vi "SpectrometerSpinCoater_v12.vi"() -> ()   [LabVIEW 2020]
uses:
  TypDef/TabControl_InSitu_Type.ctl
  <instrlib>/Classes/CCD/Abstract_CCD/Abstract_CCD.lvclass
  <instrlib>/Classes/SpinCoater/SpinCoater.lvclass
  TypDef/DeviceQueue_TypeDef.ctl
  TypDef/DeviceQueue_Action.ctl
  TypDef/TabControl.ctl
  TypDef/DataQueue_TypeDef.ctl
  TypDef/DataQueue_Action.ctl
  <vilib>/Utility/error.llb/DialogType.ctl
  <instrlib>/Classes/CCD/Avantes/Avantes.lvclass
  C:/Program Files/National Instruments/LabVIEW 2020/instr.lib/Classes/CCD/Abstract_CCD/Abstract_CCD.lvclass
  <vilib>/Analysis/baseanly.llb/A x Vector.vi
  <vilib>/Analysis/NI_AALBase.lvlib
panel:
  out "x-y":dbl
  in  "Reference\nValue":dbl
  out "WL-Det\nPos":i32
  in  "Motor_ShortStop":bool
  out "UpperWLLimit":i32=713
  out "LowerWLLimit":i32=149
  out "Nr After Spin":u16
  out "Action":string="TimeOut"
  out "Time.spin":refnum<file>
  out "Meas.spin":refnum<file>
  out "Arduino":bool
  out "NKT":bool
  out "Spectromter":bool
  in  "Abort Button":bool
  in  "Stop Button":bool=TRUE
  in  "Tab Control":T1(tab)
  in  "Trim\nSpec":bool=TRUE
  in  "Wl \nUp":dbl[unit]=7.102291259765626e-07
  in  "Wl \nLow":dbl[unit]=3.7998095703125003e-07
  in  "Frames for Ref/Dark":dbl=10000.0
  in  "Shutter Toggle":bool
  in  "Program Spin Coater":T2(array[cluster])=[{"Speed (rpm)"=1500.0, "Time (s)"=10.0, "Acc (rpm/s)"=0.0}]
  in  "Spectra Count":u16
  in  "Measure_MeasureSpectrum":bool
  out "Overall Time":dbl=13.0
  in  "Frames":i32=34211
  in  "StartMeasurement_Button":bool
  in  "Measure_Preview":bool
  out "Measure_Graph":T3(graph) caption="XY Graph"
  in  "Measure_FramesSpectrometer":dbl=200.0 caption="Frames for Spectrometer"
  in  "StartSpin_Button":bool
  in  "Record RefSpec":bool
  in  "Measure:\nRecord_Darkspec":bool
  in  "Measure_Comments":string="Just for testing" caption="Comments"
  in  "Measure_FileName":string="newlineShort" caption="File Name"
  in  "Measure_SavePath":path=path "C:/Users/Cerberus/Desktop/Test/v12Test" caption="Save Path"
  out "Measure_FrameRate":dbl[unit]=2631.5791015625 caption="Frame Rate"
  in  "Measure_IntegrationTime":dbl[unit]=3e-05 caption="Integration Time"
  in  "Tab Control SpinType":T4=enum."Short"
  in  "Seconds after Spin":dbl[unit]=3.0
  in  "Calculate Frames_Normal":bool=TRUE caption="Calculate Frames"
  in  "periodic time":dbl[unit]=2.0
  in  "Duration after":dbl[unit]
  in  "Spin at end":bool
  in  "Seconds to Spin_Normal":dbl[unit]=5.0 caption="Seconds to Spin"
  in  "Threshold":dbl=0.3
  in  "Time Detect":dbl[unit]=2.0
  in  "Seconds to Spin_Short":dbl[unit]=5.0 caption="Seconds to Spin"
  in  "Spin Time":dbl[unit]=2.0
  in  "Calculate Frames_Short":bool=TRUE caption="Calculate Frames"
  in  "Wavelenght Detect":dbl[unit]=6.000000000000001e-07
  out "SS_StepsLeft":dbl
  out "SS_TimePrediction":dbl[unit]=-6.0
  out "Horizontal Progress Bar":u8(slide) scale=0.0..100.0
  in  "SpectralStability:\nRecord_Darkspec":bool
  in  "SpectralStability_Record":bool
  in  "SpectralStability_\nMeasurementNumber":u32 caption="Measurement Number"
  in  "SpectralStability_Duration":dbl[unit] caption="Duration"
  in  "Duration/Times":bool
  in  "SpectralStability_\nPeriodicTime":dbl[unit] caption="Periodic Time"
  in  "SpectralStability_MeasureSpectrum":bool
  in  "SpectralStability_Preview":bool
  out "SpectralStability_Graph":T3(graph) caption="XY Graph"
  in  "SpectralStability_FramesSpectrometer":dbl=200.0 caption="Frames for Spectrometer"
  in  "SpectralStability_Comments":string="Just for testing" caption="Comments"
  in  "SpectralStability_FileName":string="TestingAfter" caption="File Name"
  in  "SpectralStability_SavePath":path=path "C:/Users/Timo/Desktop/Test/180824" caption="Save Path"
  out "SpectralStability_FrameRate":dbl[unit]=2631.5791015625 caption="Frame Rate"
  in  "SpectralStability_IntegrationTime":dbl[unit]=3e-05 caption="Integration Time"
  in  "Shutter Close":bool
  in  "Shutter Open":bool
  in  "SHUTTER DEBUG":bool
  in  "Shutter Position":u16=1000
  in  "Dividider Get Spectra":u32=1 min=1
  in  "Automatically \nadjust count":bool=TRUE
  in  "Reset Count\nafter Spin Coating":bool=TRUE
  in  "ESC_Speed":dbl
  in  "ESC_Milliseconds":dbl
  in  "ESC DEBUG":bool
  in  "Port Arduino":refnum<visa-resource-name>="COM7"
  out "Error Arduino":bool caption="Error"
  in  "Init_Arduino":bool caption="Init"
  out "Caption_Settings_Arduino":string="Arduino"
  out "Caption_Settings_NKT":string="NKT Laser"
  out "Error_Spectromter":bool caption="Error"
  in  "Init_Spectrometer":bool caption="Init"
  out "Caption_Settings_Spectrometer":string="Spectromter"
  # "Speed (rpm)   Time (s)        Acceleration \n                                               (rpm/s)"
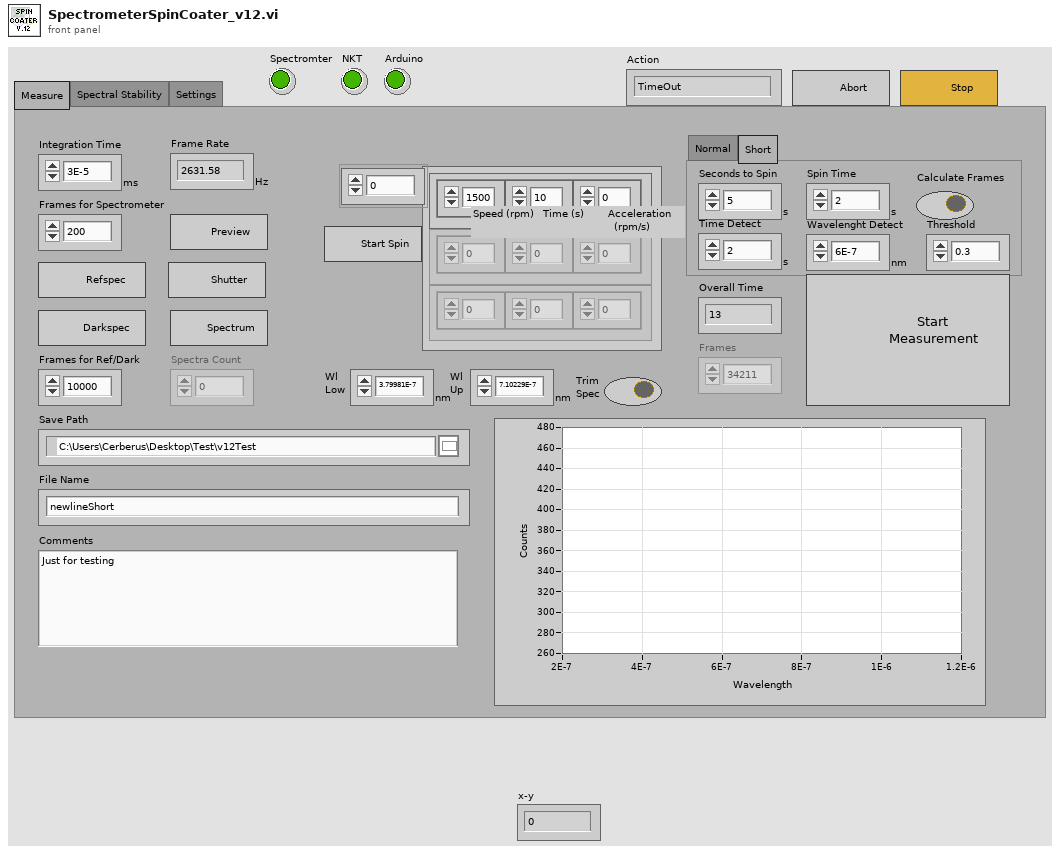
[diagram p1: front panel]
types:
  T1 = enum32{"Measure", "Spectral Stability", "Settings"}
  T2 = cluster{"Speed (rpm)":dbl, "Time (s)":dbl, "Acc (rpm/s)":dbl}[]
  T3 = cluster{"Wavlength":dbl[unit][], "Image":dbl[]}[]
  T4 = typedef "TabControl_InSitu_Type.ctl" = enum32{"Normal", "Short"}
  T5 = cluster{"Dark":cluster{"Image":dbl[][][], "Frame Size":cluster{"F":i32, "Y":i32, "X":i32}}[], "Ref":cluster{"Image":dbl[][][], "Frame Size":cluster{"F":i32, "Y":i32, "X":i32}}[], "Wavlength":dbl[unit][], "Wavlength Trim":dbl[unit][], "spec":dbl[][]}
  T6 = cluster{"Abstract_CCD.lvclass":refnum<class "Abstract_CCD.lvclass">, "SpinCoater.lvclass":refnum<class "SpinCoater.lvclass">}
  T7 = enum8{"Enabled", "Disabled", "Disabled and Grayed Out"}
  T8 = typedef "DataQueue_TypeDef.ctl" = cluster{"QueueAction":T9, "Data":cluster{"Image":dbl[][][], "Frame Size":cluster{"F":i32, "Y":i32, "X":i32}}[], "Data_Raw":cluster{"Image":dbl[][][], "Frame Size":cluster{"F":i32, "Y":i32, "X":i32}}[], "Data_Dark":cluster{"Image":dbl[][][], "Frame Size":cluster{"F":i32, "Y":i32, "X":i32}}[], "Data_Ref":cluster{"Image":dbl[][][], "Frame Size":cluster{"F":i32, "Y":i32, "X":i32}}[], "Device Information":string[], "Numeric Control":dbl, "Boolean":bool, "Wavelength":dbl[unit][], "Time":dbl[], "Time Stamp":timestamp, "Numeric Control 2":dbl, "TabControl":T10, "Numeric Control 3":dbl}
  T9 = typedef "DataQueue_Action.ctl" = enum16{"TimeOut", "Close_Program", "Abort", "Stop_Measurement", "Measure_InSituSpinCoating", "Measure_InSituSpinCoating_Short", "Measure_Spectrum", "Measure_SpectrumAdvanced", "Measure_SpectralStability", "Save_InSitu", "Save_SpectralStability", "Set_Ref", "Set_Dark", "Set_Wavelength", "Spectrometer_Measure", "Spectrometer_Preview", "Transfer_Settings", "Change_TrimSettings"}
  T10 = typedef "TabControl.ctl" = enum16{"Measure", "Spectral Stability", "Settings"}
  T11 = typedef "DeviceQueue_TypeDef.ctl" = cluster{"QueueAction":T12, "Numeric 1":dbl, "Numeric 2":dbl, "Boolean 1":bool, "Boolean 2":bool, "Spin Program":dbl[][], "Spin Prg v07":cluster{"Speed (rpm)":dbl, "Time (s)":dbl, "Acc (rpm/s)":dbl}[], "Time Stamp":timestamp, "TabControl":T10}
  T12 = typedef "DeviceQueue_Action.ctl" = enum16{"TimeOut", "Wait", "Close_Program", "Abort", "Spectrometer_Init", "Spectrometer_Close", "Spectrometer_DeviceInformation", "Spectrometer_Measure", "Spectrometer_MeasureAdvanced", "Spectrometer_Preview", "Spectrometer_Abort", "Spectrometer_StartMeasurement", "Spectrometer_GetData", "Spectrometer_GetData_Short", "Spectrometer_StopMeasurement", "Spectrometer_SetIntegrationTime", "Spectrometer_SetFrames", "Spectrometer_SetDarkspec", "Spectrometer_SetReference", "Spectrometer_SetTriggerMode", "Laser_Init", "Laser_Close", "Arduino_Init", "Arduino_Close", "Arduino_LoadProgram", "Arduino_StartProgram", "Arduino_SetSpeed", "Arduino_SetMillis", "Arduino_StopSpin", "Arduino_ShortStop", "Arduino_Shutter_SetPosition", "Arduino_Shutter_Close", "Arduino_Shutter_Open", "Measure_InSitu", "Measure_Spectrum", "Measure_InSituAdvanced", "Measure_InSituAdvanced_Short", "Measure_SpectralStability", "Measure_Stop"}
  T13 = enum16{"open", "replace", "create", "open or create", "replace or create", "replace or create with confirmation"}
  T14 = cluster{"Image":dbl[][][], "Frame Size":cluster{"F":i32, "Y":i32, "X":i32}}[]
  T15 = cluster{"Image":dbl[][][], "Frame Size":cluster{"F":i32, "Y":i32, "X":i32}}
  T16 = cluster{"Wavlength":dbl[unit][], "A x Vector":dbl[]}
  T17 = cluster{"Wavlength":dbl[unit][], "A x Vector":dbl[]}[]
  T18 = cluster{u16[][][], u16[][][], dbl[], "Numeric Control":dbl, "Numeric Control 2":dbl}
  T19 = typedef "DialogType.ctl" = u16
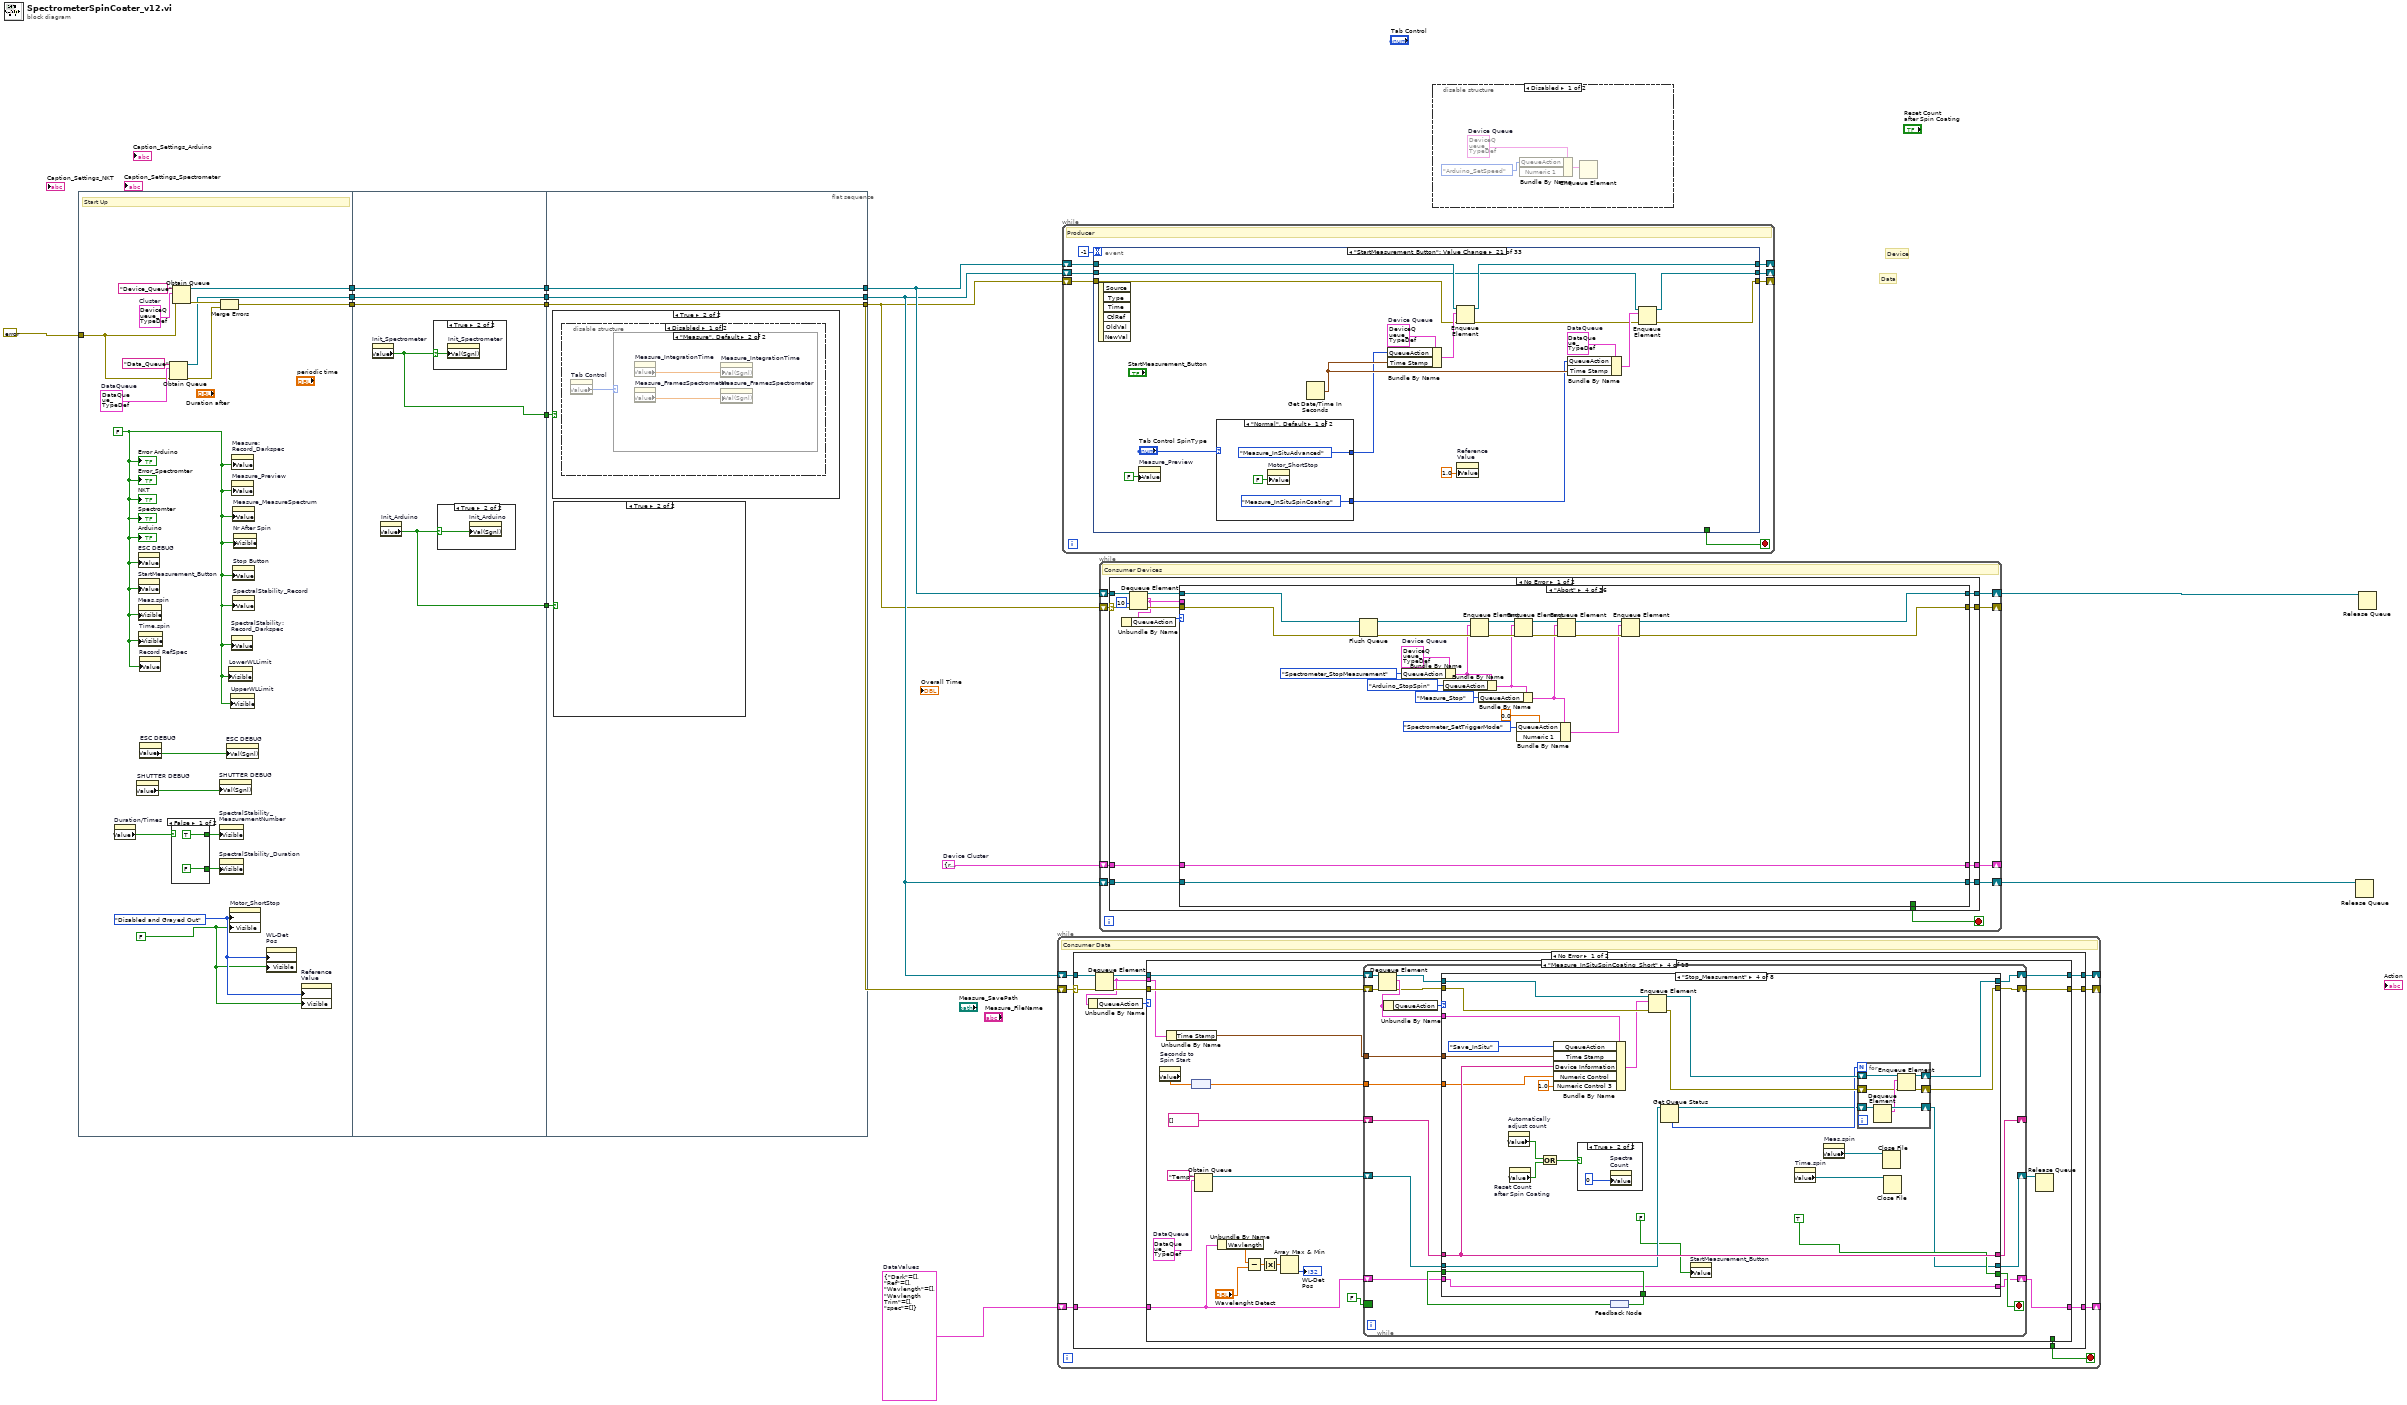
[diagram p0: block diagram]
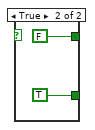
[diagram p3: hidden frame]
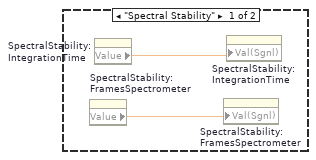
[diagram p8: hidden frame]
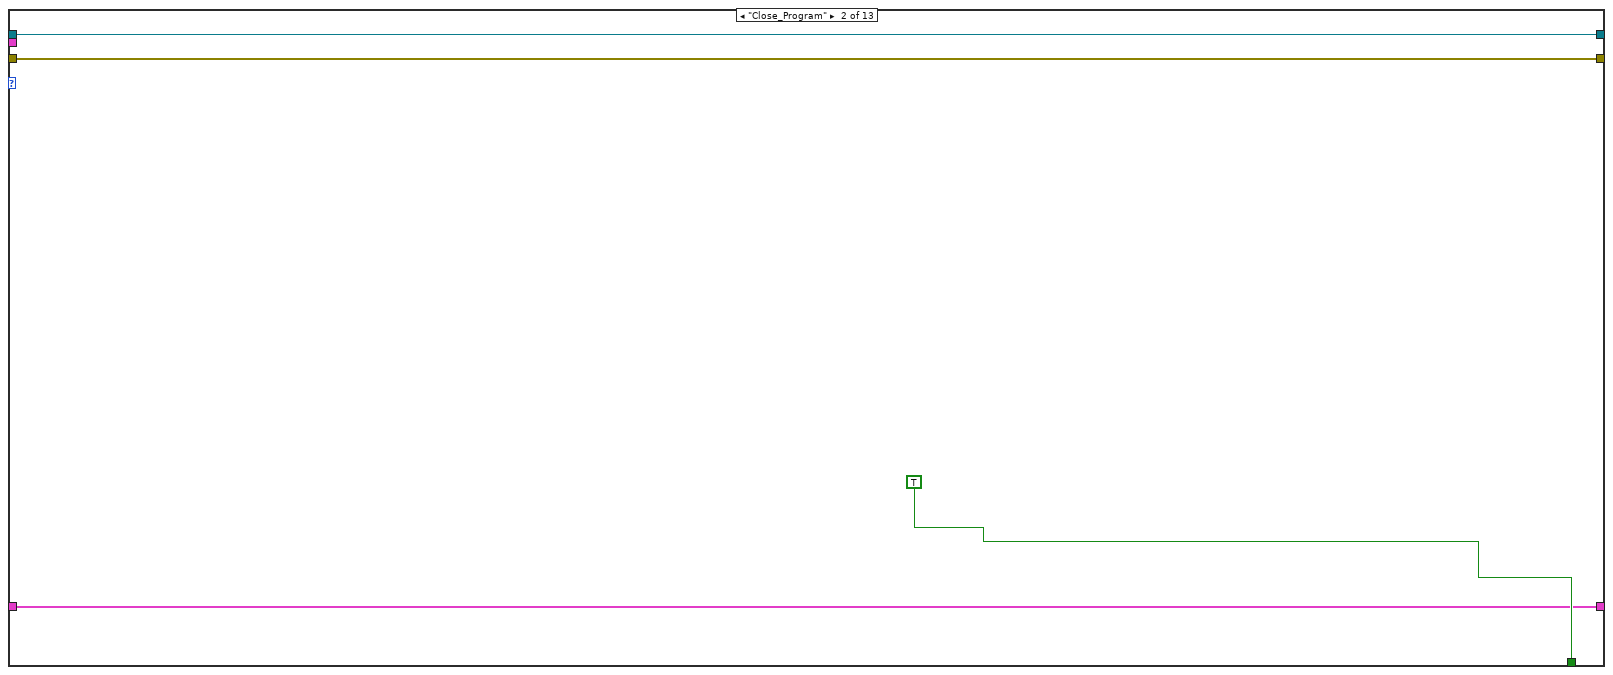
[diagram p11: hidden frame]
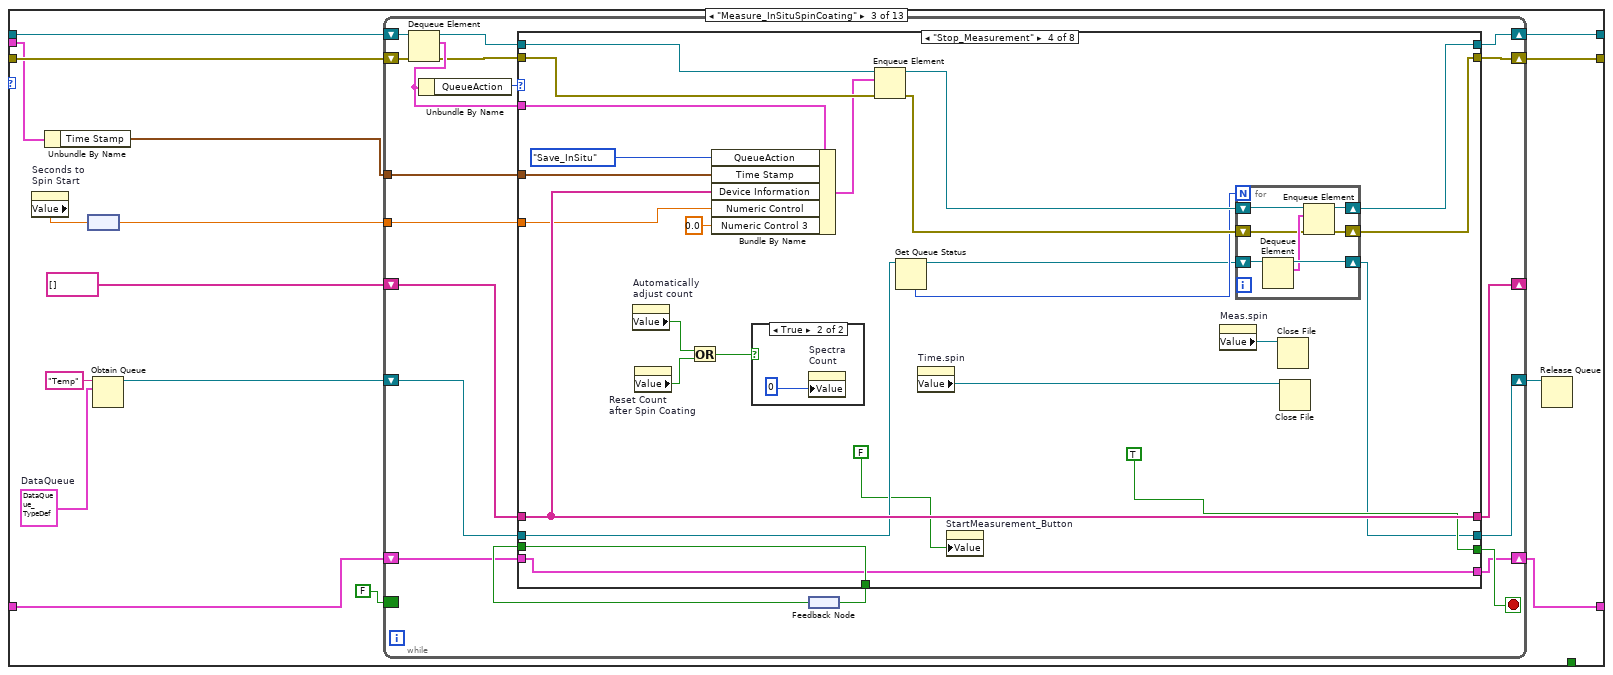
[diagram p12: hidden frame]
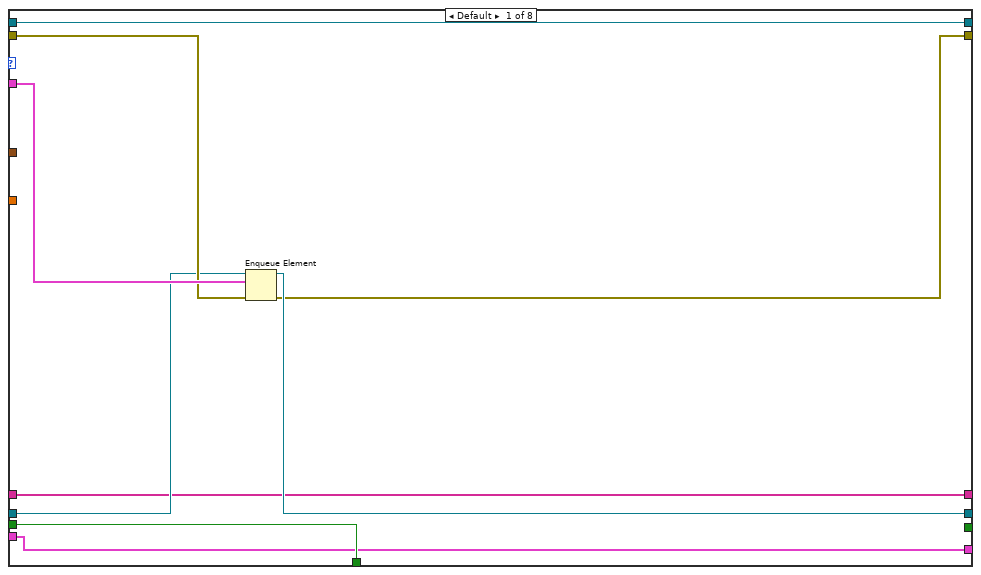
[diagram p13: hidden frame]
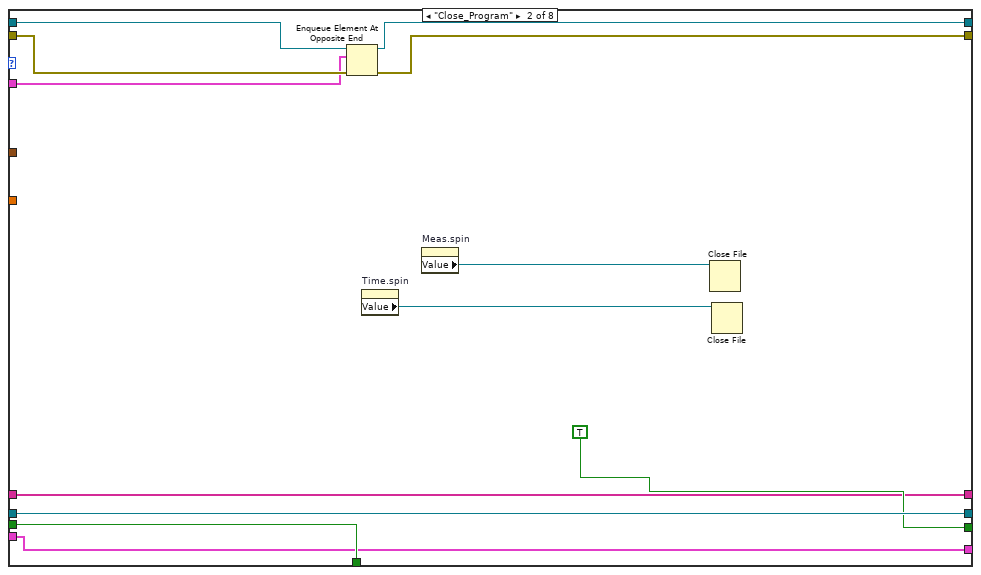
[diagram p14: hidden frame]
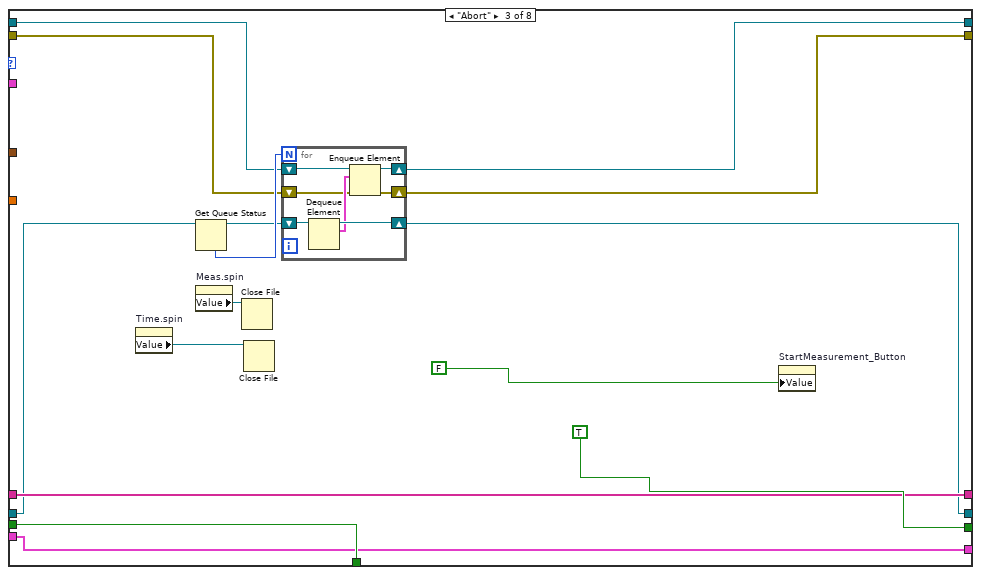
[diagram p15: hidden frame]
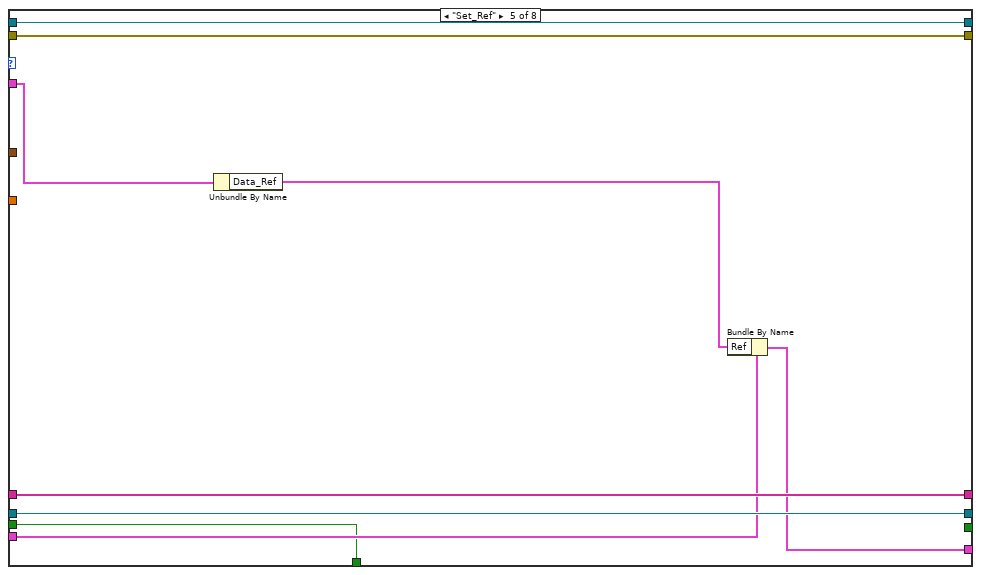
[diagram p17: hidden frame]
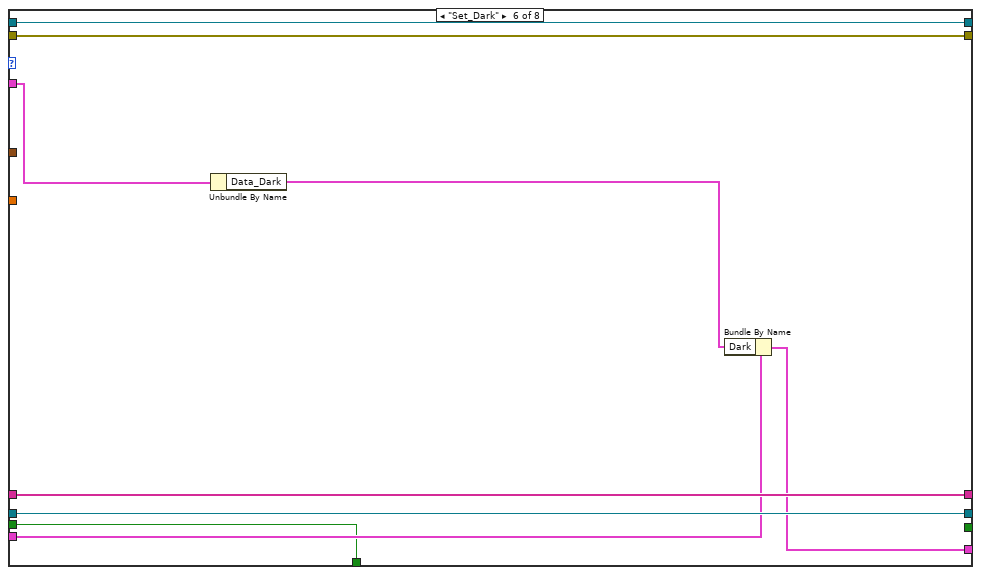
[diagram p18: hidden frame]
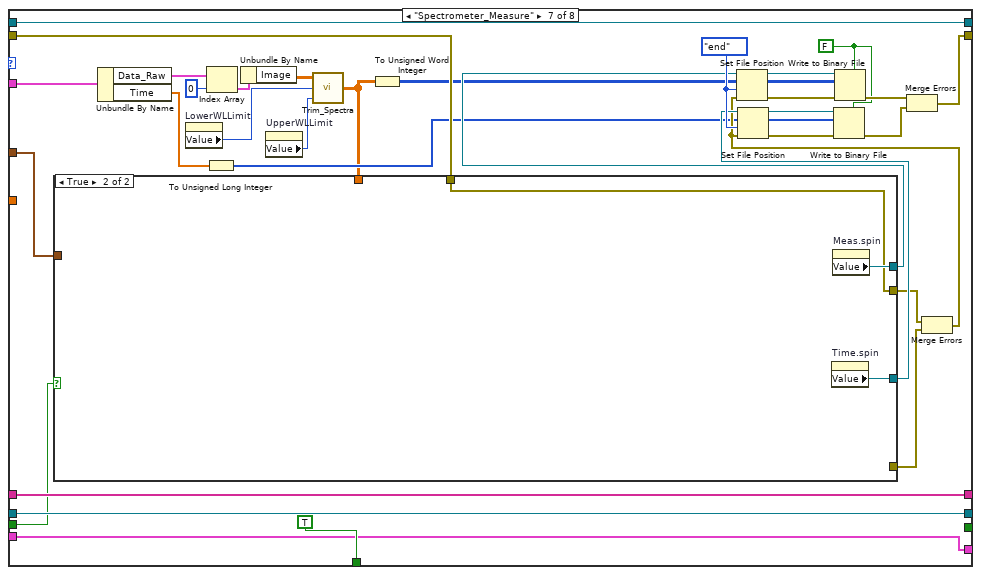
[diagram p19: hidden frame]
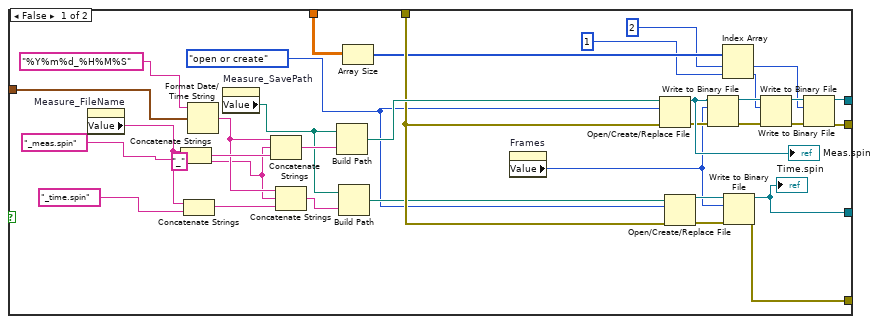
[diagram p20: hidden frame]
diagram:
  w7 = T5 {"Dark"=[], "Ref"=[], "Wavlength"=[], "Wavlength Trim"=[], "spec"=[]}  # DataValues
  w11 = T6 {"Abstract_CCD.lvclass"=refnum, "SpinCoater.lvclass"=refnum}  # Device Cluster
  # "Data"
  # "Device"
  n1 = flat-sequence {
    tunnel: errorcluster {"status"=FALSE, "code"=0, "source"=""} ("error constant") -> [w29]
    tunnel: [w32] -> w15
    tunnel: [w26] -> w14
    tunnel: [w25] -> w13
    tunnel: w15 -> [w43]
    tunnel: w14 -> [w42]
    tunnel: w13 -> [w41]
    tunnel: [w43] -> w6
    tunnel: [w42] -> w5
    tunnel: [w41] -> w4
    tunnel: [w40] -> w3
    tunnel: [w39] -> w2
    tunnel: [w48] -> w1
    tunnel: [w49] -> w8
    tunnel: [w50] -> w12
    tunnel: w6 -> [w50]
    tunnel: w5 -> [w49]
    tunnel: w4 -> [w48]
    tunnel: w3 -> [w47]
    tunnel: w2 -> [w46]
    frame #0 {
      w18 = T7."Disabled and Grayed Out" ("Disabled")
      w17 = FALSE ("Visible")
      w30 = T8 {"QueueAction"=enum."TimeOut", "Data"=[], "Data_Raw"=[], "Data_Dark"=[], "Data_Ref"=[], "Device Information"=[], "Numeric Control"=0.0, "Boolean"=FALSE, "Wavelength"=[], "Time"=[], "Time Stamp"=timestamp(0 s since 1904-01-01), "Numeric Control 2"=0.0, "TabControl"=enum."Measure", "Numeric Control 3"=0.0}  # DataQueue
      w33 = T11 {"QueueAction"=enum."TimeOut", "Numeric 1"=0.0, "Numeric 2"=0.0, "Boolean 1"=FALSE, "Boolean 2"=FALSE, "Spin Program"=[], "Spin Prg v07"=[], "Time Stamp"=timestamp(0 s since 1904-01-01), "TabControl"=enum."Measure"}  # Cluster
      w19 = FALSE ("Error Arduino")
      # "Start Up"
      n2 = property on="Duration/Times" class="Bool (strict)"() -> ("Value"=w21:bool)  [unwired: 2 in, 2 out]
      n3 = property on="SHUTTER DEBUG" class="Bool (strict)"() -> ("Value"=w20:bool)  [unwired: 2 in, 2 out]
      n4 = property on="ESC DEBUG" class="Bool (strict)"("Value"=w19) -> ()  [unwired: 2 in, 2 out]
      n5 = property on="StartMeasurement_Button" class="Bool (strict)"("Value"=w19) -> ()  [unwired: 2 in, 2 out]
      n6 = property on="Meas.spin" class="Ref (strict)"("Visible"=w19) -> ()  [unwired: 2 in, 2 out]
      n7 = property on="Time.spin" class="Ref (strict)"("Visible"=w19) -> ()  [unwired: 2 in, 2 out]
      n8 = property on="Record RefSpec" class="Bool (strict)"("Value"=w19) -> ()  [unwired: 2 in, 2 out]
      n9 = property on="ESC DEBUG" class="Bool (strict)"() -> ("Value"=w24:bool)  [unwired: 2 in, 2 out]
      n10 = Obtain Queue(name (unnamed)="Data_Queue", element data type=w30, error in (no error)=w29) -> (queue out=w26:refnum<queue>, error out=w27:errorcluster)  [unwired: 2 in, 1 out]
      n11 = case shown="False" w21 {
        tunnel: [FALSE TRUE] -> w23
        tunnel: [TRUE FALSE] -> w22
        frame False {
        }
        frame True {
        }
      }
      n12 = Obtain Queue(name (unnamed)="Device_Queue", element data type=w33, error in (no error)=w29) -> (queue out=w32:refnum<queue>, error out=w28:errorcluster)  [unwired: 2 in, 1 out]
      n13 = property on="SHUTTER DEBUG" class="Bool (strict)"("Val(Sgnl)"=w20) -> ()  [unwired: 2 in, 2 out]
      n14 = property on="SpectralStability_\nMeasurementNumber" class="DigNum (strict)"("Visible"=w22) -> ()  [unwired: 2 in, 2 out]
      n15 = property on="SpectralStability_Duration" class="DigNum (strict)"("Visible"=w23) -> ()  [unwired: 2 in, 2 out]
      n16 = Merge Errors(w28, w27) -> (w25:errorcluster)
      n17 = property on="ESC DEBUG" class="Bool (strict)"("Val(Sgnl)"=w24) -> ()  [unwired: 2 in, 2 out]
      n18 = property on="LowerWLLimit" class="DigNum (strict)"("Visible"=w19) -> ()  [unwired: 2 in, 2 out]
      n19 = property on="Motor_ShortStop" class="Bool (strict)"("DisabledEnum"=w18, "Visible"=w17) -> ()  [unwired: 2 in, 2 out]
      n20 = property on="UpperWLLimit" class="DigNum (strict)"("Visible"=w19) -> ()  [unwired: 2 in, 2 out]
      n21 = property on="SpectralStability:\nRecord_Darkspec" class="Bool (strict)"("Value"=w19) -> ()  [unwired: 2 in, 2 out]
      n22 = property on="Measure:\nRecord_Darkspec" class="Bool (strict)"("Value"=w19) -> ()  [unwired: 2 in, 2 out]
      n23 = property on="Measure_Preview" class="Bool (strict)"("Value"=w19) -> ()  [unwired: 2 in, 2 out]
      n24 = property on="Measure_MeasureSpectrum" class="Bool (strict)"("Value"=w19) -> ()  [unwired: 2 in, 2 out]
      n25 = property on="Stop Button" class="Bool (strict)"("Value"=w19) -> ()  [unwired: 2 in, 2 out]
      n26 = property on="SpectralStability_Record" class="Bool (strict)"("Value"=w19) -> ()  [unwired: 2 in, 2 out]
      n27 = property on="Nr After Spin" class="DigNum (strict)"("Visible"=w19) -> ()  [unwired: 2 in, 2 out]
      n28 = property on="WL-Det\nPos" class="DigNum (strict)"("DisabledEnum"=w18, "Visible"=w17) -> ()  [unwired: 2 in, 2 out]
      n29 = property on="Reference\nValue" class="DigNum (strict)"("DisabledEnum"=w18, "Visible"=w17) -> ()  [unwired: 2 in, 2 out]
      "Error_Spectromter" <- w19
      "Error Arduino" <- w19
      "Spectromter" <- w19
      "NKT" <- w19
      "Arduino" <- w19
    }
    frame #1 {
      n30 = property on="Init_Spectrometer" class="Bool (strict)"() -> ("Value"=w40:bool)  [unwired: 2 in, 2 out]
      n31 = property on="Init_Arduino" class="Bool (strict)"() -> ("Value"=w39:bool)  [unwired: 2 in, 2 out]
      n32 = case shown="True" w40 {
        selector: w40 -> [_ w45]
        frame False {
        }
        frame True {
          n33 = property on="Init_Spectrometer" class="Bool (strict)"("Val(Sgnl)"=w45) -> ()  [unwired: 2 in, 2 out]
        }
      }
      n34 = case shown="True" w39 {
        selector: w39 -> [_ w44]
        frame False {
        }
        frame True {
          n35 = property on="Init_Arduino" class="Bool (strict)"("Val(Sgnl)"=w44) -> ()  [unwired: 2 in, 2 out]
        }
      }
    }
    frame #2 {
      n36 = case shown="True" w47 {
        frame False {
        }
        frame True {
          n37 = disable-structure shown="Disabled" {
            frame Disabled {
              n38 = property on="Tab Control" class="TabCtl (strict)"() -> ("Value"=w51:T1)  [unwired: 2 in, 2 out]
              n39 = case shown="\"Measure\", Default" w51 {
                frame "Spectral Stability" {
                  n40 = property on="SpectralStability:\nFramesSpectrometer" class="DigNum (strict)"() -> ("Value"=w52:dbl)  [unwired: 2 in, 2 out]
                  n41 = property on="SpectralStability:\nIntegrationTime" class="DigNum (strict)"() -> ("Value"=w53:dbl[unit])  [unwired: 2 in, 2 out]
                  n42 = property on="SpectralStability:\nFramesSpectrometer" class="DigNum (strict)"("Val(Sgnl)"=w52) -> ()  [unwired: 2 in, 2 out]
                  n43 = property on="SpectralStability:\nIntegrationTime" class="DigNum (strict)"("Val(Sgnl)"=w53) -> ()  [unwired: 2 in, 2 out]
                }
                frame "Measure", Default {
                  n44 = property on="Measure_IntegrationTime" class="DigNum (strict)"() -> ("Value"=w54:dbl[unit])  [unwired: 2 in, 2 out]
                  n45 = property on="Measure_FramesSpectrometer" class="DigNum (strict)"() -> ("Value"=w55:dbl)  [unwired: 2 in, 2 out]
                  n46 = property on="Measure_IntegrationTime" class="DigNum (strict)"("Val(Sgnl)"=w54) -> ()  [unwired: 2 in, 2 out]
                  n47 = property on="Measure_FramesSpectrometer" class="DigNum (strict)"("Val(Sgnl)"=w55) -> ()  [unwired: 2 in, 2 out]
                }
              }
            }
            frame Enabled {
            }
          }
        }
      }
      n48 = case shown="True" w46 {
        frame False {
        }
        frame True {
        }
      }
    }
  }
  n49 = while {
    shift-right: [w56] -> _
    shift-left: w1 -> [w62]
    shift-right: [w57] -> _
    shift-left: w8 -> [w61]
    shift-right: [w58] -> _
    shift-left: w7 -> [w60]
    stop <- w59 stop-if-true
    # "Consumer Data"
    n50 = case shown="No Error" w62 {
      selector: w62 -> [w73 w1049]
      tunnel: w61 -> [w72 w1050]
      tunnel: w60 -> [w70 w1047]
      tunnel: [w69 _] -> w59
      tunnel: [w68 w1047] -> w58
      tunnel: [w67 w1050] -> w57
      tunnel: [w65 w1048] -> w56
      frame No Error {
        n51 = Dequeue Element(queue=w72, error in (no error)=w73) -> (queue out=w66:refnum<queue>, element=w63:T8, error out=w64:errorcluster)  [unwired: 1 in, 1 out]
        n52 = Unbundle By Name(w63) -> ("QueueAction"=w71:T9)
        n53 = case shown="\"Measure_InSituSpinCoating_Short\"" w71 {
          tunnel: w70 -> [w74 w79 w81 w294 w502 w607 w709 w928 w965 w974 w997 w1010 w1017]
          tunnel: [_ TRUE _ _ _ _ _ _ _ _ _ _ _] -> w69
          tunnel: [w74 w79 w83 w296 w502 w607 w700 w928 w969 w988 w996 w1010 w1016] -> w68
          tunnel: [w76 w78 w96 w309 w508 w613 w693 w950 w970 w989 w993 w1012 w1023] -> w67
          tunnel: w66 -> [w76 w78 w94 w307 w509 w614 w704 w950 w970 w989 w993 w1012 w1023]
          tunnel: [w75 w77 w95 w308 w507 w612 w694 w949 w971 w990 w994 w1011 w1020] -> w65
          tunnel: w64 -> [w75 w77 w93 w306 w510 w615 w703 w949 w971 w990 w994 w1011 w1020]
          tunnel: w63 -> [_ _ w88 w301 _ _ w696 w940 w972 w991 w995 w1001 w1022]
          frame "TimeOut", Default {
          }
          frame "Close_Program" {
          }
          frame "Measure_InSituSpinCoating" {
            w91 = T8 {"QueueAction"=enum."TimeOut", "Data"=[], "Data_Raw"=[], "Data_Dark"=[], "Data_Ref"=[], "Device Information"=[], "Numeric Control"=0.0, "Boolean"=FALSE, "Wavelength"=[], "Time"=[], "Time Stamp"=timestamp(0 s since 1904-01-01), "Numeric Control 2"=0.0, "TabControl"=enum."Measure", "Numeric Control 3"=0.0}  # DataQueue
            n54 = property on="Seconds to\nSpin Start" class="DigNum (strict)"() -> ("Value"=w85:dbl[unit])  [unwired: 2 in, 2 out]
            n55 = Unbundle By Name(w88) -> ("Time Stamp"=w87:timestamp)
            n56 = node(w85) -> (w84:dbl)
            n57 = Obtain Queue(name (unnamed)="Temp", element data type=w91) -> (queue out=w90:refnum<queue>)  [unwired: 3 in, 2 out]
            n58 = while {
              shift-right: [w106] -> w96
              shift-left: w94 -> [w115]
              shift-right: [w107] -> w95
              shift-left: w93 -> [w114]
              shift-right: [w108] -> w89
              shift-left: w90 -> [w109]
              tunnel: w87 -> [w102]
              shift-right: [w103] -> _
              shift-left: string[] [] ("Device Information") -> [w104]
              border: FALSE -> [_]
              tunnel: w84 -> [w99]
              shift-right: [w97] -> w83
              shift-left: w81 -> [w98]
              stop <- w105 stop-if-true
              n59 = Dequeue Element(queue=w115, error in (no error)=w114) -> (queue out=w110:refnum<queue>, element=w112:T8, error out=w111:errorcluster)  [unwired: 1 in, 1 out]
              n60 = Unbundle By Name(w112) -> ("QueueAction"=w113:T9)
              n61 = feedback #1() -> (w101:bool)
              n62 = case shown="\"Stop_Measurement\"" w113 {
                tunnel: w112 -> [w124 w134 _ w183 w201 w210 w242 w287]
                tunnel: w111 -> [w123 w135 w142 w180 w199 w208 w233 w284]
                tunnel: w110 -> [w119 w136 w141 w179 w200 w209 w241 w285]
                tunnel: w109 -> [w122 w131 w143 w174 w197 w206 w230 w288]
                tunnel: [w121 w131 w138 w171 w197 w206 w230 w288] -> w108
                tunnel: [w120 w132 w140 w170 w199 w208 w231 w284] -> w107
                tunnel: [w119 w133 w139 w169 w200 w209 w241 w285] -> w106
                tunnel: [_ TRUE TRUE TRUE _ _ _ _] -> w105
                tunnel: w104 -> [w118 w129 w150 w181 w198 w207 w228 _]
                tunnel: [w118 w129 w150 w181 w198 w207 w228 w286] -> w103
                tunnel: w102 -> [_ _ _ w182 _ _ w243 _]
                tunnel: w101 -> [w117 w128 w149 w168 w193 w202 w226 w283]
                tunnel: [w117 w128 w149 w168 w193 w202 TRUE w283] -> w100
                tunnel: w99 -> [_ _ _ w165 _ _ _ _]
                tunnel: w98 -> [w116 w125 w137 w160 w196 w205 w211 w282]
                tunnel: [w116 w125 w137 w160 w194 w203 w211 w282] -> w97
                frame Default {
                  n63 = Enqueue Element(queue=w122, element=w124, error in (no error)=w123) -> (queue out=w121:refnum<queue>, error out=w120:errorcluster)  [unwired: 1 in, 1 out]
                }
                frame "Close_Program" {
                  n64 = Enqueue Element At Opposite End(queue=w136, element=w134, error in (no error)=w135) -> (queue out=w133:refnum<queue>, error out=w132:errorcluster)  [unwired: 1 in, 1 out]
                  n65 = property on="Time.spin" class="Ref (strict)"() -> ("Value"=w126:refnum<file>)  [unwired: 2 in, 2 out]
                  n66 = property on="Meas.spin" class="Ref (strict)"() -> ("Value"=w127:refnum<file>)  [unwired: 2 in, 2 out]
                  n67 = Close File(refnum=w127) -> ()  [unwired: 1 in, 2 out]
                  n68 = Close File(refnum=w126) -> ()  [unwired: 1 in, 2 out]
                }
                frame "Abort" {
                  n69 = property on="Time.spin" class="Ref (strict)"() -> ("Value"=w147:refnum<file>)  [unwired: 2 in, 2 out]
                  n70 = Get Queue Status(queue=w143) -> (queue out=w144:refnum<queue>, # elements in queue=w145:i32)  [unwired: 2 in, 6 out]
                  n71 = property on="Meas.spin" class="Ref (strict)"() -> ("Value"=w148:refnum<file>)  [unwired: 2 in, 2 out]
                  n72 = Close File(refnum=w148) -> ()  [unwired: 1 in, 2 out]
                  n73 = Close File(refnum=w147) -> ()  [unwired: 1 in, 2 out]
                  n74 = for {
                    N: w145 -> [_]
                    shift-right: [w157] -> w138
                    shift-left: w144 -> [w158]
                    shift-right: [w154] -> w139
                    shift-left: w141 -> [w155]
                    shift-right: [w152] -> w140
                    shift-left: w142 -> [w153]
                    n75 = Dequeue Element(queue=w158) -> (queue out=w157:refnum<queue>, element=w156:T8)  [unwired: 2 in, 2 out]
                    n76 = Enqueue Element(queue=w155, element=w156, error in (no error)=w153) -> (queue out=w154:refnum<queue>, error out=w152:errorcluster)  [unwired: 1 in, 1 out]
                  }
                  n77 = property on="StartMeasurement_Button" class="Bool (strict)"("Value"=FALSE ("StartMeasurement_Button")) -> ()  [unwired: 2 in, 2 out]
                }
                frame "Stop_Measurement" {
                  n78 = property on="Automatically \nadjust count" class="Bool (strict)"() -> ("Value"=w162:bool)  [unwired: 2 in, 2 out]
                  n79 = property on="Reset Count\nafter Spin Coating" class="Bool (strict)"() -> ("Value"=w163:bool)  [unwired: 2 in, 2 out]
                  n80 = Or(x=w162, y=w163) -> (x .or. y?=w161:bool)
                  n81 = Bundle By Name(cluster=w183, "QueueAction"=DataQueue_Action."Save_InSitu", "Time Stamp"=w182, "Device Information"=w181, "Numeric Control"=w165, "Numeric Control 3"=0.0) -> (w178:T8)
                  n82 = case shown="True" w161 {
                    frame False {
                    }
                    frame True {
                      n83 = property on="Spectra \nCount" class="DigNum (strict)"("Value"=u16 0 ("Spectra Count")) -> ()  [unwired: 2 in, 2 out]
                    }
                  }
                  n84 = Enqueue Element(queue=w179, element=w178, error in (no error)=w180) -> (queue out=w176:refnum<queue>, error out=w175:errorcluster)  [unwired: 1 in, 1 out]
                  n85 = Get Queue Status(queue=w174) -> (queue out=w172:refnum<queue>, # elements in queue=w173:i32)  [unwired: 2 in, 6 out]
                  n86 = property on="Time.spin" class="Ref (strict)"() -> ("Value"=w166:refnum<file>)  [unwired: 2 in, 2 out]
                  n87 = property on="StartMeasurement_Button" class="Bool (strict)"("Value"=FALSE ("StartMeasurement_Button")) -> ()  [unwired: 2 in, 2 out]
                  n88 = property on="Meas.spin" class="Ref (strict)"() -> ("Value"=w167:refnum<file>)  [unwired: 2 in, 2 out]
                  n89 = for {
                    N: w173 -> [_]
                    shift-right: [w191] -> w171
                    shift-left: w172 -> [w192]
                    shift-right: [w188] -> w169
                    shift-left: w176 -> [w189]
                    shift-right: [w186] -> w170
                    shift-left: w175 -> [w187]
                    n90 = Dequeue Element(queue=w192) -> (queue out=w191:refnum<queue>, element=w190:T8)  [unwired: 2 in, 2 out]
                    n91 = Enqueue Element(queue=w189, element=w190, error in (no error)=w187) -> (queue out=w188:refnum<queue>, error out=w186:errorcluster)  [unwired: 1 in, 1 out]
                  }
                  n92 = Close File(refnum=w167) -> ()  [unwired: 1 in, 2 out]
                  n93 = Close File(refnum=w166) -> ()  [unwired: 1 in, 2 out]
                }
                frame "Set_Ref" {
                  n94 = Unbundle By Name(w201) -> ("Data_Ref"=w195:T14)
                  n95 = Bundle By Name(cluster=w196, "Ref"=w195) -> (w194:T5)
                }
                frame "Set_Dark" {
                  n96 = Unbundle By Name(w210) -> ("Data_Dark"=w204:T14)
                  n97 = Bundle By Name(cluster=w205, "Dark"=w204) -> (w203:T5)
                }
                frame "Spectrometer_Measure" {
                  w216 = FALSE ("prepend array or string size? (T)")
                  w229 = enum16{"start", "end", "current"}."end" ("from (0:start)")
                  n98 = Unbundle By Name(w242) -> ("Data_Raw"=w238:T14, "Time"=w232:dbl[])
                  n99 = property on="LowerWLLimit" class="DigNum (strict)"() -> ("Value"=w213:i32)  [unwired: 2 in, 2 out]
                  n100 = To Unsigned Long Integer(number=w232) -> (unsigned 32bit integer=w218:u32[])
                  n101 = Index Array(array=w238, index=0) -> (element=w237:T15)
                  n102 = Unbundle By Name(w237) -> ("Image"=w215:dbl[][][])
                  n103 = property on="UpperWLLimit" class="DigNum (strict)"() -> ("Value"=w212:i32)  [unwired: 2 in, 2 out]
                  n104 = call "Trim_Spectra.vi"("WL_UpperIndex"=w212, "WL_LowerIndex"=w213, "Image"=w215) -> ("ImageCut"=w214:dbl[][][])
                  n105 = case shown="True" w226 {
                    tunnel: w243 -> [w275 _]
                    tunnel: w233 -> [w270 w279]
                    tunnel: [w256 w279] -> w220
                    tunnel: [w244 _] -> w221
                    tunnel: [w255 w281] -> w223
                    tunnel: [w245 w280] -> w222
                    tunnel: w214 -> [w253 _]
                    frame False {
                      w265 = T13."open or create" ("operation (0:open)")
                      w264 = "_" ("string")
                      n106 = property on="Measure_FileName" class="Str"() -> ("Value"=w273:string)  [unwired: 2 in, 2 out]
                      n107 = Concatenate Strings(w273, "_meas.spin" ("string")) -> (w276:string)
                      n108 = Concatenate Strings(w273, "_time.spin" ("string")) -> (w268:string)
                      n109 = Format Date/Time String(time format string (%c)="%Y%m%d_%H%M%S", seconds (now)=w275) -> (date/time string=w269:string)  [unwired: 1 in]
                      n110 = property on="Measure_SavePath" class="Path"() -> ("Value"=w247:path)  [unwired: 2 in, 2 out]
                      n111 = Concatenate Strings(w269, w264, w276) -> (w274:string)
                      n112 = Concatenate Strings(w269, w264, w268) -> (w267:string)
                      n113 = Build Path(base path=w247, name or relative path=w274) -> (appended path=w271:path)
                      n114 = Build Path(base path=w247, name or relative path=w267) -> (appended path=w266:path)
                      n115 = Array Size(array=w253) -> (size(s)=w252:i32[])
                      n116 = property on="Frames" class="DigNum (strict)"() -> ("Value"=w246:i32)  [unwired: 2 in, 2 out]
                      n117 = Open/Create/Replace File(file path (use dialog)=w271, error in=w270, operation (0:open)=w265) -> (refnum out=w263:refnum<file>, error out=w262:errorcluster)  [unwired: 3 in, 1 out]
                      "Meas.spin" <- w263
                      n118 = Open/Create/Replace File(file path (use dialog)=w266, error in=w270, operation (0:open)=w265) -> (refnum out=w261:refnum<file>, error out=w260:errorcluster)  [unwired: 3 in, 1 out]
                      n119 = Write to Binary File(file (use dialog)=w263, data=w246, error in=w262) -> (refnum out=w259:refnum<file>, error out=w258:errorcluster)  [unwired: 3 in, 1 out]
                      n120 = Index Array(array=w252, index #1=2 ("index"), index #2=1 ("index")) -> (element #1=w248:i32, element #2=w249:i32)
                      n121 = Write to Binary File(file (use dialog)=w261, data=w246, error in=w260) -> (refnum out=w245:refnum<file>, error out=w244:errorcluster)  [unwired: 3 in, 1 out]
                      "Time.spin" <- w245
                      n122 = Write to Binary File(file (use dialog)=w259, data=w249, error in=w258) -> (refnum out=w254:refnum<file>, error out=w257:errorcluster)  [unwired: 3 in, 1 out]
                      n123 = Write to Binary File(file (use dialog)=w254, data=w248, error in=w257) -> (refnum out=w255:refnum<file>, error out=w256:errorcluster)  [unwired: 3 in, 1 out]
                    }
                    frame True {
                      n124 = property on="Time.spin" class="Ref (strict)"() -> ("Value"=w280:refnum<file>)  [unwired: 2 in, 2 out]
                      n125 = property on="Meas.spin" class="Ref (strict)"() -> ("Value"=w281:refnum<file>)  [unwired: 2 in, 2 out]
                    }
                  }
                  n126 = To Unsigned Word Integer(number=w214) -> (unsigned 16bit integer=w217:u16[][][])
                  n127 = Merge Errors(w220, w221) -> (w219:errorcluster)
                  n128 = Set File Position(refnum=w223, from (0:start)=w229, error in=w219) -> (refnum out=w235:refnum<file>, error out=w234:errorcluster)  [unwired: 1 in]
                  n129 = Set File Position(refnum=w222, from (0:start)=w229, error in=w219) -> (refnum out=w240:refnum<file>, error out=w239:errorcluster)  [unwired: 1 in]
                  n130 = Write to Binary File(file (use dialog)=w240, data=w218, error in=w239, 5:w216) -> (error out=w224:errorcluster)  [unwired: 2 in, 2 out]
                  n131 = Write to Binary File(file (use dialog)=w235, data=w217, error in=w234, 5:w216) -> (error out=w225:errorcluster)  [unwired: 2 in, 2 out]
                  n132 = Merge Errors(w225, w224) -> (w231:errorcluster)
                }
                frame "Transfer_Settings" {
                  n133 = Unbundle By Name(w287) -> ("Device Information"=w286:string[])
                }
              }
              n134 = feedback-in #1(w100) -> ()
            }
            n135 = Release Queue(queue=w89) -> ()  [unwired: 2 in, 3 out]
          }
          frame "Measure_InSituSpinCoating_Short" {
            w304 = T8 {"QueueAction"=enum."TimeOut", "Data"=[], "Data_Raw"=[], "Data_Dark"=[], "Data_Ref"=[], "Device Information"=[], "Numeric Control"=0.0, "Boolean"=FALSE, "Wavelength"=[], "Time"=[], "Time Stamp"=timestamp(0 s since 1904-01-01), "Numeric Control 2"=0.0, "TabControl"=enum."Measure", "Numeric Control 3"=0.0}  # DataQueue
            n136 = property on="Seconds to\nSpin Start" class="DigNum (strict)"() -> ("Value"=w298:dbl[unit])  [unwired: 2 in, 2 out]
            n137 = Unbundle By Name(w301) -> ("Time Stamp"=w300:timestamp)
            n138 = node(w298) -> (w297:dbl)
            n139 = Obtain Queue(name (unnamed)="Temp", element data type=w304) -> (queue out=w303:refnum<queue>)  [unwired: 3 in, 2 out]
            n140 = Unbundle By Name(w294) -> ("Wavlength"=w292:dbl[unit][])
            n141 = Subtract(x=w292, y="Wavelenght Detect") -> (x-y=w293:dbl[unit][])
            n142 = Absolute Value(x=w293) -> (abs(x)=w291:dbl[unit][])
            n143 = Array Max & Min(array=w291) -> (min index (indices)=→"WL-Det\nPos":i32)  [unwired: 3 out]
            n144 = while {
              shift-right: [w319] -> w309
              shift-left: w307 -> [w328]
              shift-right: [w320] -> w308
              shift-left: w306 -> [w327]
              shift-right: [w321] -> w302
              shift-left: w303 -> [w322]
              tunnel: w300 -> [w315]
              shift-right: [w316] -> _
              shift-left: string[] [] ("Device Information") -> [w317]
              border: FALSE -> [_]
              tunnel: w297 -> [w312]
              shift-right: [w310] -> w296
              shift-left: w294 -> [w311]
              stop <- w318 stop-if-true
              n145 = Dequeue Element(queue=w328, error in (no error)=w327) -> (queue out=w323:refnum<queue>, element=w325:T8, error out=w324:errorcluster)  [unwired: 1 in, 1 out]
              n146 = Unbundle By Name(w325) -> ("QueueAction"=w326:T9)
              n147 = feedback #2() -> (w314:bool)
              n148 = case shown="\"Stop_Measurement\"" w326 {
                tunnel: w325 -> [w337 w347 _ w396 w414 w423 w455 w500]
                tunnel: w324 -> [w336 w348 w357 w393 w412 w421 w446 w497]
                tunnel: w323 -> [w332 w349 w356 w392 w413 w422 w454 w498]
                tunnel: w322 -> [w335 w344 w358 w387 w410 w419 w443 w501]
                tunnel: [w334 w344 w353 w384 w410 w419 w443 w501] -> w321
                tunnel: [w333 w345 w355 w383 w412 w421 w444 w497] -> w320
                tunnel: [w332 w346 w354 w382 w413 w422 w454 w498] -> w319
                tunnel: [_ TRUE TRUE TRUE _ _ _ _] -> w318
                tunnel: w317 -> [w331 w342 w363 w394 w411 w420 w441 _]
                tunnel: [w331 w342 w363 w394 w411 w420 w441 w499] -> w316
                tunnel: w315 -> [_ _ _ w395 _ _ w456 _]
                tunnel: w314 -> [w330 w341 w362 w381 w406 w415 w439 w496]
                tunnel: [w330 w341 w362 w381 w406 w415 TRUE w496] -> w313
                tunnel: w312 -> [_ _ _ w380 _ _ _ _]
                tunnel: w311 -> [w329 w340 w352 w375 w409 w418 w424 w495]
                tunnel: [w329 w340 w352 w375 w407 w416 w424 w495] -> w310
                frame Default {
                  n149 = Enqueue Element(queue=w335, element=w337, error in (no error)=w336) -> (queue out=w334:refnum<queue>, error out=w333:errorcluster)  [unwired: 1 in, 1 out]
                }
                frame "Close_Program" {
                  n150 = property on="Meas.spin" class="Ref (strict)"() -> ("Value"=w339:refnum<file>)  [unwired: 2 in, 2 out]
                  n151 = property on="Time.spin" class="Ref (strict)"() -> ("Value"=w338:refnum<file>)  [unwired: 2 in, 2 out]
                  n152 = Enqueue Element At Opposite End(queue=w349, element=w347, error in (no error)=w348) -> (queue out=w346:refnum<queue>, error out=w345:errorcluster)  [unwired: 1 in, 1 out]
                  n153 = Close File(refnum=w339) -> ()  [unwired: 1 in, 2 out]
                  n154 = Close File(refnum=w338) -> ()  [unwired: 1 in, 2 out]
                }
                frame "Abort" {
                  n155 = property on="Time.spin" class="Ref (strict)"() -> ("Value"=w350:refnum<file>)  [unwired: 2 in, 2 out]
                  n156 = property on="Meas.spin" class="Ref (strict)"() -> ("Value"=w351:refnum<file>)  [unwired: 2 in, 2 out]
                  n157 = Get Queue Status(queue=w358) -> (queue out=w359:refnum<queue>, # elements in queue=w360:i32)  [unwired: 2 in, 6 out]
                  n158 = Close File(refnum=w351) -> ()  [unwired: 1 in, 2 out]
                  n159 = Close File(refnum=w350) -> ()  [unwired: 1 in, 2 out]
                  n160 = for {
                    N: w360 -> [_]
                    shift-right: [w370] -> w353
                    shift-left: w359 -> [w371]
                    shift-right: [w367] -> w354
                    shift-left: w356 -> [w368]
                    shift-right: [w365] -> w355
                    shift-left: w357 -> [w366]
                    n161 = Dequeue Element(queue=w371) -> (queue out=w370:refnum<queue>, element=w369:T8)  [unwired: 2 in, 2 out]
                    n162 = Enqueue Element(queue=w368, element=w369, error in (no error)=w366) -> (queue out=w367:refnum<queue>, error out=w365:errorcluster)  [unwired: 1 in, 1 out]
                  }
                  n163 = property on="StartMeasurement_Button" class="Bool (strict)"("Value"=FALSE ("StartMeasurement_Button")) -> ()  [unwired: 2 in, 2 out]
                }
                frame "Stop_Measurement" {
                  n164 = property on="Automatically \nadjust count" class="Bool (strict)"() -> ("Value"=w377:bool)  [unwired: 2 in, 2 out]
                  n165 = property on="Reset Count\nafter Spin Coating" class="Bool (strict)"() -> ("Value"=w378:bool)  [unwired: 2 in, 2 out]
                  n166 = Or(x=w377, y=w378) -> (x .or. y?=w376:bool)
                  n167 = Bundle By Name(cluster=w396, "QueueAction"=DataQueue_Action."Save_InSitu", "Time Stamp"=w395, "Device Information"=w394, "Numeric Control"=w380, "Numeric Control 3"=1.0) -> (w391:T8)
                  n168 = case shown="True" w376 {
                    frame False {
                    }
                    frame True {
                      n169 = property on="Spectra \nCount" class="DigNum (strict)"("Value"=u16 0 ("Spectra Count")) -> ()  [unwired: 2 in, 2 out]
                    }
                  }
                  n170 = Enqueue Element(queue=w392, element=w391, error in (no error)=w393) -> (queue out=w389:refnum<queue>, error out=w388:errorcluster)  [unwired: 1 in, 1 out]
                  n171 = Get Queue Status(queue=w387) -> (queue out=w385:refnum<queue>, # elements in queue=w386:i32)  [unwired: 2 in, 6 out]
                  n172 = property on="StartMeasurement_Button" class="Bool (strict)"("Value"=FALSE ("StartMeasurement_Button")) -> ()  [unwired: 2 in, 2 out]
                  n173 = property on="Time.spin" class="Ref (strict)"() -> ("Value"=w373:refnum<file>)  [unwired: 2 in, 2 out]
                  n174 = property on="Meas.spin" class="Ref (strict)"() -> ("Value"=w374:refnum<file>)  [unwired: 2 in, 2 out]
                  n175 = for {
                    N: w386 -> [_]
                    shift-right: [w404] -> w384
                    shift-left: w385 -> [w405]
                    shift-right: [w401] -> w382
                    shift-left: w389 -> [w402]
                    shift-right: [w399] -> w383
                    shift-left: w388 -> [w400]
                    n176 = Dequeue Element(queue=w405) -> (queue out=w404:refnum<queue>, element=w403:T8)  [unwired: 2 in, 2 out]
                    n177 = Enqueue Element(queue=w402, element=w403, error in (no error)=w400) -> (queue out=w401:refnum<queue>, error out=w399:errorcluster)  [unwired: 1 in, 1 out]
                  }
                  n178 = Close File(refnum=w374) -> ()  [unwired: 1 in, 2 out]
                  n179 = Close File(refnum=w373) -> ()  [unwired: 1 in, 2 out]
                }
                frame "Set_Ref" {
                  n180 = Unbundle By Name(w414) -> ("Data_Ref"=w408:T14)
                  n181 = Bundle By Name(cluster=w409, "Ref"=w408) -> (w407:T5)
                }
                frame "Set_Dark" {
                  n182 = Unbundle By Name(w423) -> ("Data_Dark"=w417:T14)
                  n183 = Bundle By Name(cluster=w418, "Dark"=w417) -> (w416:T5)
                }
                frame "Spectrometer_Measure" {
                  w429 = FALSE ("prepend array or string size? (T)")
                  w442 = enum16{"start", "end", "current"}."end" ("from (0:start)")
                  n184 = Unbundle By Name(w455) -> ("Data_Raw"=w451:T14, "Time"=w445:dbl[])
                  n185 = property on="LowerWLLimit" class="DigNum (strict)"() -> ("Value"=w426:i32)  [unwired: 2 in, 2 out]
                  n186 = To Unsigned Long Integer(number=w445) -> (unsigned 32bit integer=w431:u32[])
                  n187 = Index Array(array=w451, index=0) -> (element=w450:T15)
                  n188 = Unbundle By Name(w450) -> ("Image"=w428:dbl[][][])
                  n189 = property on="UpperWLLimit" class="DigNum (strict)"() -> ("Value"=w425:i32)  [unwired: 2 in, 2 out]
                  n190 = call "Trim_Spectra.vi"("WL_UpperIndex"=w425, "WL_LowerIndex"=w426, "Image"=w428) -> ("ImageCut"=w427:dbl[][][])
                  n191 = case shown="False" w439 {
                    tunnel: w456 -> [w488 _]
                    tunnel: w446 -> [w483 w494]
                    tunnel: [w470 w494] -> w433
                    tunnel: [w459 _] -> w434
                    tunnel: [w469 w493] -> w436
                    tunnel: [w458 w492] -> w435
                    tunnel: w427 -> [w467 _]
                    frame False {
                      w478 = T13."open or create" ("operation (0:open)")
                      w477 = "_" ("string")
                      n192 = property on="Measure_FileName" class="Str"() -> ("Value"=w486:string)  [unwired: 2 in, 2 out]
                      n193 = Concatenate Strings(w486, "_meas.spin" ("string")) -> (w489:string)
                      n194 = Concatenate Strings(w486, "_time.spin" ("string")) -> (w481:string)
                      n195 = Format Date/Time String(time format string (%c)="%Y%m%d_%H%M%S", seconds (now)=w488) -> (date/time string=w482:string)  [unwired: 1 in]
                      n196 = property on="Measure_SavePath" class="Path"() -> ("Value"=w461:path)  [unwired: 2 in, 2 out]
                      n197 = Concatenate Strings(w482, w477, w489) -> (w487:string)
                      n198 = Concatenate Strings(w482, w477, w481) -> (w480:string)
                      n199 = Build Path(base path=w461, name or relative path=w487) -> (appended path=w484:path)
                      n200 = Build Path(base path=w461, name or relative path=w480) -> (appended path=w479:path)
                      n201 = Array Size(array=w467) -> (size(s)=w466:i32[])
                      n202 = property on="Frames" class="DigNum (strict)"() -> ("Value"=w460:i32)  [unwired: 2 in, 2 out]
                      n203 = Open/Create/Replace File(file path (use dialog)=w484, error in=w483, operation (0:open)=w478) -> (refnum out=w457:refnum<file>, error out=w476:errorcluster)  [unwired: 3 in, 1 out]
                      n204 = Open/Create/Replace File(file path (use dialog)=w479, error in=w483, operation (0:open)=w478) -> (refnum out=w475:refnum<file>, error out=w474:errorcluster)  [unwired: 3 in, 1 out]
                      n205 = Write to Binary File(file (use dialog)=w457, data=w460, error in=w476) -> (refnum out=w473:refnum<file>, error out=w472:errorcluster)  [unwired: 3 in, 1 out]
                      n206 = Index Array(array=w466, index #1=2 ("index"), index #2=1 ("index")) -> (element #1=w462:i32, element #2=w463:i32)
                      n207 = Write to Binary File(file (use dialog)=w475, data=w460, error in=w474) -> (refnum out=w458:refnum<file>, error out=w459:errorcluster)  [unwired: 3 in, 1 out]
                      n208 = property on="Meas.spin" class="Ref (strict)"("Value"=w457) -> ()  [unwired: 2 in, 2 out]
                      n209 = Write to Binary File(file (use dialog)=w473, data=w463, error in=w472) -> (refnum out=w468:refnum<file>, error out=w471:errorcluster)  [unwired: 3 in, 1 out]
                      n210 = property on="Time.spin" class="Ref (strict)"("Value"=w458) -> ()  [unwired: 2 in, 2 out]
                      n211 = Write to Binary File(file (use dialog)=w468, data=w462, error in=w471) -> (refnum out=w469:refnum<file>, error out=w470:errorcluster)  [unwired: 3 in, 1 out]
                    }
                    frame True {
                      n212 = property on="Meas.spin" class="Ref (strict)"() -> ("Value"=w493:refnum<file>)  [unwired: 2 in, 2 out]
                      n213 = property on="Time.spin" class="Ref (strict)"() -> ("Value"=w492:refnum<file>)  [unwired: 2 in, 2 out]
                    }
                  }
                  n214 = To Unsigned Word Integer(number=w427) -> (unsigned 16bit integer=w430:u16[][][])
                  n215 = Merge Errors(w433, w434) -> (w432:errorcluster)
                  n216 = Set File Position(refnum=w436, from (0:start)=w442, error in=w432) -> (refnum out=w448:refnum<file>, error out=w447:errorcluster)  [unwired: 1 in]
                  n217 = Set File Position(refnum=w435, from (0:start)=w442, error in=w432) -> (refnum out=w453:refnum<file>, error out=w452:errorcluster)  [unwired: 1 in]
                  n218 = Write to Binary File(file (use dialog)=w453, data=w431, error in=w452, 5:w429) -> (error out=w437:errorcluster)  [unwired: 2 in, 2 out]
                  n219 = Write to Binary File(file (use dialog)=w448, data=w430, error in=w447, 5:w429) -> (error out=w438:errorcluster)  [unwired: 2 in, 2 out]
                  n220 = Merge Errors(w438, w437) -> (w444:errorcluster)
                }
                frame "Transfer_Settings" {
                  n221 = Unbundle By Name(w500) -> ("Device Information"=w499:string[])
                }
              }
              n222 = feedback-in #2(w313) -> ()
            }
            n223 = Release Queue(queue=w302) -> ()  [unwired: 2 in, 3 out]
          }
          frame "Measure_Spectrum" {
            w505 = T8 {"QueueAction"=enum."TimeOut", "Data"=[], "Data_Raw"=[], "Data_Dark"=[], "Data_Ref"=[], "Device Information"=[], "Numeric Control"=0.0, "Boolean"=FALSE, "Wavelength"=[], "Time"=[], "Time Stamp"=timestamp(0 s since 1904-01-01), "Numeric Control 2"=0.0, "TabControl"=enum."Measure", "Numeric Control 3"=0.0}  # DataQueue
            n224 = Obtain Queue(name (unnamed)="Temp", element data type=w505) -> (queue out=w504:refnum<queue>)  [unwired: 3 in, 2 out]
            n225 = while {
              shift-right: [w514] -> w508
              shift-left: w509 -> [w522]
              shift-right: [w515] -> w507
              shift-left: w510 -> [w523]
              shift-right: [w516] -> w503
              shift-left: w504 -> [w518]
              tunnel: w502 -> [w512]
              stop <- w513 stop-if-true
              n226 = Dequeue Element(queue=w522, error in (no error)=w523) -> (queue out=w520:refnum<queue>, element=w517:T8, error out=w519:errorcluster)  [unwired: 1 in, 1 out]
              n227 = Unbundle By Name(w517) -> ("QueueAction"=w521:T9, "TabControl"=w511:T10)
              n228 = case shown="\"Spectrometer_Measure\"" w521 {
                tunnel: w520 -> [w524 w552 w592]
                tunnel: w519 -> [w527 w562 w591]
                tunnel: w518 -> [w529 w568 w594]
                tunnel: w517 -> [w525 w541 _]
                tunnel: [w528 w568 w590] -> w516
                tunnel: [w526 w553 w588] -> w515
                tunnel: [w524 w552 w589] -> w514
                tunnel: [_ _ TRUE] -> w513
                tunnel: w512 -> [_ w545 _]
                tunnel: w511 -> [_ w539 w586]
                frame Default {
                  n229 = Enqueue Element(queue=w529, element=w525, error in (no error)=w527) -> (queue out=w528:refnum<queue>, error out=w526:errorcluster)  [unwired: 1 in, 1 out]
                }
                frame "Spectrometer_Measure" {
                  n230 = Unbundle By Name(w541) -> ("Data_Raw"=w559:T14)
                  n231 = case shown="\"Spectral Stability\"" w539 {
                    tunnel: [w581 "SpectralStability_SavePath"] -> w532
                    tunnel: [w580 "SpectralStability_FileName"] -> w530
                    tunnel: [w576 "SpectralStability_Comments"] -> w533
                    frame "Measure", Default {
                      n232 = property on="Spectra Count" class="DigNum (strict)"() -> ("Value"=w582:u16)  [unwired: 2 in, 2 out]
                      n233 = property on="Measure_SavePath" class="Path"() -> ("Value"=w581:path)  [unwired: 2 in, 2 out]
                      n234 = property on="Measure_Comments" class="Str"() -> ("Value"=w576:string)  [unwired: 2 in, 2 out]
                      n235 = property on="Measure_FileName" class="Str"() -> ("Value"=w577:string)  [unwired: 2 in, 2 out]
                      n236 = Number To Decimal String(number=w582) -> (decimal integer string=w578:string)  [unwired: 1 in]
                      n237 = Concatenate Strings(w577, "_", w578) -> (w580:string)
                    }
                    frame "Spectral Stability" {
                    }
                  }
                  n238 = Index Array(array=w559, index=0) -> (element=w557:T15)
                  n239 = Unbundle By Name(w541) -> ("Time Stamp"=w540:timestamp)
                  n240 = Unbundle By Name(w557) -> ("Image"=w535:dbl[][][])
                  n241 = Index Array(array=w535, index (dim 1)=0 ("disabled index (row)")) -> (element=w551:dbl[][])  [unwired: 2 in]
                  n242 = Transpose 2D Array(2D array=w551) -> (transposed array=w548:dbl[][])
                  n243 = Format Date/Time String(time format string (%c)="%Y%m%d_%H%M%S", seconds (now)=w540) -> (date/time string=w566:string)  [unwired: 1 in]
                  n244 = Matrix Size(0:w548) -> (2:w549:i32)  [unwired: 1 out]
                  n245 = Empty String/Path?(string/path=w533) -> (empty?=w534:bool)
                  n246 = Reciprocal(x=w549) -> (1/x=w550:dbl)
                  n247 = Concatenate Strings(w566, "_") -> (w531:string)
                  n248 = case shown="False" w534 {
                    tunnel: w533 -> [w575 _]
                    tunnel: w532 -> [w574 _]
                    tunnel: w531 -> [w573 _]
                    tunnel: w530 -> [w572 _]
                    frame False {
                      n249 = Concatenate Strings(w573, w572, "_comments.txt" ("string")) -> (w569:string)
                      n250 = Build Path(base path=w574, name or relative path=w569) -> (appended path=w570:path)
                      n251 = Write to Text File(file (use dialog)=w570, text=w575) -> ()  [unwired: 2 in, 3 out]
                    }
                    frame True {
                    }
                  }
                  n252 = Initialize Array(w550, w549) -> (w547:dbl[])
                  n253 = Concatenate Strings(w531, w530, ".spectra" ("string")) -> (w537:string)
                  n254 = Unbundle By Name(w545) -> ("Wavlength"=w542:dbl[unit][])
                  n255 = call-poly <vilib>:"A x B.vi"("Vector"=w547, "A"=w548) -> ("A x Vector"=w536:dbl[])  [unwired: 1 out]
                  n256 = Build Path(base path=w532, name or relative path=w537) -> (appended path=w564:path)
                  n257 = Bundle("Wavlength"=w542, "A x Vector"=w536) -> (w544:T16)  [unwired: 1 in]
                  n258 = Open/Create/Replace File(file path (use dialog)=w564, error in=w562, operation (0:open)=T13."open or create") -> (refnum out=w561:refnum<file>, error out=w560:errorcluster)  [unwired: 3 in, 1 out]
                  n259 = Build Array(w544) -> (w543:T17)
                  n260 = To Unsigned Word Integer(number=w535) -> (unsigned 16bit integer=w556:u16[][][])
                  n261 = property on="Measure_Graph" class="XYGraph (strict)"("Value"=w543) -> ()  [unwired: 2 in, 2 out]
                  n262 = Write to Binary File(file (use dialog)=w561, data=w556, error in=w560) -> (refnum out=w554:refnum<file>, error out=w555:errorcluster)  [unwired: 3 in, 1 out]
                  n263 = Close File(refnum=w554, error in=w555) -> (error out=w553:errorcluster)  [unwired: 1 out]
                }
                frame "Stop_Measurement" {
                  w587 = FALSE ("Measure Spectrum")
                  n264 = case shown="Default" w586 {
                    frame Default {
                    }
                    frame "Measure" {
                      n265 = property on="Automatically \nadjust count" class="Bool (strict)"() -> ("Value"=w597:bool)  [unwired: 2 in, 2 out]
                      n266 = case shown="True" w597 {
                        frame False {
                        }
                        frame True {
                          n267 = Increment(x="Spectra Count") -> (x+1=w598:u16)
                          n268 = property on="Spectra Count" class="DigNum (strict)"("Value"=w598) -> ()  [unwired: 2 in, 2 out]
                        }
                      }
                    }
                  }
                  n269 = Get Queue Status(queue=w594) -> (queue out=w595:refnum<queue>, # elements in queue=w593:i32)  [unwired: 2 in, 6 out]
                  n270 = property on="SpectralStability_MeasureSpectrum" class="Bool (strict)"("Value"=w587) -> ()  [unwired: 2 in, 2 out]
                  n271 = property on="Measure_MeasureSpectrum" class="Bool (strict)"("Value"=w587) -> ()  [unwired: 2 in, 2 out]
                  n272 = for {
                    N: w593 -> [_]
                    shift-right: [w605] -> w590
                    shift-left: w595 -> [w606]
                    shift-right: [w602] -> w589
                    shift-left: w592 -> [w603]
                    shift-right: [w600] -> w588
                    shift-left: w591 -> [w601]
                    n273 = Dequeue Element(queue=w606) -> (queue out=w605:refnum<queue>, element=w604:T8)  [unwired: 2 in, 2 out]
                    n274 = Enqueue Element(queue=w603, element=w604, error in (no error)=w601) -> (queue out=w602:refnum<queue>, error out=w600:errorcluster)  [unwired: 1 in, 1 out]
                  }
                }
              }
            }
            n275 = Release Queue(queue=w503) -> ()  [unwired: 2 in, 3 out]
          }
          frame "Measure_SpectrumAdvanced" {
            w610 = T8 {"QueueAction"=enum."TimeOut", "Data"=[], "Data_Raw"=[], "Data_Dark"=[], "Data_Ref"=[], "Device Information"=[], "Numeric Control"=0.0, "Boolean"=FALSE, "Wavelength"=[], "Time"=[], "Time Stamp"=timestamp(0 s since 1904-01-01), "Numeric Control 2"=0.0, "TabControl"=enum."Measure", "Numeric Control 3"=0.0}  # DataQueue
            n276 = Obtain Queue(name (unnamed)="Temp", element data type=w610) -> (queue out=w609:refnum<queue>)  [unwired: 3 in, 2 out]
            n277 = while {
              shift-right: [w618] -> w613
              shift-left: w614 -> [w626]
              shift-right: [w619] -> w612
              shift-left: w615 -> [w627]
              shift-right: [w620] -> w608
              shift-left: w609 -> [w622]
              tunnel: w607 -> [w616]
              stop <- w617 stop-if-true
              n278 = Dequeue Element(queue=w626, error in (no error)=w627) -> (queue out=w624:refnum<queue>, element=w621:T8, error out=w623:errorcluster)  [unwired: 1 in, 1 out]
              n279 = Unbundle By Name(w621) -> ("QueueAction"=w625:T9)
              n280 = case shown="\"Stop_Measurement\"" w625 {
                tunnel: w624 -> [w628 w652 w678]
                tunnel: w623 -> [w631 w662 w677]
                tunnel: w622 -> [w633 w671 w680]
                tunnel: w621 -> [w629 w639 _]
                tunnel: [w632 w671 w676] -> w620
                tunnel: [w630 w653 w674] -> w619
                tunnel: [w628 w652 w675] -> w618
                tunnel: [_ _ TRUE] -> w617
                tunnel: w616 -> [_ w644 _]
                frame Default {
                  n281 = Enqueue Element(queue=w633, element=w629, error in (no error)=w631) -> (queue out=w632:refnum<queue>, error out=w630:errorcluster)  [unwired: 1 in, 1 out]
                }
                frame "Spectrometer_Measure" {
                  w668 = "_"
                  n282 = Unbundle By Name(w639) -> ("Time Stamp"=w638:timestamp)
                  n283 = property on="Nr After Spin" class="DigNum (strict)"() -> ("Value"=w637:u16)  [unwired: 2 in, 2 out]
                  n284 = Unbundle By Name(w644) -> ("Wavlength"=w641:dbl[unit][])
                  n285 = property on="Measure_FileName" class="Str"() -> ("Value"=w667:string)  [unwired: 2 in, 2 out]
                  n286 = Number To Decimal String(number=w637) -> (decimal integer string=w635:string)  [unwired: 1 in]
                  n287 = Format Date/Time String(time format string (%c)="%Y%m%d_%H%M%S", seconds (now)=w638) -> (date/time string=w669:string)  [unwired: 1 in]
                  n288 = Concatenate Strings(w669, w668, w667, w668, "a" ("string"), w635, ".spectra" ("string")) -> (w666:string)
                  n289 = property on="Measure_SavePath" class="Path"() -> ("Value"=w665:path)  [unwired: 2 in, 2 out]
                  n290 = Build Path(base path=w665, name or relative path=w666) -> (appended path=w664:path)
                  n291 = Unbundle By Name(w639) -> ("Data_Raw"=w659:T14)
                  n292 = Open/Create/Replace File(file path (use dialog)=w664, error in=w662, operation (0:open)=T13."open or create") -> (refnum out=w661:refnum<file>, error out=w660:errorcluster)  [unwired: 3 in, 1 out]
                  n293 = Index Array(array=w659, index=0) -> (element=w657:T15)
                  n294 = Unbundle By Name(w657) -> ("Image"=w645:dbl[][][])
                  n295 = Index Array(array=w645, index (dim 1)=0 ("disabled index (row)")) -> (element=w651:dbl[][])  [unwired: 2 in]
                  n296 = Transpose 2D Array(2D array=w651) -> (transposed array=w648:dbl[][])
                  n297 = To Unsigned Word Integer(number=w645) -> (unsigned 16bit integer=w656:u16[][][])
                  n298 = Matrix Size(0:w648) -> (2:w649:i32)  [unwired: 1 out]
                  n299 = Write to Binary File(file (use dialog)=w661, data=w656, error in=w660) -> (refnum out=w654:refnum<file>, error out=w655:errorcluster)  [unwired: 3 in, 1 out]
                  n300 = Reciprocal(x=w649) -> (1/x=w650:dbl)
                  n301 = Close File(refnum=w654, error in=w655) -> (error out=w653:errorcluster)  [unwired: 1 out]
                  n302 = Initialize Array(w650, w649) -> (w647:dbl[])
                  n303 = call-poly <vilib>:"A x B.vi"("Vector"=w647, "A"=w648) -> ("A x Vector"=w640:dbl[])  [unwired: 1 out]
                  n304 = Bundle("Wavlength"=w641, "A x Vector"=w640) -> (w643:T16)  [unwired: 1 in]
                  n305 = Build Array(w643) -> (w642:T17)
                  n306 = property on="Measure_Graph" class="XYGraph (strict)"("Value"=w642) -> ()  [unwired: 2 in, 2 out]
                }
                frame "Stop_Measurement" {
                  n307 = property on="Automatically \nadjust count" class="Bool (strict)"() -> ("Value"=w672:bool)  [unwired: 2 in, 2 out]
                  n308 = case shown="True" w672 {
                    frame False {
                    }
                    frame True {
                      n309 = property on="Nr After Spin" class="DigNum (strict)"() -> ("Value"=w684:u16)  [unwired: 2 in, 2 out]
                      n310 = Increment(x=w684) -> (x+1=w683:u16)
                      n311 = property on="Nr After Spin" class="DigNum (strict)"("Value"=w683) -> ()  [unwired: 2 in, 2 out]
                    }
                  }
                  n312 = Get Queue Status(queue=w680) -> (queue out=w681:refnum<queue>, # elements in queue=w679:i32)  [unwired: 2 in, 6 out]
                  n313 = property on="Measure_MeasureSpectrum" class="Bool (strict)"("Value"=FALSE ("Measure Spectrum")) -> ()  [unwired: 2 in, 2 out]
                  n314 = for {
                    N: w679 -> [_]
                    shift-right: [w690] -> w676
                    shift-left: w681 -> [w691]
                    shift-right: [w687] -> w675
                    shift-left: w678 -> [w688]
                    shift-right: [w685] -> w674
                    shift-left: w677 -> [w686]
                    n315 = Dequeue Element(queue=w691) -> (queue out=w690:refnum<queue>, element=w689:T8)  [unwired: 2 in, 2 out]
                    n316 = Enqueue Element(queue=w688, element=w689, error in (no error)=w686) -> (queue out=w687:refnum<queue>, error out=w685:errorcluster)  [unwired: 1 in, 1 out]
                  }
                }
              }
            }
            n317 = Release Queue(queue=w608) -> ()  [unwired: 2 in, 3 out]
          }
          frame "Measure_SpectralStability" {
            w707 = T8 {"QueueAction"=enum."TimeOut", "Data"=[], "Data_Raw"=[], "Data_Dark"=[], "Data_Ref"=[], "Device Information"=[], "Numeric Control"=0.0, "Boolean"=FALSE, "Wavelength"=[], "Time"=[], "Time Stamp"=timestamp(0 s since 1904-01-01), "Numeric Control 2"=0.0, "TabControl"=enum."Measure", "Numeric Control 3"=0.0}  # DataQueue
            n318 = Unbundle By Name(w696) -> ("Time Stamp"=w702:timestamp)
            n319 = Unbundle By Name(w696) -> ("Numeric Control"=w692:dbl)
            n320 = property on="SpectralStability\n_SavePath" class="Path"() -> ("Value"=w698:path)  [unwired: 2 in, 2 out]
            n321 = property on="SpectralStability\n_FileName" class="Str"() -> ("Value"=w697:string)  [unwired: 2 in, 2 out]
            n322 = Obtain Queue(name (unnamed)="Temp", element data type=w707) -> (queue out=w706:refnum<queue>)  [unwired: 3 in, 2 out]
            n323 = call "Num2Str_TrailingZero.vi"("Numeric Control"=w692) -> ("format string"=w695:string)  [unwired: 10 in]
            n324 = Format Date/Time String(time format string (%c)="%Y%m%d_%H%M%S", seconds (now)=w702) -> (date/time string=w699:string)  [unwired: 1 in]
            n325 = while {
              shift-right: [w712] -> w700
              shift-left: w709 -> [w712]
              shift-right: [w718] -> _
              shift-left: w706 -> [w720]
              border: 0 -> [_]
              shift-right: [w719] -> w693
              shift-left: w704 -> [w728]
              shift-right: [w717] -> w694
              shift-left: w703 -> [w727]
              tunnel: w699 -> [w715]
              tunnel: w698 -> [w714]
              tunnel: w697 -> [w713]
              tunnel: w695 -> [w711]
              tunnel: w692 -> [w710]
              stop <- w716 stop-if-true
              n326 = Dequeue Element(queue=w728, error in (no error)=w727) -> (queue out=w726:refnum<queue>, element=w724:T8, error out=w725:errorcluster)  [unwired: 1 in, 1 out]
              n327 = Unbundle By Name(w724) -> ("QueueAction"=w723:T9)
              n328 = feedback #3() -> (w721:i32)
              n329 = case shown="\"Spectrometer_Measure\"" w723 {
                tunnel: w726 -> [w732 w741 w747 w765 w848 w855]
                tunnel: w725 -> [w731 w738 w748 w766 _ w856]
                tunnel: w724 -> [w733 w737 _ _ w802 w887]
                tunnel: [w735 w743 w754 w772 w786 w888] -> w722
                tunnel: w721 -> [w735 w743 w754 w772 w846 w888]
                tunnel: w720 -> [w734 w742 w750 w768 w847 w865]
                tunnel: [w732 w740 w745 w763 w848 w855] -> w719
                tunnel: [w730 w742 w749 w767 w847 w865] -> w718
                tunnel: [w729 w739 w746 w764 w791 w856] -> w717
                tunnel: [_ TRUE TRUE TRUE _ _] -> w716
                tunnel: w715 -> [_ _ _ _ w844 w885]
                tunnel: w714 -> [_ _ _ _ w811 w853]
                tunnel: w713 -> [_ _ _ _ w843 w883]
                tunnel: w712 -> [_ _ _ _ w818 w882]
                tunnel: w711 -> [_ _ _ _ w845 _]
                tunnel: w710 -> [_ _ _ _ w787 _]
                frame Default {
                  n330 = Enqueue Element(queue=w734, element=w733, error in (no error)=w731) -> (queue out=w730:refnum<queue>, error out=w729:errorcluster)  [unwired: 1 in, 1 out]
                }
                frame "Close_Program" {
                  n331 = Enqueue Element At Opposite End(queue=w741, element=w737, error in (no error)=w738) -> (queue out=w740:refnum<queue>, error out=w739:errorcluster)  [unwired: 1 in, 1 out]
                }
                frame "Abort" {
                  n332 = Get Queue Status(queue=w750) -> (queue out=w752:refnum<queue>, # elements in queue=w753:i32)  [unwired: 2 in, 6 out]
                  n333 = for {
                    N: w753 -> [_]
                    shift-right: [w760] -> w749
                    shift-left: w752 -> [w761]
                    shift-right: [w757] -> w745
                    shift-left: w747 -> [w758]
                    shift-right: [w755] -> w746
                    shift-left: w748 -> [w756]
                    n334 = Dequeue Element(queue=w761) -> (queue out=w760:refnum<queue>, element=w759:T8)  [unwired: 2 in, 2 out]
                    n335 = Enqueue Element(queue=w758, element=w759, error in (no error)=w756) -> (queue out=w757:refnum<queue>, error out=w755:errorcluster)  [unwired: 1 in, 1 out]
                  }
                  n336 = property on="SpectralStability_Record" class="Bool (strict)"("Value"=FALSE ("SpectralStability_Record")) -> ()  [unwired: 2 in, 2 out]
                }
                frame "Stop_Measurement" {
                  n337 = Get Queue Status(queue=w768) -> (queue out=w770:refnum<queue>, # elements in queue=w771:i32)  [unwired: 2 in, 6 out]
                  n338 = for {
                    N: w771 -> [_]
                    shift-right: [w778] -> w767
                    shift-left: w770 -> [w779]
                    shift-right: [w775] -> w763
                    shift-left: w765 -> [w776]
                    shift-right: [w773] -> w764
                    shift-left: w766 -> [w774]
                    n339 = Dequeue Element(queue=w779) -> (queue out=w778:refnum<queue>, element=w777:T8)  [unwired: 2 in, 2 out]
                    n340 = Enqueue Element(queue=w776, element=w777, error in (no error)=w774) -> (queue out=w775:refnum<queue>, error out=w773:errorcluster)  [unwired: 1 in, 1 out]
                  }
                  n341 = property on="SpectralStability_Record" class="Bool (strict)"("Value"=FALSE ("SpectralStability_Record")) -> ()  [unwired: 2 in, 2 out]
                }
                frame "Spectrometer_Measure" {
                  w842 = "_"
                  n342 = Increment(x=w846) -> (x+1=w786:i32)
                  n343 = Unbundle By Name(w802) -> ("Numeric Control 2"=w801:dbl)
                  n344 = Unbundle By Name(w802) -> ("Data_Raw"=w840:T14)
                  n345 = Format Into String(format string=w845, w846) -> (resulting string=w800:string)  [unwired: 2 in, 1 out]
                  n346 = Concatenate Strings(w844, w842, w843, w842) -> (w813:string)
                  n347 = Unbundle By Name(w818) -> ("Wavlength"=w816:dbl[unit][])
                  n348 = Index Array(array=w840, index=0) -> (element=w838:T15)
                  n349 = Divide(x=w786, y=w787) -> (x/y=w790:dbl)
                  n350 = Concatenate Strings(w813, "s" ("string"), w800, ".smean" ("string")) -> (w822:string)
                  n351 = Concatenate Strings(w813, "raw" ("string"), w800, ".spectra" ("string")) -> (w830:string)
                  n352 = Unbundle By Name(w838) -> ("Image"=w826:dbl[][][])
                  n353 = Concatenate Strings(w813, "timing.txt" ("string")) -> (w810:string)
                  n354 = Subtract(x=w787, y=w786) -> (x-y=w782:dbl)
                  "SS_StepsLeft" <- w782
                  n355 = Number To Exponential String(number=w801, 1:FALSE ("use system decimal point (T)")) -> (E-format string=w798:string)  [unwired: 2 in]
                  n356 = Build Path(base path=w811, name or relative path=w822) -> (appended path=w819:path)
                  n357 = Build Path(base path=w811, name or relative path=w810) -> (appended path=w809:path)
                  n358 = Multiply(x=w790, y=100.0) -> (x*y=w789:dbl)
                  n359 = property on="SS:PeriodicTime" class="DigNum (strict)"() -> ("Value"=w784:dbl[unit])  [unwired: 2 in, 2 out]
                  n360 = Build Path(base path=w811, name or relative path=w830) -> (appended path=w827:path)
                  n361 = Index Array(array=w826, index (dim 1)=0 ("disabled index (row)")) -> (element=w837:dbl[][])  [unwired: 2 in]
                  n362 = To Unsigned Byte Integer(number=w789) -> (unsigned 8bit integer=→"Horizontal Progress Bar":u8)
                  n363 = To Unsigned Word Integer(number=w826) -> (unsigned 16bit integer=w825:u16[][][])
                  n364 = Open/Create/Replace File(file path (use dialog)=w809, operation (0:open)=T13."open or create") -> (refnum out=w807:refnum<file>, error out=w804:errorcluster)  [unwired: 4 in, 1 out]
                  n365 = Concatenate Strings(w800, "\t", w798, "\r\n") -> (w797:string)
                  n366 = Transpose 2D Array(2D array=w837) -> (transposed array=w834:dbl[][])
                  n367 = Write to Binary File(file (use dialog)=w827, data=w825) -> (refnum out=w823:refnum<file>, error out=w824:errorcluster)  [unwired: 4 in, 1 out]
                  n368 = Multiply(x=w784, y=w782) -> (x*y=→"SS_TimePrediction":dbl[unit])
                  n369 = Set File Position(refnum=w807, from (0:start)=enum16{"start", "end", "current"}."end", error in=w804) -> (refnum out=w805:refnum<file>, error out=w803:errorcluster)  [unwired: 1 in]
                  n370 = Matrix Size(0:w834) -> (2:w835:i32)  [unwired: 1 out]
                  n371 = Close File(refnum=w823, error in=w824) -> (error out=w794:errorcluster)  [unwired: 1 out]
                  n372 = Reciprocal(x=w835) -> (1/x=w836:dbl)
                  n373 = Write to Text File(file (use dialog)=w805, text=w797, error in=w803) -> (refnum out=w796:refnum<file>, error out=w795:errorcluster)  [unwired: 1 in, 1 out]
                  n374 = Initialize Array(w836, w835) -> (w833:dbl[])
                  n375 = call-poly <vilib>:"A x B.vi"("Vector"=w833, "A"=w834) -> ("A x Vector"=w815:dbl[])  [unwired: 1 out]
                  n376 = Bundle("Wavlength"=w816, "A x Vector"=w815) -> (w817:T16)  [unwired: 1 in]
                  n377 = Close File(refnum=w796, error in=w795) -> (error out=w792:errorcluster)  [unwired: 1 out]
                  n378 = Write to Binary File(file (use dialog)=w819, data=w815) -> (refnum out=w821:refnum<file>, error out=w820:errorcluster)  [unwired: 4 in, 1 out]
                  n379 = Build Array(w817) -> (w814:T17)
                  n380 = Close File(refnum=w821, error in=w820) -> (error out=w793:errorcluster)  [unwired: 1 out]
                  n381 = property on="SpectralStability:\nGraph" class="XYGraph (strict)"("Value"=w814) -> ()  [unwired: 2 in, 2 out]
                  n382 = Merge Errors(w794, w793, w792) -> (w791:errorcluster)
                }
                frame "Transfer_Settings" {
                  w858 = "\r\n"
                  w872 = 0.0
                  w878 = 0 ("index")
                  n383 = Unbundle By Name(w882) -> ("Dark"=w879:T14, "Ref"=w880:T14, "Wavlength"=w881:dbl[unit][])
                  n384 = Concatenate Strings(w885, "_", w883) -> (w871:string)
                  n385 = property on="SpectralStability_\nPeriodicTime" class="DigNum (strict)"() -> ("Value"=w864:dbl[unit])  [unwired: 2 in, 2 out]
                  n386 = Unbundle By Name(w887) -> ("Device Information"=w886:string[])
                  n387 = property on="SpectralStability_Duration" class="DigNum (strict)"() -> ("Value"=w863:dbl[unit])  [unwired: 2 in, 2 out]
                  n388 = Index Array(array=w879, index=w878) -> (element=w876:T15)
                  n389 = Index Array(array=w880, index=w878) -> (element=w877:T15)
                  n390 = Concatenate Strings(w871, "_add.spin" ("string")) -> (w868:string)
                  n391 = Concatenate Strings(w871, "_comments.txt" ("string")) -> (w854:string)
                  n392 = Unbundle By Name(w876) -> ("Image"=w850:dbl[][][])
                  n393 = Unbundle By Name(w877) -> ("Image"=w849:dbl[][][])
                  n394 = property on="SpectralStability_\nMeasurementNumber" class="DigNum (strict)"() -> ("Value"=w862:u32)  [unwired: 2 in, 2 out]
                  n395 = Build Path(base path=w853, name or relative path=w868) -> (appended path=w867:path)
                  n396 = Build Path(base path=w853, name or relative path=w854) -> (appended path=w852:path)
                  n397 = node(w881) -> (w873:dbl[])
                  n398 = property on="Duration/Times" class="Bool (strict)"() -> ("Value"=w861:bool)  [unwired: 2 in, 2 out]
                  n399 = To Unsigned Word Integer(number=w850) -> (unsigned 16bit integer=w875:u16[][][])
                  n400 = To Unsigned Word Integer(number=w849) -> (unsigned 16bit integer=w874:u16[][][])
                  n401 = call "DeviceInfo2Str.vi"("Device Information"=w886) -> ("String"=w860:string)  [unwired: 10 in]
                  n402 = property on="SpectralStability:\nComments" class="Str"() -> ("Value"=w857:string)  [unwired: 2 in, 2 out]
                  n403 = Bundle(w875, w874, w873, w872, w872) -> (w866:cluster{u16[][][], u16[][][], dbl[], dbl, dbl})  [unwired: 1 in]
                  n404 = call "String_SpectralStabilitySettings.vi"("Duration/Times"=w861, "Measurement Number"=w862, "Duration"=w863, "Periodic Time"=w864) -> ("String"=w859:string)  [unwired: 7 in]
                  n405 = Concatenate Strings(w860, w858, w859, w858, w857) -> (w851:string)
                  n406 = Write to Binary File(file (use dialog)=w867, data=w866) -> ()  [unwired: 4 in, 3 out]
                  n407 = Write to Text File(file (use dialog)=w852, text=w851) -> ()  [unwired: 2 in, 3 out]
                }
              }
              n408 = feedback-in #3(w722) -> ()
            }
          }
          frame "Save_InSitu" {
            w906 = "\r\n"
            n409 = Unbundle By Name(w940) -> ("Time Stamp"=w938:timestamp, "Device Information"=w930:string[], "Numeric Control"=w927:dbl, "Numeric Control 2"=w926:dbl, "Numeric Control 3"=w890:dbl)
            n410 = case shown="0, Default" w890 {
              tunnel: ["In-Situ Normal:\n" ("string") "In-Situ Short\n" ("string")] -> w889
              frame 0, Default {
              }
              frame 1 {
              }
            }
            n411 = Unbundle By Name(w928) -> ("Dark"=w946:T14, "Ref"=w944:T14, "Wavlength Trim"=w948:dbl[unit][])
            n412 = property on="Threshold" class="DigNum (strict)"() -> ("Value"=w891:dbl)  [unwired: 2 in, 2 out]
            n413 = node(w948) -> (w941:dbl[])
            n414 = property on="Frames" class="DigNum (strict)"() -> ("Value"=w914:i32)  [unwired: 2 in, 2 out]
            n415 = property on="Wavelenght Detect" class="DigNum (strict)"() -> ("Value"=w892:dbl[unit])  [unwired: 2 in, 2 out]
            n416 = call "DeviceInfo2Str.vi"("Device Information"=w930) -> ("String"=w929:string)  [unwired: 10 in]
            n417 = Number To Decimal String(number=w914) -> (decimal integer string=w913:string)  [unwired: 1 in]
            n418 = Index Array(array=w944, index=0) -> (element=w942:T15)
            n419 = property on="Time Detect" class="DigNum (strict)"() -> ("Value"=w893:dbl[unit])  [unwired: 2 in, 2 out]
            n420 = property on="LowerWLLimit" class="DigNum (strict)"() -> ("Value"=w902:i32)  [unwired: 2 in, 2 out]
            n421 = Index Array(array=w946, index=0) -> (element=w943:T15)
            n422 = property on="Measure_FileName" class="Str"() -> ("Value"=w923:string)  [unwired: 2 in, 2 out]
            n423 = property on="Spin Time" class="DigNum (strict)"() -> ("Value"=w894:dbl[unit])  [unwired: 2 in, 2 out]
            n424 = property on="Seconds to Spin_Normal" class="DigNum (strict)"() -> ("Value"=w896:dbl[unit])  [unwired: 2 in, 2 out]
            n425 = Unbundle By Name(w943) -> ("Image"=w903:dbl[][][])
            n426 = Unbundle By Name(w942) -> ("Image"=w904:dbl[][][])
            n427 = property on="UpperWLLimit" class="DigNum (strict)"() -> ("Value"=w901:i32)  [unwired: 2 in, 2 out]
            n428 = Format Date/Time String(time format string (%c)="%Y%m%d_%H%M%S", seconds (now)=w938) -> (date/time string=w937:string)  [unwired: 1 in]
            n429 = property on="Seconds after Spin" class="DigNum (strict)"() -> ("Value"=w895:dbl[unit])  [unwired: 2 in, 2 out]
            n430 = Concatenate Strings(w937, "_" ("string"), w923) -> (w935:string)
            n431 = property on="Program Spin Coater" class="Arr (strict)"() -> ("Value"=w912:T2)  [unwired: 2 in, 2 out]
            n432 = call "Trim_Spectra.vi"("WL_UpperIndex"=w901, "WL_LowerIndex"=w902, "Image"=w904) -> ("ImageCut"=w899:dbl[][][])
            n433 = call "Trim_Spectra.vi"("WL_UpperIndex"=w901, "WL_LowerIndex"=w902, "Image"=w903) -> ("ImageCut"=w900:dbl[][][])
            n434 = call "MeasurementSpin2String_v02.vi"("Program Spin Coater"=w912, "Seconds to Spin Start"=w896, "Seconds after Spin Stop"=w895, "Spin Time"=w894, "Time Detect"=w893, "Wavelength Detect"=w892, "Threshold"=w891) -> ("concatenated string"=w911:string)  [unwired: 8 in]
            n435 = To Unsigned Word Integer(number=w899) -> (unsigned 16bit integer=w916:u16[][][])
            n436 = To Unsigned Word Integer(number=w900) -> (unsigned 16bit integer=w917:u16[][][])
            n437 = property on="Duration after" class="DigNum (strict)"() -> ("Value"=w908:dbl[unit])  [unwired: 2 in, 2 out]
            n438 = property on="periodic time" class="DigNum (strict)"() -> ("Value"=w909:dbl[unit])  [unwired: 2 in, 2 out]
            n439 = property on="Spin at end" class="Bool (strict)"() -> ("Value"=w907:bool)  [unwired: 2 in, 2 out]
            n440 = call "AfterSpinOptions.vi"("Spin at end"=w907, "Duration after"=w908, "periodic time"=w909) -> ("concatenated string"=w910:string)  [unwired: 8 in]
            n441 = Concatenate Strings(w889, w929, w906, "Frames:\t" ("string"), w913, w906, w911, w906, w910, w906, "Comments:" ("string"), w906, "Measure_Comments") -> (w925:string)
            n442 = Bundle(w917, w916, w941, "Numeric Control"=w927, "Numeric Control 2"=w926) -> (w920:T18)  [unwired: 1 in]
            n443 = property on="Measure_SavePath" class="Path"() -> ("Value"=w922:path)  [unwired: 2 in, 2 out]
            n444 = Concatenate Strings(w935, "_add.spin" ("string")) -> (w934:string)
            n445 = Concatenate Strings(w935, "_comments.txt" ("string")) -> (w933:string)
            n446 = Build Path(base path=w922, name or relative path=w934) -> (appended path=w921:path)
            n447 = Build Path(base path=w922, name or relative path=w933) -> (appended path=w932:path)
            n448 = Write to Text File(file (use dialog)=w932, text=w925) -> (error out=w919:errorcluster)  [unwired: 2 in, 2 out]
            n449 = Write to Binary File(file (use dialog)=w921, data=w920) -> (error out=w918:errorcluster)  [unwired: 4 in, 2 out]
            n450 = flat-sequence {
              tunnel: w919 -> [_]
              tunnel: w918 -> [_]
              frame #0 {
                n451 = property on="Action" class="Str"("Value"="" ("Action")) -> ()  [unwired: 2 in, 2 out]
              }
            }
            n452 = property on="Action" class="Str"("Value"="Saving" ("Action")) -> ()  [unwired: 2 in, 2 out]
          }
          frame "Set_Dark" {
            # "Averaging"
            n453 = Unbundle By Name(w965) -> ("Wavlength"=w964:dbl[unit][])
            n454 = Unbundle By Name(w972) -> ("Data_Dark"=w962:T14)
            n455 = Index Array(array=w962, index=0) -> (element=w967:T15)
            n456 = Unbundle By Name(w967) -> ("Image"=w961:dbl[][][])
            n457 = Index Array(array=w961, index (dim 1)=0 ("disabled index (row)")) -> (element=w959:dbl[][])  [unwired: 2 in]
            n458 = Transpose 2D Array(2D array=w959) -> (transposed array=w956:dbl[][])
            n459 = Matrix Size(0:w956) -> (2:w957:i32)  [unwired: 1 out]
            n460 = Reciprocal(x=w957) -> (1/x=w958:dbl)
            n461 = Initialize Array(w958, w957) -> (w955:dbl[])
            n462 = call-poly <vilib>:"A x B.vi"("Vector"=w955, "A"=w956) -> ("A x Vector"=w954:dbl[])  [unwired: 1 out]
            n463 = Bundle("Wavlength"=w964, "A x Vector"=w954) -> (w966:T16)  [unwired: 1 in]
            n464 = Build Array(w966) -> (w963:T17)
            n465 = property on="Measure_Graph" class="XYGraph (strict)"("Value"=w963) -> ()  [unwired: 2 in, 2 out]
            n466 = Bundle By Name(cluster=w965, "Dark"=w962) -> (w969:T5)
          }
          frame "Set_Ref" {
            # "Averaging"
            n467 = Unbundle By Name(w974) -> ("Wavlength"=w973:dbl[unit][])
            n468 = Unbundle By Name(w991) -> ("Data_Ref"=w978:T14)
            n469 = Index Array(array=w978, index=0) -> (element=w986:T15)
            n470 = Unbundle By Name(w986) -> ("Image"=w985:dbl[][][])
            n471 = Index Array(array=w985, index (dim 1)=0 ("disabled index (row)")) -> (element=w983:dbl[][])  [unwired: 2 in]
            n472 = Transpose 2D Array(2D array=w983) -> (transposed array=w980:dbl[][])
            n473 = Matrix Size(0:w980) -> (2:w981:i32)  [unwired: 1 out]
            n474 = Reciprocal(x=w981) -> (1/x=w982:dbl)
            n475 = Initialize Array(w982, w981) -> (w979:dbl[])
            n476 = call-poly <vilib>:"A x B.vi"("Vector"=w979, "A"=w980) -> ("A x Vector"=w975:dbl[])  [unwired: 1 out]
            n477 = Bundle("Wavlength"=w973, "A x Vector"=w975) -> (w977:T16)  [unwired: 1 in]
            n478 = Build Array(w977) -> (w976:T17)
            n479 = Bundle By Name(cluster=w974, "Ref"=w978) -> (w988:T5)
            n480 = property on="Measure_Graph" class="XYGraph (strict)"("Value"=w976) -> ()  [unwired: 2 in, 2 out]
          }
          frame "Set_Wavelength" {
            n481 = Unbundle By Name(w995) -> ("Wavelength"=w998:dbl[unit][])
            n482 = Bundle By Name(cluster=w997, "Wavlength"=w998) -> (w996:T5)
            n483 = property on="Trim\nSpec" class="Bool (strict)"() -> ("Value"=w992:bool)  [unwired: 2 in, 2 out]
            n484 = property on="Trim\nSpec" class="Bool (strict)"("Val(Sgnl)"=w992) -> ()  [unwired: 2 in, 2 out]
          }
          frame "Spectrometer_Preview" {
            w1005 = 0 ("index (page)")
            n485 = Unbundle By Name(w1001) -> ("Data_Raw"=w1009:T14)
            n486 = Unbundle By Name(w1010) -> ("Wavlength"=w1004:dbl[unit][])
            n487 = Unbundle By Name(w1001) -> ("TabControl"=w1000:T10)
            n488 = Index Array(array=w1009, index=0) -> (element=w1007:T15)
            n489 = Unbundle By Name(w1007) -> ("Image"=w1006:dbl[][][])
            n490 = Index Array(array=w1006, index (dim 0)=w1005, index (dim 1)=w1005) -> (element=w1003:dbl[])  [unwired: 1 in]
            n491 = Bundle("Wavlength"=w1004, "Image"=w1003) -> (w1002:cluster{"Wavlength":dbl[unit][], "Image":dbl[]})  [unwired: 1 in]
            n492 = Build Array(w1002) -> (w999:T3)
            n493 = case shown="Default" w1000 {
              tunnel: w999 -> [w1013 w1014 _]
              frame "Measure" {
                "Measure_Graph" <- w1013
              }
              frame "Spectral Stability" {
                "SpectralStability_Graph" <- w1014
              }
              frame Default {
              }
            }
          }
          frame "Change_TrimSettings" {
            n494 = Unbundle By Name(w1022) -> ("Boolean"=w1021:bool)
            n495 = case shown="True" w1021 {
              tunnel: w1017 -> [w1028 w1046]
              tunnel: w1022 -> [_ w1041]
              tunnel: [0 w1032] -> w1019
              tunnel: [w1026 w1033] -> w1018
              tunnel: [w1024 w1029] -> w1015
              frame False {
                n496 = Unbundle By Name(w1028) -> ("Wavlength"=w1024:dbl[unit][])
                n497 = Array Size(array=w1024) -> (size(s)=w1027:i32)
                n498 = Decrement(x=w1027) -> (x-1=w1026:i32)
              }
              frame True {
                n499 = Unbundle By Name(w1041) -> ("Numeric Control"=w1045:dbl, "Numeric Control 2"=w1039:dbl)
                n500 = Unbundle By Name(w1046) -> ("Wavlength"=w1034:dbl[unit][])
                n501 = node(w1045) -> (w1044:dbl[unit])
                n502 = node(w1039) -> (w1038:dbl[unit])
                n503 = Subtract(x=w1034, y=w1038) -> (x-y=w1037:dbl[unit][])
                n504 = Subtract(x=w1034, y=w1044) -> (x-y=w1043:dbl[unit][])
                n505 = Absolute Value(x=w1037) -> (abs(x)=w1036:dbl[unit][])
                n506 = Absolute Value(x=w1043) -> (abs(x)=w1042:dbl[unit][])
                n507 = Array Max & Min(array=w1036) -> (min index (indices)=w1033:i32)  [unwired: 3 out]
                n508 = Array Max & Min(array=w1042) -> (min index (indices)=w1032:i32)  [unwired: 3 out]
                n509 = Subtract(x=w1033, y=w1032) -> (x-y=w1031:i32)
                n510 = Index Array(array=w1034, index=w1033) -> (element=w1035:dbl[unit])
                n511 = Index Array(array=w1034, index=w1032) -> (element=w1040:dbl[unit])
                n512 = Increment(x=w1031) -> (x+1=w1030:i32)
                n513 = Array Subset(array=w1034, index=w1032, length=w1030) -> (w1029:dbl[unit][])
                n514 = property on="Wl \nLow" class="DigNum (strict)"("Value"=w1040) -> ()  [unwired: 2 in, 2 out]
                n515 = property on="Wl \nUp" class="DigNum (strict)"("Value"=w1035) -> ()  [unwired: 2 in, 2 out]
              }
            }
            "LowerWLLimit" <- w1019
            "UpperWLLimit" <- w1018
            n516 = Bundle By Name(cluster=w1017, "Wavlength Trim"=w1015) -> (w1016:T5)
          }
        }
      }
      frame Error {
        w1052 = T19 4 items=["no dialog", "OK message", "continue or stop message", "OK message + warnings", "continue/stop + warnings"] ("type of dialog (OK msg:1)")
        n517 = call <vilib>:"General Error Handler.vi"("type of dialog (OK msg:1)"=w1052, "error in (no error)"=w1049) -> ("error out"=w1051:errorcluster)  [unwired: 9 in, 4 out]
        n518 = call <vilib>:"Clear Errors.vi"("error in (no error)"=w1051) -> ("error out"=w1048:errorcluster)  [unwired: 5 in, 1 out]
      }
    }
  }
  n519 = while {
    shift-right: [w1055] -> _
    shift-left: w12 -> [w1053]
    shift-right: [w1058] -> _
    shift-left: w8 -> [w1059]
    shift-right: [w1056] -> _
    shift-left: w1 -> [w1057]
    stop <- w1054 stop-if-true
    # "Producer"
    n520 = event shown="[20] \"StartMeasurement_Button\": Value Change" {
      selector: _ -> [_ _ _ _ _ _ _ _ _ _ _ _ _ _ _ _ _ _ _ _ _ _ _ _ _ _ _ _ _ _ _ _ _]
      dyn-events: _ -> [_ _ _ _ _ _ _ _ _ _ _ _ _ _ _ _ _ _ _ _ _ _ _ _ _ _ _ _ _ _ _ _ _]
      timeout: -1 -> [_ _ _ _ _ _ _ _ _ _ _ _ _ _ _ _ _ _ _ _ _ _ _ _ _ _ _ _ _ _ _ _ _]
      tunnel: w1059 -> [w1062 w1077 w1085 w1098 w1113 w1130 w1135 w1150 w1154 w1163 w1175 w1190 w1214 w1218 w1221 w1225 w1234 w1284 w1289 w1333 w1342 w1367 w1376 w1385 w1393 w1399 w1413 w1440 w1457 w1463 w1478 w1519 w1525]
      tunnel: [w1062 w1074 w1084 w1098 w1113 w1130 w1135 w1150 w1154 w1163 w1175 w1190 w1214 w1218 w1221 w1225 w1234 w1284 w1289 w1333 w1341 w1367 w1376 w1385 w1393 w1399 w1411 w1438 w1457 w1463 w1478 w1518 w1525] -> w1058
      tunnel: w1057 -> [w1061 w1076 w1088 w1096 w1110 w1129 w1134 w1147 w1155 w1164 w1176 w1188 w1209 w1217 w1222 w1224 w1231 w1249 w1288 w1325 w1346 w1366 w1375 w1384 w1392 w1398 w1416 w1444 w1458 w1462 w1476 w1511 w1524]
      tunnel: [w1061 w1070 w1079 w1092 w1109 w1127 w1134 w1146 w1156 w1165 w1177 w1186 w1208 w1217 w1222 w1224 w1229 w1266 w1286 w1309 w1340 w1361 w1372 w1381 w1392 w1398 w1416 w1444 w1458 w1462 w1473 w1511 w1523] -> w1056
      tunnel: w1053 -> [w1063 w1078 w1089 w1097 w1112 w1131 w1136 w1149 w1158 w1167 w1179 w1189 w1211 w1219 w1220 w1226 w1232 w1272 w1290 w1326 w1348 w1368 w1377 w1386 w1394 w1400 w1409 w1445 w1456 w1464 w1477 w1522 w1527]
      tunnel: [w1063 w1075 w1087 w1093 w1111 w1128 w1136 w1148 w1157 w1166 w1178 w1187 w1210 w1219 w1220 w1226 w1233 w1265 w1287 w1308 w1347 w1362 w1373 w1382 w1394 w1397 w1404 w1443 w1456 w1464 w1474 w1522 w1526] -> w1055
      tunnel: [_ TRUE _ _ _ _ _ _ _ _ _ _ _ _ _ _ _ _ _ _ _ _ _ _ _ _ _ _ _ _ _ _ _] -> w1054
      event Timeout {
        n521 = event-data() -> ()  [unwired: 1 in, 3 out]
      }
      event "Stop Button": Value Change {
        w1066 = T8 {"QueueAction"=enum."TimeOut", "Data"=[], "Data_Raw"=[], "Data_Dark"=[], "Data_Ref"=[], "Device Information"=[], "Numeric Control"=0.0, "Boolean"=FALSE, "Wavelength"=[], "Time"=[], "Time Stamp"=timestamp(0 s since 1904-01-01), "Numeric Control 2"=0.0, "TabControl"=enum."Measure", "Numeric Control 3"=0.0}  # DataQueue
        w1069 = T11 {"QueueAction"=enum."TimeOut", "Numeric 1"=0.0, "Numeric 2"=0.0, "Boolean 1"=FALSE, "Boolean 2"=FALSE, "Spin Program"=[], "Spin Prg v07"=[], "Time Stamp"=timestamp(0 s since 1904-01-01), "TabControl"=enum."Measure"}  # Device Queue
        n522 = event-data() -> ()  [unwired: 1 in, 6 out]
        n523 = Bundle By Name(cluster=w1069, "QueueAction"=DeviceQueue_Action."Close_Program") -> (w1067:T11)
        n524 = Enqueue Element At Opposite End(queue=w1078, element=w1067, error in (no error)=w1076) -> (queue out=w1075:refnum<queue>, error out=w1071:errorcluster)  [unwired: 1 in, 1 out]
        n525 = Bundle By Name(cluster=w1066, "QueueAction"=DataQueue_Action."Close_Program") -> (w1064:T8)
        n526 = Enqueue Element At Opposite End(queue=w1077, element=w1064, error in (no error)=w1076) -> (queue out=w1074:refnum<queue>, error out=w1072:errorcluster)  [unwired: 1 in, 1 out]
        n527 = Merge Errors(w1072, w1071) -> (w1070:errorcluster)
      }
      event "Abort Button": Value Change {
        w1083 = T8 {"QueueAction"=enum."TimeOut", "Data"=[], "Data_Raw"=[], "Data_Dark"=[], "Data_Ref"=[], "Device Information"=[], "Numeric Control"=0.0, "Boolean"=FALSE, "Wavelength"=[], "Time"=[], "Time Stamp"=timestamp(0 s since 1904-01-01), "Numeric Control 2"=0.0, "TabControl"=enum."Measure", "Numeric Control 3"=0.0}  # DataQueue
        w1091 = T11 {"QueueAction"=enum."TimeOut", "Numeric 1"=0.0, "Numeric 2"=0.0, "Boolean 1"=FALSE, "Boolean 2"=FALSE, "Spin Program"=[], "Spin Prg v07"=[], "Time Stamp"=timestamp(0 s since 1904-01-01), "TabControl"=enum."Measure"}  # Device Queue
        n528 = event-data() -> ()  [unwired: 1 in, 6 out]
        n529 = Bundle By Name(cluster=w1091, "QueueAction"=DeviceQueue_Action."Abort") -> (w1090:T11)
        n530 = Bundle By Name(cluster=w1083, "QueueAction"=DataQueue_Action."Abort") -> (w1081:T8)
        n531 = Enqueue Element At Opposite End(queue=w1089, element=w1090, error in (no error)=w1088) -> (queue out=w1087:refnum<queue>, error out=w1080:errorcluster)  [unwired: 1 in, 1 out]
        n532 = Enqueue Element At Opposite End(queue=w1085, element=w1081, error in (no error)=w1080) -> (queue out=w1084:refnum<queue>, error out=w1079:errorcluster)  [unwired: 1 in, 1 out]
      }
      event "Init_Spectrometer": Value Change {
        n533 = event-data() -> ()  [unwired: 1 in, 6 out]
        n534 = case shown="False" "Init_Spectrometer" {
          tunnel: [w1100 w1103] -> w1094
          frame True {
            n535 = property on="Tab Control" class="TabCtl (strict)"() -> ("Value"=w1099:T1)  [unwired: 2 in, 2 out]
            n536 = Bundle By Name(cluster=T11 {"QueueAction"=enum."TimeOut", "Numeric 1"=0.0, "Numeric 2"=0.0, "Boolean 1"=FALSE, "Boolean 2"=FALSE, "Spin Program"=[], "Spin Prg v07"=[], "Time Stamp"=timestamp(0 s since 1904-01-01), "TabControl"=enum."Measure"} ("element"), "QueueAction"=DeviceQueue_Action."Spectrometer_Init", "TabControl"=w1099) -> (w1100:T11)
          }
          frame False {
            n537 = Bundle By Name(cluster=T11 {"QueueAction"=enum."TimeOut", "Numeric 1"=0.0, "Numeric 2"=0.0, "Boolean 1"=FALSE, "Boolean 2"=FALSE, "Spin Program"=[], "Spin Prg v07"=[], "Time Stamp"=timestamp(0 s since 1904-01-01), "TabControl"=enum."Measure"} ("element"), "QueueAction"=DeviceQueue_Action."Spectrometer_Close") -> (w1103:T11)
          }
        }
        n538 = Enqueue Element(queue=w1097, element=w1094, error in (no error)=w1096) -> (queue out=w1093:refnum<queue>, error out=w1092:errorcluster)  [unwired: 1 in, 1 out]
      }
      event "Init_Arduino": Value Change {
        # "Shutter is closed after init"
        n539 = event-data() -> ("NewVal"=w1108:bool)  [unwired: 1 in, 5 out]
        n540 = case shown="True" w1108 {
          tunnel: [w1114 w1117] -> w1107
          frame False {
            w1116 = T11 {"QueueAction"=enum."TimeOut", "Numeric 1"=0.0, "Numeric 2"=0.0, "Boolean 1"=FALSE, "Boolean 2"=FALSE, "Spin Program"=[], "Spin Prg v07"=[], "Time Stamp"=timestamp(0 s since 1904-01-01), "TabControl"=enum."Measure"}  # Device Queue
            n541 = Bundle By Name(cluster=w1116, "QueueAction"=DeviceQueue_Action."Arduino_Close") -> (w1114:T11)
          }
          frame True {
            w1119 = T11 {"QueueAction"=enum."TimeOut", "Numeric 1"=0.0, "Numeric 2"=0.0, "Boolean 1"=FALSE, "Boolean 2"=FALSE, "Spin Program"=[], "Spin Prg v07"=[], "Time Stamp"=timestamp(0 s since 1904-01-01), "TabControl"=enum."Measure"}  # Device Queue
            n542 = Bundle By Name(cluster=w1119, "QueueAction"=DeviceQueue_Action."Arduino_Init") -> (w1117:T11)
          }
        }
        n543 = property on="Shutter Toggle" class="Bool (strict)"("Value"=FALSE ("Shutter Toggle")) -> ()  [unwired: 2 in, 2 out]
        n544 = Enqueue Element(queue=w1112, element=w1107, error in (no error)=w1110) -> (queue out=w1111:refnum<queue>, error out=w1109:errorcluster)  [unwired: 1 in, 1 out]
      }
      event "Program Spin Coater": Value Change {
        w1133 = T11 {"QueueAction"=enum."TimeOut", "Numeric 1"=0.0, "Numeric 2"=0.0, "Boolean 1"=FALSE, "Boolean 2"=FALSE, "Spin Program"=[], "Spin Prg v07"=[], "Time Stamp"=timestamp(0 s since 1904-01-01), "TabControl"=enum."Measure"}  # Device Queue
        n545 = event-data() -> ("NewVal"=w1122:T2)  [unwired: 1 in, 5 out]
        n546 = property on="Seconds to Spin_Normal" class="DigNum (strict)"() -> ("Value"=w1124:dbl[unit])  [unwired: 2 in, 2 out]
        n547 = property on="Spin Time" class="DigNum (strict)"() -> ("Value"=w1121:dbl[unit])  [unwired: 2 in, 2 out]
        n548 = node(w1121) -> (w1120:dbl)
        n549 = node(w1124) -> (w1123:dbl)
        n550 = Bundle By Name(cluster=w1133, "QueueAction"=DeviceQueue_Action."Arduino_LoadProgram", "Spin Prg v07"=w1122, "Numeric 1"=w1123, "Numeric 2"=w1120) -> (w1132:T11)
        n551 = Enqueue Element(queue=w1131, element=w1132, error in (no error)=w1129) -> (queue out=w1128:refnum<queue>, error out=w1127:errorcluster)  [unwired: 1 in, 1 out]
        n552 = property on="Measure_IntegrationTime" class="DigNum (strict)"() -> ("Value"=w1125:dbl[unit])  [unwired: 2 in, 2 out]
        n553 = property on="Measure_IntegrationTime" class="DigNum (strict)"("Val(Sgnl)"=w1125) -> ()  [unwired: 2 in, 2 out]
      }
      event "SHUTTER DEBUG": Value Change {
        n554 = event-data() -> ("NewVal"=w1138:bool)  [unwired: 1 in, 5 out]
        n555 = Select(t=u8 0, s=w1138, f=u8 2) -> (s? t:f=w1137:u8)
        n556 = property on="Shutter Position" class="DigNum (strict)"("DisabledEnum"=w1137) -> ()  [unwired: 2 in, 2 out]
        n557 = property on="Shutter Close" class="Bool (strict)"("DisabledEnum"=w1137) -> ()  [unwired: 2 in, 2 out]
        n558 = property on="Shutter Open" class="Bool (strict)"("DisabledEnum"=w1137) -> ()  [unwired: 2 in, 2 out]
      }
      event "Shutter Position": Value Change {
        w1145 = FALSE ("Shutter Close")
        w1143 = T11 {"QueueAction"=enum."TimeOut", "Numeric 1"=0.0, "Numeric 2"=0.0, "Boolean 1"=FALSE, "Boolean 2"=FALSE, "Spin Program"=[], "Spin Prg v07"=[], "Time Stamp"=timestamp(0 s since 1904-01-01), "TabControl"=enum."Measure"}  # Device Queue
        (unwired) DeviceQueue_Action."Arduino_SetSpeed" ("QueueAction")
        (unwired) T11 {"QueueAction"=enum."TimeOut", "Numeric 1"=0.0, "Numeric 2"=0.0, "Boolean 1"=FALSE, "Boolean 2"=FALSE, "Spin Program"=[], "Spin Prg v07"=[], "Time Stamp"=timestamp(0 s since 1904-01-01), "TabControl"=enum."Measure"}  # Device Queue
        n559 = event-data() -> ("NewVal"=w1141:u16)  [unwired: 1 in, 5 out]
        n560 = property on="Shutter Close" class="Bool (strict)"("Value"=w1145) -> ()  [unwired: 2 in, 2 out]
        n561 = property on="Shutter Open" class="Bool (strict)"("Value"=w1145) -> ()  [unwired: 2 in, 2 out]
        n562 = Bundle By Name(cluster=w1143, "QueueAction"=DeviceQueue_Action."Arduino_Shutter_SetPosition", "Numeric 1"=w1141) -> (w1144:T11)
        n563 = Enqueue Element(queue=w1149, element=w1144, error in (no error)=w1147) -> (queue out=w1148:refnum<queue>, error out=w1146:errorcluster)  [unwired: 1 in, 1 out]
      }
      event "Shutter Close": Value Change {
        w1153 = T11 {"QueueAction"=enum."TimeOut", "Numeric 1"=0.0, "Numeric 2"=0.0, "Boolean 1"=FALSE, "Boolean 2"=FALSE, "Spin Program"=[], "Spin Prg v07"=[], "Time Stamp"=timestamp(0 s since 1904-01-01), "TabControl"=enum."Measure"}  # Device Queue
        (unwired) DeviceQueue_Action."Arduino_SetSpeed" ("QueueAction")
        (unwired) T11 {"QueueAction"=enum."TimeOut", "Numeric 1"=0.0, "Numeric 2"=0.0, "Boolean 1"=FALSE, "Boolean 2"=FALSE, "Spin Program"=[], "Spin Prg v07"=[], "Time Stamp"=timestamp(0 s since 1904-01-01), "TabControl"=enum."Measure"}  # Device Queue
        n564 = event-data() -> ()  [unwired: 1 in, 6 out]
        n565 = property on="Shutter Open" class="Bool (strict)"("Value"=FALSE ("Shutter Open")) -> ()  [unwired: 2 in, 2 out]
        n566 = Bundle By Name(cluster=w1153, "QueueAction"=DeviceQueue_Action."Arduino_Shutter_Close") -> (w1152:T11)
        n567 = Enqueue Element(queue=w1158, element=w1152, error in (no error)=w1155) -> (queue out=w1157:refnum<queue>, error out=w1156:errorcluster)  [unwired: 1 in, 1 out]
      }
      event "Shutter Open": Value Change {
        w1162 = T11 {"QueueAction"=enum."TimeOut", "Numeric 1"=0.0, "Numeric 2"=0.0, "Boolean 1"=FALSE, "Boolean 2"=FALSE, "Spin Program"=[], "Spin Prg v07"=[], "Time Stamp"=timestamp(0 s since 1904-01-01), "TabControl"=enum."Measure"}  # Device Queue
        (unwired) DeviceQueue_Action."Arduino_SetSpeed" ("QueueAction")
        (unwired) T11 {"QueueAction"=enum."TimeOut", "Numeric 1"=0.0, "Numeric 2"=0.0, "Boolean 1"=FALSE, "Boolean 2"=FALSE, "Spin Program"=[], "Spin Prg v07"=[], "Time Stamp"=timestamp(0 s since 1904-01-01), "TabControl"=enum."Measure"}  # Device Queue
        n568 = event-data() -> ()  [unwired: 1 in, 6 out]
        n569 = property on="Shutter Close" class="Bool (strict)"("Value"=FALSE ("Shutter Open")) -> ()  [unwired: 2 in, 2 out]
        n570 = Bundle By Name(cluster=w1162, "QueueAction"=DeviceQueue_Action."Arduino_Shutter_Open") -> (w1161:T11)
        n571 = Enqueue Element(queue=w1167, element=w1161, error in (no error)=w1164) -> (queue out=w1166:refnum<queue>, error out=w1165:errorcluster)  [unwired: 1 in, 1 out]
      }
      event "Shutter Toggle": Value Change {
        w1174 = T11 {"QueueAction"=enum."TimeOut", "Numeric 1"=0.0, "Numeric 2"=0.0, "Boolean 1"=FALSE, "Boolean 2"=FALSE, "Spin Program"=[], "Spin Prg v07"=[], "Time Stamp"=timestamp(0 s since 1904-01-01), "TabControl"=enum."Measure"}  # Device Queue
        (unwired) T11 {"QueueAction"=enum."TimeOut", "Numeric 1"=0.0, "Numeric 2"=0.0, "Boolean 1"=FALSE, "Boolean 2"=FALSE, "Spin Program"=[], "Spin Prg v07"=[], "Time Stamp"=timestamp(0 s since 1904-01-01), "TabControl"=enum."Measure"}  # Device Queue
        n572 = event-data() -> ("NewVal"=w1172:bool)  [unwired: 1 in, 5 out]
        n573 = Select(t=DeviceQueue_Action."Arduino_Shutter_Open" ("QueueAction"), s=w1172, f=DeviceQueue_Action."Arduino_Shutter_Close" ("QueueAction")) -> (s? t:f=w1169:T12)
        n574 = Bundle By Name(cluster=w1174, "QueueAction"=w1169) -> (w1173:T11)
        n575 = Enqueue Element(queue=w1179, element=w1173, error in (no error)=w1176) -> (queue out=w1178:refnum<queue>, error out=w1177:errorcluster)  [unwired: 1 in, 1 out]
      }
      event "Measure_IntegrationTime", "SpectralStability_IntegrationTime": Value Change {
        w1192 = T11 {"QueueAction"=enum."TimeOut", "Numeric 1"=0.0, "Numeric 2"=0.0, "Boolean 1"=FALSE, "Boolean 2"=FALSE, "Spin Program"=[], "Spin Prg v07"=[], "Time Stamp"=timestamp(0 s since 1904-01-01), "TabControl"=enum."Measure"}  # Device Queue
        n576 = event-data() -> ("NewVal"=w1184:dbl[unit])  [unwired: 1 in, 5 out]
        n577 = property on="Calculate Frames_Normal" class="Bool (strict)"() -> ("Value"=w1180:bool)  [unwired: 2 in, 2 out]
        n578 = node(w1184) -> (w1183:dbl)
        n579 = property on="Tab Control" class="TabCtl (strict)"() -> ("Value"=w1182:T1)  [unwired: 2 in, 2 out]
        n580 = property on="Tab Control" class="TabCtl (strict)"() -> ("Value"=w1181:T1)  [unwired: 2 in, 2 out]
        n581 = case shown="\"Measure\"" w1182 {
          tunnel: w1192 -> [w1193 w1199 w1205]
          tunnel: [w1193 w1196 w1202] -> w1191
          tunnel: DeviceQueue_Action."Spectrometer_SetIntegrationTime" ("QueueAction") -> [_ w1198 w1204]
          tunnel: w1183 -> [_ w1197 w1203]
          tunnel: w1181 -> [_ w1195 w1200]
          tunnel: w1180 -> [_ w1194 _]
          frame Default {
          }
          frame "Measure" {
            n582 = Bundle By Name(cluster=w1199, "QueueAction"=w1198, "Numeric 1"=w1197, "Boolean 1"=w1194, "TabControl"=w1195) -> (w1196:T11)
          }
          frame "Spectral Stability" {
            n583 = Bundle By Name(cluster=w1205, "QueueAction"=w1204, "Numeric 1"=w1203, "Boolean 1"=FALSE, "TabControl"=w1200) -> (w1202:T11)
          }
        }
        n584 = Enqueue Element(queue=w1189, element=w1191, error in (no error)=w1188) -> (queue out=w1187:refnum<queue>, error out=w1186:errorcluster)  [unwired: 1 in, 1 out]
      }
      event "Frames": Value Change {
        w1213 = T11 {"QueueAction"=enum."TimeOut", "Numeric 1"=0.0, "Numeric 2"=0.0, "Boolean 1"=FALSE, "Boolean 2"=FALSE, "Spin Program"=[], "Spin Prg v07"=[], "Time Stamp"=timestamp(0 s since 1904-01-01), "TabControl"=enum."Measure"}  # Device Queue
        n585 = event-data() -> ()  [unwired: 1 in, 6 out]
        n586 = Bundle By Name(cluster=w1213, "QueueAction"=DeviceQueue_Action."Spectrometer_SetFrames", "Numeric 1"="Frames") -> (w1212:T11)
        n587 = Enqueue Element(queue=w1211, element=w1212, error in (no error)=w1209) -> (queue out=w1210:refnum<queue>, error out=w1208:errorcluster)  [unwired: 1 in, 1 out]
      }
      event "Seconds to Spin_Normal", "Seconds to Spin_Short": Value Change {
        n588 = event-data() -> ("NewVal"=w1215:dbl[unit])  [unwired: 1 in, 5 out]
        n589 = property on="Seconds to Spin_Short" class="DigNum (strict)"("Value"=w1215) -> ()  [unwired: 2 in, 2 out]
        n590 = property on="Seconds to Spin_Normal" class="DigNum (strict)"("Value"=w1215) -> ()  [unwired: 2 in, 2 out]
        n591 = property on="Program Spin Coater" class="Arr (strict)"() -> ("Value"=w1216:T2)  [unwired: 2 in, 2 out]
        n592 = property on="Program Spin Coater" class="Arr (strict)"("Val(Sgnl)"=w1216) -> ()  [unwired: 2 in, 2 out]
      }
      event "Spin Time": Value Change {
        n593 = event-data() -> ()  [unwired: 1 in, 6 out]
        n594 = property on="Program Spin Coater" class="Arr (strict)"() -> ("Value"=w1223:T2)  [unwired: 2 in, 2 out]
        n595 = property on="Program Spin Coater" class="Arr (strict)"("Val(Sgnl)"=w1223) -> ()  [unwired: 2 in, 2 out]
      }
      event "Seconds after Spin": Value Change {
        n596 = event-data() -> ()  [unwired: 1 in, 6 out]
        n597 = property on="Measure_IntegrationTime" class="DigNum (strict)"() -> ("Value"=w1227:dbl[unit])  [unwired: 2 in, 2 out]
        n598 = property on="Measure_IntegrationTime" class="DigNum (strict)"("Val(Sgnl)"=w1227) -> ()  [unwired: 2 in, 2 out]
      }
      event "Calculate Frames_Normal", "Calculate Frames_Short": Value Change {
        n599 = event-data() -> ("NewVal"=w1228:bool)  [unwired: 1 in, 5 out]
        n600 = case shown="False" w1228 {
          tunnel: [0 2] -> w1230
          tunnel: w1232 -> [w1236 w1245]
          tunnel: [w1236 w1243] -> w1233
          tunnel: w1231 -> [w1235 w1242]
          tunnel: [w1235 w1238] -> w1229
          frame False {
          }
          frame True {
            w1244 = T11 {"QueueAction"=enum."TimeOut", "Numeric 1"=0.0, "Numeric 2"=0.0, "Boolean 1"=FALSE, "Boolean 2"=FALSE, "Spin Program"=[], "Spin Prg v07"=[], "Time Stamp"=timestamp(0 s since 1904-01-01), "TabControl"=enum."Measure"}  # Device Queue
            n601 = property on="Measure_IntegrationTime" class="DigNum (strict)"() -> ("Value"=w1240:dbl[unit])  [unwired: 2 in, 2 out]
            n602 = node(w1240) -> (w1239:dbl)
            n603 = Bundle By Name(cluster=w1244, "QueueAction"=DeviceQueue_Action."Spectrometer_SetIntegrationTime", "Numeric 1"=w1239) -> (w1246:T11)
            n604 = Enqueue Element(queue=w1245, element=w1246, error in (no error)=w1242) -> (queue out=w1243:refnum<queue>, error out=w1238:errorcluster)  [unwired: 1 in, 1 out]
          }
        }
        n605 = property on="Calculate Frames_Short" class="Bool (strict)"("Value"=w1228) -> ()  [unwired: 2 in, 2 out]
        n606 = property on="Calculate Frames_Normal" class="Bool (strict)"("Value"=w1228) -> ()  [unwired: 2 in, 2 out]
        n607 = property on="Frames" class="DigNum (strict)"("DisabledEnum"=w1230) -> ()  [unwired: 2 in, 2 out]
      }
      event "Record RefSpec": Value Change {
        w1253 = T11 {"QueueAction"=enum."TimeOut", "Numeric 1"=0.0, "Numeric 2"=0.0, "Boolean 1"=FALSE, "Boolean 2"=FALSE, "Spin Program"=[], "Spin Prg v07"=[], "Time Stamp"=timestamp(0 s since 1904-01-01), "TabControl"=enum."Measure"}  # Device Queue
        n608 = event-data() -> ()  [unwired: 1 in, 6 out]
        n609 = property on="Shutter Toggle" class="Bool (strict)"("Value"=FALSE ("Shutter Toggle")) -> ()  [unwired: 2 in, 2 out]
        n610 = property on="Frames for Ref/Dark" class="DigNum (strict)"() -> ("Value"=w1262:dbl)  [unwired: 2 in, 2 out]
        n611 = property on="Measure_FramesSpectrometer" class="DigNum (strict)"() -> ("Value"=w1257:dbl)  [unwired: 2 in, 2 out]
        n612 = Bundle By Name(cluster=w1253, "QueueAction"=DeviceQueue_Action."Spectrometer_SetTriggerMode", "Numeric 1"=0.0) -> (w1252:T11)
        n613 = Bundle By Name(cluster=w1252, "QueueAction"=DeviceQueue_Action."Arduino_Shutter_Open") -> (w1248:T11)
        n614 = Bundle By Name(cluster=w1248, "QueueAction"=DeviceQueue_Action."Wait", "Numeric 1"=0.5) -> (w1263:T11)
        n615 = Enqueue Element(queue=w1272, element=w1252, error in (no error)=w1249) -> (queue out=w1254:refnum<queue>, error out=w1250:errorcluster)  [unwired: 1 in, 1 out]
        n616 = Bundle By Name(cluster=w1263, "QueueAction"=DeviceQueue_Action."Spectrometer_SetFrames", "Numeric 1"=w1262) -> (w1261:T11)
        n617 = Enqueue Element(queue=w1254, element=w1248, error in (no error)=w1250) -> (queue out=w1278:refnum<queue>, error out=w1275:errorcluster)  [unwired: 1 in, 1 out]
        n618 = Bundle By Name(cluster=w1261, "QueueAction"=DeviceQueue_Action."Spectrometer_SetReference") -> (w1260:T11)
        n619 = Enqueue Element(queue=w1278, element=w1263, error in (no error)=w1275) -> (queue out=w1277:refnum<queue>, error out=w1274:errorcluster)  [unwired: 1 in, 1 out]
        n620 = Bundle By Name(cluster=w1260, "QueueAction"=DeviceQueue_Action."Arduino_Shutter_Close") -> (w1258:T11)
        n621 = Enqueue Element(queue=w1277, element=w1261, error in (no error)=w1274) -> (queue out=w1276:refnum<queue>, error out=w1273:errorcluster)  [unwired: 1 in, 1 out]
        n622 = Bundle By Name(cluster=w1258, "QueueAction"=DeviceQueue_Action."Spectrometer_SetFrames", "Numeric 1"=w1257) -> (w1256:T11)
        n623 = Enqueue Element(queue=w1276, element=w1260, error in (no error)=w1273) -> (queue out=w1269:refnum<queue>, error out=w1270:errorcluster)  [unwired: 1 in, 1 out]
        n624 = Enqueue Element(queue=w1269, element=w1258, error in (no error)=w1270) -> (queue out=w1267:refnum<queue>, error out=w1268:errorcluster)  [unwired: 1 in, 1 out]
        n625 = Enqueue Element(queue=w1267, element=w1256, error in (no error)=w1268) -> (queue out=w1265:refnum<queue>, error out=w1266:errorcluster)  [unwired: 1 in, 1 out]
      }
      event "Measure_Preview", "SpectralStability_Preview": Value Change {
        n626 = event-data() -> ("NewVal"=w1285:bool)  [unwired: 1 in, 5 out]
        n627 = case shown="False" w1285 {
          tunnel: w1290 -> [w1292 w1297]
          tunnel: w1288 -> [w1291 w1296]
          tunnel: [w1292 w1295] -> w1287
          tunnel: [w1291 w1294] -> w1286
          frame False {
          }
          frame True {
            w1300 = T11 {"QueueAction"=enum."TimeOut", "Numeric 1"=0.0, "Numeric 2"=0.0, "Boolean 1"=FALSE, "Boolean 2"=FALSE, "Spin Program"=[], "Spin Prg v07"=[], "Time Stamp"=timestamp(0 s since 1904-01-01), "TabControl"=enum."Measure"}  # Device Queue
            n628 = property on="Tab Control" class="TabCtl (strict)"() -> ("Value"=w1293:T1)  [unwired: 2 in, 2 out]
            n629 = Bundle By Name(cluster=w1300, "QueueAction"=DeviceQueue_Action."Spectrometer_Preview", "TabControl"=w1293) -> (w1299:T11)
            n630 = Enqueue Element(queue=w1297, element=w1299, error in (no error)=w1296) -> (queue out=w1295:refnum<queue>, error out=w1294:errorcluster)  [unwired: 1 in, 1 out]
          }
        }
      }
      event "Measure:\nRecord_Darkspec", "SpectralStability:\nRecord_Darkspec": Value Change {
        w1331 = T11 {"QueueAction"=enum."TimeOut", "Numeric 1"=0.0, "Numeric 2"=0.0, "Boolean 1"=FALSE, "Boolean 2"=FALSE, "Spin Program"=[], "Spin Prg v07"=[], "Time Stamp"=timestamp(0 s since 1904-01-01), "TabControl"=enum."Measure"}  # Device Queue
        n631 = event-data() -> ()  [unwired: 1 in, 6 out]
        n632 = property on="Shutter Toggle" class="Bool (strict)"("Value"=FALSE ("Shutter Toggle")) -> ()  [unwired: 2 in, 2 out]
        n633 = property on="Frames for Ref/Dark" class="DigNum (strict)"() -> ("Value"=w1316:dbl)  [unwired: 2 in, 2 out]
        n634 = property on="Measure_FramesSpectrometer" class="DigNum (strict)"() -> ("Value"=w1310:dbl)  [unwired: 2 in, 2 out]
        n635 = Bundle By Name(cluster=w1331, "QueueAction"=DeviceQueue_Action."Arduino_Shutter_Close") -> (w1306:T11)
        n636 = Bundle By Name(cluster=w1306, "QueueAction"=DeviceQueue_Action."Spectrometer_SetTriggerMode", "Numeric 1"=0.0) -> (w1305:T11)
        n637 = Bundle By Name(cluster=w1305, "QueueAction"=DeviceQueue_Action."Wait", "Numeric 1"=0.5) -> (w1330:T11)
        n638 = Bundle By Name(cluster=w1330, "QueueAction"=DeviceQueue_Action."Spectrometer_SetFrames", "Numeric 1"=w1316) -> (w1314:T11)
        n639 = Enqueue Element(queue=w1326, element=w1306, error in (no error)=w1325) -> (queue out=w1324:refnum<queue>, error out=w1302:errorcluster)  [unwired: 1 in, 1 out]
        n640 = Bundle By Name(cluster=w1314, "QueueAction"=DeviceQueue_Action."Spectrometer_SetDarkspec") -> (w1312:T11)
        n641 = Enqueue Element(queue=w1324, element=w1305, error in (no error)=w1302) -> (queue out=w1307:refnum<queue>, error out=w1301:errorcluster)  [unwired: 1 in, 1 out]
        n642 = Bundle By Name(cluster=w1312, "QueueAction"=DeviceQueue_Action."Spectrometer_SetFrames", "Numeric 1"=w1310) -> (w1313:T11)
        n643 = Enqueue Element(queue=w1307, element=w1330, error in (no error)=w1301) -> (queue out=w1322:refnum<queue>, error out=w1323:errorcluster)  [unwired: 1 in, 1 out]
        n644 = Enqueue Element(queue=w1322, element=w1314, error in (no error)=w1323) -> (queue out=w1320:refnum<queue>, error out=w1319:errorcluster)  [unwired: 1 in, 1 out]
        n645 = Enqueue Element(queue=w1320, element=w1312, error in (no error)=w1319) -> (queue out=w1318:refnum<queue>, error out=w1317:errorcluster)  [unwired: 1 in, 1 out]
        n646 = Enqueue Element(queue=w1318, element=w1313, error in (no error)=w1317) -> (queue out=w1308:refnum<queue>, error out=w1309:errorcluster)  [unwired: 1 in, 1 out]
      }
      event "StartMeasurement_Button": Value Change {
        w1343 = T8 {"QueueAction"=enum."TimeOut", "Data"=[], "Data_Raw"=[], "Data_Dark"=[], "Data_Ref"=[], "Device Information"=[], "Numeric Control"=0.0, "Boolean"=FALSE, "Wavelength"=[], "Time"=[], "Time Stamp"=timestamp(0 s since 1904-01-01), "Numeric Control 2"=0.0, "TabControl"=enum."Measure", "Numeric Control 3"=0.0}  # DataQueue
        w1350 = T11 {"QueueAction"=enum."TimeOut", "Numeric 1"=0.0, "Numeric 2"=0.0, "Boolean 1"=FALSE, "Boolean 2"=FALSE, "Spin Program"=[], "Spin Prg v07"=[], "Time Stamp"=timestamp(0 s since 1904-01-01), "TabControl"=enum."Measure"}  # Device Queue
        n647 = event-data() -> ()  [unwired: 1 in, 6 out]
        n648 = property on="Measure_Preview" class="Bool (strict)"("Value"=FALSE ("Preview")) -> ()  [unwired: 2 in, 2 out]
        n649 = case shown="\"Normal\", Default" "Tab Control SpinType" {
          tunnel: [DeviceQueue_Action."Measure_InSituAdvanced" ("QueueAction") DeviceQueue_Action."Measure_InSituAdvanced_Short" ("QueueAction")] -> w1336
          tunnel: [DataQueue_Action."Measure_InSituSpinCoating" ("QueueAction") DataQueue_Action."Measure_InSituSpinCoating_Short" ("QueueAction")] -> w1335
          frame "Normal", Default {
            n650 = property on="Motor_ShortStop" class="Bool (strict)"("Value"=FALSE ("Motor_ShortStop")) -> ()  [unwired: 2 in, 2 out]
          }
          frame "Short" {
            n651 = property on="Motor_ShortStop" class="Bool (strict)"("Value"=TRUE ("Motor_ShortStop")) -> ()  [unwired: 2 in, 2 out]
          }
        }
        n652 = Get Date/Time In Seconds() -> (seconds since 1Jan1904=w1338:timestamp)
        n653 = Bundle By Name(cluster=w1350, "QueueAction"=w1336, "Time Stamp"=w1338) -> (w1349:T11)
        n654 = Enqueue Element(queue=w1348, element=w1349, error in (no error)=w1346) -> (queue out=w1347:refnum<queue>, error out=w1339:errorcluster)  [unwired: 1 in, 1 out]
        n655 = property on="Reference\nValue" class="DigNum (strict)"("Value"=1.0 ("Reference\nValue")) -> ()  [unwired: 2 in, 2 out]
        n656 = Bundle By Name(cluster=w1343, "QueueAction"=w1335, "Time Stamp"=w1338) -> (w1344:T8)
        n657 = Enqueue Element(queue=w1342, element=w1344, error in (no error)=w1339) -> (queue out=w1341:refnum<queue>, error out=w1340:errorcluster)  [unwired: 1 in, 1 out]
      }
      event "StartSpin_Button": Value Change {
        w1369 = T11 {"QueueAction"=enum."TimeOut", "Numeric 1"=0.0, "Numeric 2"=0.0, "Boolean 1"=FALSE, "Boolean 2"=FALSE, "Spin Program"=[], "Spin Prg v07"=[], "Time Stamp"=timestamp(0 s since 1904-01-01), "TabControl"=enum."Measure"}  # Device Queue
        n658 = event-data() -> ()  [unwired: 1 in, 6 out]
        n659 = Bundle By Name(cluster=w1369, "QueueAction"=DeviceQueue_Action."Arduino_StartProgram", "Numeric 1"=1.0) -> (w1360:T11)
        n660 = Bundle By Name(cluster=w1360, "QueueAction"=DeviceQueue_Action."Arduino_Shutter_Close") -> (w1358:T11)
        n661 = Enqueue Element(queue=w1368, element=w1360, error in (no error)=w1366) -> (queue out=w1363:refnum<queue>, error out=w1364:errorcluster)  [unwired: 1 in, 1 out]
        n662 = Enqueue Element(queue=w1363, element=w1358, error in (no error)=w1364) -> (queue out=w1362:refnum<queue>, error out=w1361:errorcluster)  [unwired: 1 in, 1 out]
      }
      event "ESC_Milliseconds": Value Change {
        w1378 = T11 {"QueueAction"=enum."TimeOut", "Numeric 1"=0.0, "Numeric 2"=0.0, "Boolean 1"=FALSE, "Boolean 2"=FALSE, "Spin Program"=[], "Spin Prg v07"=[], "Time Stamp"=timestamp(0 s since 1904-01-01), "TabControl"=enum."Measure"}  # Device Queue
        n663 = event-data() -> ()  [unwired: 1 in, 6 out]
        n664 = Bundle By Name(cluster=w1378, "QueueAction"=DeviceQueue_Action."Arduino_SetMillis", "Numeric 1"="ESC_Milliseconds") -> (w1374:T11)
        n665 = Enqueue Element(queue=w1377, element=w1374, error in (no error)=w1375) -> (queue out=w1373:refnum<queue>, error out=w1372:errorcluster)  [unwired: 1 in, 1 out]
      }
      event "ESC_Speed": Value Change {
        w1387 = T11 {"QueueAction"=enum."TimeOut", "Numeric 1"=0.0, "Numeric 2"=0.0, "Boolean 1"=FALSE, "Boolean 2"=FALSE, "Spin Program"=[], "Spin Prg v07"=[], "Time Stamp"=timestamp(0 s since 1904-01-01), "TabControl"=enum."Measure"}  # Device Queue
        n666 = event-data() -> ()  [unwired: 1 in, 6 out]
        n667 = Bundle By Name(cluster=w1387, "QueueAction"=DeviceQueue_Action."Arduino_SetSpeed", "Numeric 1"="ESC_Speed") -> (w1383:T11)
        n668 = Enqueue Element(queue=w1386, element=w1383, error in (no error)=w1384) -> (queue out=w1382:refnum<queue>, error out=w1381:errorcluster)  [unwired: 1 in, 1 out]
      }
      event "ESC DEBUG": Value Change {
        n669 = event-data() -> ()  [unwired: 1 in, 6 out]
        n670 = Select(t=u8 0, s="ESC DEBUG", f=u8 2) -> (s? t:f=w1388:u8)
        n671 = property on="ESC_Milliseconds" class="DigNum (strict)"("DisabledEnum"=w1388) -> ()  [unwired: 2 in, 2 out]
        n672 = property on="ESC_Speed" class="DigNum (strict)"("DisabledEnum"=w1388) -> ()  [unwired: 2 in, 2 out]
      }
      event "Measure_FramesSpectrometer", "SpectralStability_FramesSpectrometer": Value Change {
        w1402 = T11 {"QueueAction"=enum."TimeOut", "Numeric 1"=0.0, "Numeric 2"=0.0, "Boolean 1"=FALSE, "Boolean 2"=FALSE, "Spin Program"=[], "Spin Prg v07"=[], "Time Stamp"=timestamp(0 s since 1904-01-01), "TabControl"=enum."Measure"}  # Device Queue
        n673 = event-data() -> ("NewVal"=w1396:dbl)  [unwired: 1 in, 5 out]
        n674 = property on="Tab Control" class="TabCtl (strict)"() -> ("Value"=w1395:T1)  [unwired: 2 in, 2 out]
        n675 = Bundle By Name(cluster=w1402, "QueueAction"=DeviceQueue_Action."Spectrometer_SetFrames", "Numeric 1"=w1396, "TabControl"=w1395) -> (w1403:T11)
        n676 = Enqueue Element(queue=w1400, element=w1403) -> (queue out=w1397:refnum<queue>)  [unwired: 2 in, 2 out]
      }
      event "Measure_MeasureSpectrum", "SpectralStability_MeasureSpectrum": Value Change {
        w1415 = T8 {"QueueAction"=enum."TimeOut", "Data"=[], "Data_Raw"=[], "Data_Dark"=[], "Data_Ref"=[], "Device Information"=[], "Numeric Control"=0.0, "Boolean"=FALSE, "Wavelength"=[], "Time"=[], "Time Stamp"=timestamp(0 s since 1904-01-01), "Numeric Control 2"=0.0, "TabControl"=enum."Measure", "Numeric Control 3"=0.0}  # DataQueue
        n677 = event-data() -> ()  [unwired: 1 in, 6 out]
        n678 = property on="Tab Control" class="TabCtl (strict)"() -> ("Value"=w1407:T1)  [unwired: 2 in, 2 out]
        n679 = case shown="\"Measure\"" w1407 {
          tunnel: w1409 -> [w1427 w1430]
          tunnel: [w1427 w1429] -> w1408
          tunnel: [w1426 w1428] -> w1406
          frame Default {
            w1426 = T11 {"QueueAction"=enum."TimeOut", "Numeric 1"=0.0, "Numeric 2"=0.0, "Boolean 1"=FALSE, "Boolean 2"=FALSE, "Spin Program"=[], "Spin Prg v07"=[], "Time Stamp"=timestamp(0 s since 1904-01-01), "TabControl"=enum."Measure"}  # Device Queue
          }
          frame "Measure" {
            w1433 = T11 {"QueueAction"=enum."TimeOut", "Numeric 1"=0.0, "Numeric 2"=0.0, "Boolean 1"=FALSE, "Boolean 2"=FALSE, "Spin Program"=[], "Spin Prg v07"=[], "Time Stamp"=timestamp(0 s since 1904-01-01), "TabControl"=enum."Measure"}  # Device Queue
            (unwired) T11 {"QueueAction"=enum."TimeOut", "Numeric 1"=0.0, "Numeric 2"=0.0, "Boolean 1"=FALSE, "Boolean 2"=FALSE, "Spin Program"=[], "Spin Prg v07"=[], "Time Stamp"=timestamp(0 s since 1904-01-01), "TabControl"=enum."Measure"}  # Device Queue
            n680 = Bundle By Name(cluster=w1433, "QueueAction"=DeviceQueue_Action."Spectrometer_SetFrames", "Numeric 1"="Frames for Ref/Dark") -> (w1428:T11)
            n681 = Enqueue Element(queue=w1430, element=w1428) -> (queue out=w1429:refnum<queue>)  [unwired: 2 in, 2 out]
          }
        }
        n682 = Get Date/Time In Seconds() -> (seconds since 1Jan1904=w1410:timestamp)
        n683 = Bundle By Name(cluster=w1406, "QueueAction"=DeviceQueue_Action."Measure_Spectrum", "Time Stamp"=w1410, "TabControl"=w1407) -> (w1418:T11)
        n684 = Enqueue Element(queue=w1408, element=w1418) -> (queue out=w1405:refnum<queue>)  [unwired: 2 in, 2 out]
        n685 = case shown="Default" w1407 {
          tunnel: w1406 -> [_ w1424]
          tunnel: w1405 -> [w1419 w1423]
          tunnel: [w1419 w1422] -> w1404
          frame Default {
          }
          frame "Measure" {
            n686 = property on="Measure_FramesSpectrometer" class="DigNum (strict)"() -> ("Value"=w1421:dbl)  [unwired: 2 in, 2 out]
            n687 = Bundle By Name(cluster=w1424, "QueueAction"=DeviceQueue_Action."Spectrometer_SetFrames", "Numeric 1"=w1421) -> (w1420:T11)
            n688 = Enqueue Element(queue=w1423, element=w1420) -> (queue out=w1422:refnum<queue>)  [unwired: 2 in, 2 out]
          }
        }
        n689 = Bundle By Name(cluster=w1415, "QueueAction"=DataQueue_Action."Measure_Spectrum", "TabControl"=w1407) -> (w1412:T8)
        n690 = Enqueue Element(queue=w1413, element=w1412) -> (queue out=w1411:refnum<queue>)  [unwired: 2 in, 2 out]
      }
      event "SpectralStability_Record": Value Change {
        w1442 = T8 {"QueueAction"=enum."TimeOut", "Data"=[], "Data_Raw"=[], "Data_Dark"=[], "Data_Ref"=[], "Device Information"=[], "Numeric Control"=0.0, "Boolean"=FALSE, "Wavelength"=[], "Time"=[], "Time Stamp"=timestamp(0 s since 1904-01-01), "Numeric Control 2"=0.0, "TabControl"=enum."Measure", "Numeric Control 3"=0.0}  # DataQueue
        w1447 = T11 {"QueueAction"=enum."TimeOut", "Numeric 1"=0.0, "Numeric 2"=0.0, "Boolean 1"=FALSE, "Boolean 2"=FALSE, "Spin Program"=[], "Spin Prg v07"=[], "Time Stamp"=timestamp(0 s since 1904-01-01), "TabControl"=enum."Measure"}  # Device Queue
        n691 = event-data() -> ()  [unwired: 1 in, 6 out]
        n692 = property on="Duration/\nTimes" class="Bool (strict)"() -> ("Value"=w1435:bool)  [unwired: 2 in, 2 out]
        n693 = case shown="False" w1435 {
          tunnel: ["SpectralStability_\nMeasurementNumber" w1450] -> w1434
          frame False {
            # "Number"
          }
          frame True {
            # "Duration"
            n694 = property on="SpectralStability_\nPeriodicTime" class="DigNum (strict)"() -> ("Value"=w1452:dbl[unit])  [unwired: 2 in, 2 out]
            n695 = Divide(x="SpectralStability_Duration", y=w1452) -> (x/y=w1453:dbl)
            n696 = Round Toward +Infinity(x=w1453) -> (ceil(x): smallest int >= x=w1451:dbl)
            n697 = Increment(x=w1451) -> (x+1=w1450:dbl)
          }
        }
        n698 = Get Date/Time In Seconds() -> (seconds since 1Jan1904=w1436:timestamp)
        n699 = property on="Tab Control" class="TabCtl (strict)"() -> ("Value"=w1437:T1)  [unwired: 2 in, 2 out]
        n700 = Bundle By Name(cluster=w1447, "QueueAction"=DeviceQueue_Action."Measure_SpectralStability", "Time Stamp"=w1436, "TabControl"=w1437, "Numeric 1"=w1434) -> (w1448:T11)
        n701 = property on="SS_StepsLeft" class="DigNum (strict)"("Value"=w1434) -> ()  [unwired: 2 in, 2 out]
        n702 = Enqueue Element(queue=w1445, element=w1448) -> (queue out=w1443:refnum<queue>)  [unwired: 2 in, 2 out]
        n703 = Bundle By Name(cluster=w1442, "QueueAction"=DataQueue_Action."Measure_SpectralStability", "TabControl"=w1437, "Time Stamp"=w1436, "Numeric Control"=w1434) -> (w1439:T8)
        n704 = Enqueue Element(queue=w1440, element=w1439) -> (queue out=w1438:refnum<queue>)  [unwired: 2 in, 2 out]
      }
      event "Automatically \nadjust count": Value Change {
        n705 = event-data() -> ("NewVal"=w1461:bool)  [unwired: 1 in, 5 out]
        n706 = Select(t=u8 2, s=w1461, f=u8 0) -> (s? t:f=w1455:u8)
        n707 = property on="Spectra Count" class="DigNum (strict)"("DisabledEnum"=w1455) -> ()  [unwired: 2 in, 2 out]
      }
      event "Duration/Times": Value Change {
        n708 = event-data() -> ("NewVal"=w1467:bool)  [unwired: 1 in, 5 out]
        n709 = case shown="False" w1467 {
          tunnel: [FALSE TRUE] -> w1466
          tunnel: [TRUE FALSE] -> w1465
          frame False {
          }
          frame True {
          }
        }
        n710 = property on="SpectralStability_Duration" class="DigNum (strict)"("Visible"=w1466) -> ()  [unwired: 2 in, 2 out]
        n711 = property on="SpectralStability_\nMeasurementNumber" class="DigNum (strict)"("Visible"=w1465) -> ()  [unwired: 2 in, 2 out]
      }
      event "Tab Control": Value Change {
        w1472 = FALSE ("SpectralStability_Preview")
        n712 = event-data() -> ("NewVal"=w1475:T1)  [unwired: 1 in]
        n713 = case shown="\"Spectral Stability\"" w1475 {
          tunnel: w1477 -> [w1480 w1493 w1508]
          tunnel: [w1480 w1482 w1499] -> w1474
          tunnel: w1476 -> [w1479 w1492 w1507]
          tunnel: w1475 -> [_ w1491 w1506]
          tunnel: [w1479 w1481 w1498] -> w1473
          frame Default {
          }
          frame "Measure" {
            w1495 = T11 {"QueueAction"=enum."TimeOut", "Numeric 1"=0.0, "Numeric 2"=0.0, "Boolean 1"=FALSE, "Boolean 2"=FALSE, "Spin Program"=[], "Spin Prg v07"=[], "Time Stamp"=timestamp(0 s since 1904-01-01), "TabControl"=enum."Measure"}  # Device Queue
            n714 = property on="Measure_IntegrationTime" class="DigNum (strict)"() -> ("Value"=w1490:dbl[unit])  [unwired: 2 in, 2 out]
            n715 = node(w1490) -> (w1489:dbl)
            n716 = Bundle By Name(cluster=w1495, "QueueAction"=DeviceQueue_Action."Spectrometer_SetIntegrationTime", "Numeric 1"=w1489, "TabControl"=w1491) -> (w1486:T11)
            n717 = property on="Measure_FramesSpectrometer" class="DigNum (strict)"() -> ("Value"=w1484:dbl)  [unwired: 2 in, 2 out]
            n718 = Enqueue Element(queue=w1493, element=w1486, error in (no error)=w1492) -> (queue out=w1488:refnum<queue>, error out=w1487:errorcluster)  [unwired: 1 in, 1 out]
            n719 = Bundle By Name(cluster=w1486, "QueueAction"=DeviceQueue_Action."Spectrometer_SetFrames", "Numeric 1"=w1484) -> (w1483:T11)
            n720 = Enqueue Element(queue=w1488, element=w1483, error in (no error)=w1487) -> (queue out=w1482:refnum<queue>, error out=w1481:errorcluster)  [unwired: 1 in, 1 out]
          }
          frame "Spectral Stability" {
            w1510 = T11 {"QueueAction"=enum."TimeOut", "Numeric 1"=0.0, "Numeric 2"=0.0, "Boolean 1"=FALSE, "Boolean 2"=FALSE, "Spin Program"=[], "Spin Prg v07"=[], "Time Stamp"=timestamp(0 s since 1904-01-01), "TabControl"=enum."Measure"}  # Device Queue
            n721 = property on="SpectralStability_IntegrationTime" class="DigNum (strict)"() -> ("Value"=w1497:dbl[unit])  [unwired: 2 in, 2 out]
            n722 = node(w1497) -> (w1505:dbl)
            n723 = property on="SpectralStability_FramesSpectrometer" class="DigNum (strict)"() -> ("Value"=w1496:dbl)  [unwired: 2 in, 2 out]
            n724 = Bundle By Name(cluster=w1510, "QueueAction"=DeviceQueue_Action."Spectrometer_SetIntegrationTime", "Numeric 1"=w1505, "TabControl"=w1506) -> (w1502:T11)
            n725 = Enqueue Element(queue=w1508, element=w1502, error in (no error)=w1507) -> (queue out=w1504:refnum<queue>, error out=w1503:errorcluster)  [unwired: 1 in, 1 out]
            n726 = Bundle By Name(cluster=w1502, "QueueAction"=DeviceQueue_Action."Spectrometer_SetFrames", "Numeric 1"=w1496) -> (w1500:T11)
            n727 = Enqueue Element(queue=w1504, element=w1500, error in (no error)=w1503) -> (queue out=w1499:refnum<queue>, error out=w1498:errorcluster)  [unwired: 1 in, 1 out]
          }
        }
        n728 = property on="SpectralStability_Preview" class="Bool (strict)"("Value"=w1472) -> ()  [unwired: 2 in, 2 out]
        n729 = property on="Measure_Preview" class="Bool (strict)"("Value"=w1472) -> ()  [unwired: 2 in, 2 out]
      }
      event "Trim\nSpec", "Wl \nUp", "Wl \nLow": Value Change {
        w1520 = T8 {"QueueAction"=enum."TimeOut", "Data"=[], "Data_Raw"=[], "Data_Dark"=[], "Data_Ref"=[], "Device Information"=[], "Numeric Control"=0.0, "Boolean"=FALSE, "Wavelength"=[], "Time"=[], "Time Stamp"=timestamp(0 s since 1904-01-01), "Numeric Control 2"=0.0, "TabControl"=enum."Measure", "Numeric Control 3"=0.0}  # DataQueue
        n730 = event-data() -> ()  [unwired: 1 in, 6 out]
        n731 = node("Wl \nLow") -> (w1514:dbl)
        n732 = node("Wl \nUp") -> (w1513:dbl)
        n733 = Bundle By Name(cluster=w1520, "QueueAction"=DataQueue_Action."Change_TrimSettings", "Numeric Control"=w1514, "Numeric Control 2"=w1513, "Boolean"="Trim\nSpec") -> (w1521:T8)
        n734 = Enqueue Element(queue=w1519, element=w1521) -> (queue out=w1518:refnum<queue>)  [unwired: 2 in, 2 out]
      }
      event "Motor_ShortStop": Value Change {
        w1529 = T11 {"QueueAction"=enum."TimeOut", "Numeric 1"=0.0, "Numeric 2"=0.0, "Boolean 1"=FALSE, "Boolean 2"=FALSE, "Spin Program"=[], "Spin Prg v07"=[], "Time Stamp"=timestamp(0 s since 1904-01-01), "TabControl"=enum."Measure"}  # Device Queue
        n735 = event-data() -> ()  [unwired: 1 in, 6 out]
        n736 = Bundle By Name(cluster=w1529, "QueueAction"=DeviceQueue_Action."Arduino_ShortStop") -> (w1528:T11)
        n737 = Enqueue Element At Opposite End(queue=w1527, element=w1528, error in (no error)=w1524) -> (queue out=w1526:refnum<queue>, error out=w1523:errorcluster)  [unwired: 1 in, 1 out]
      }
    }
  }
  n738 = while {
    shift-right: [w1535] -> _
    shift-left: w1 -> [w1539]
    shift-right: [w1536] -> w10
    shift-left: w12 -> [w1538]
    shift-right: [w1533] -> w9
    shift-left: w8 -> [w1534]
    shift-right: [w1531] -> _
    shift-left: w11 -> [w1532]
    stop <- w1537 stop-if-true
    # "Consumer Devices"
    n739 = case shown="No Error" w1539 {
      selector: w1539 -> [w1552 w2446]
      tunnel: w1538 -> [w1553 w2447]
      tunnel: [w1549 _] -> w1537
      tunnel: [w1548 w2447] -> w1536
      tunnel: [w1546 w2443] -> w1535
      tunnel: w1534 -> [w1544 w2441]
      tunnel: [w1545 w2441] -> w1533
      tunnel: w1532 -> [w1543 w2442]
      tunnel: [w1542 w2442] -> w1531
      frame No Error {
        n740 = Dequeue Element(queue=w1553, timeout in ms (-1)=10, error in (no error)=w1552) -> (queue out=w1551:refnum<queue>, element=w1541:T11, error out=w1547:errorcluster)  [unwired: 1 out]
        n741 = Unbundle By Name(w1541) -> ("QueueAction"=w1550:T12)
        n742 = case shown="\"Abort\"" w1550 {
          tunnel: w1551 -> [w1558 w1579 w1620 w1643 w1654 w1709 w1728 w1753 w1764 w1787 w1794 w1813 w1878 w1935 w1966 w1985 w2000 w2010 w2022 w2023 w2045 w2069 w2076 w2083 w2095 w2101 w2107 w2119 w2126 w2133 w2142 w2188 w2283 w2386 w2402 w2412]
          tunnel: [_ _ w1622 _ _ _ _ _ _ _ _ _ _ _ _ _ _ _ _ _ _ _ _ _ _ _ _ _ _ _ _ _ _ _ _ _] -> w1549
          tunnel: [w1558 w1579 w1605 w1630 w1650 w1709 w1728 w1753 w1765 w1787 w1794 w1813 w1878 w1935 w1966 w1985 w2000 w2010 w2022 w2023 w2045 w2069 w2076 w2083 w2095 w2101 w2107 w2119 w2126 w2133 w2142 w2150 w2199 w2346 w2393 w2415] -> w1548
          tunnel: w1547 -> [w1557 w1578 w1604 w1642 w1665 w1710 w1727 w1752 w1760 w1790 w1798 w1810 w1866 w1945 w1964 w1975 w1991 w2007 w2018 w2030 w2048 w2063 w2073 w2081 w2090 w2098 w2104 w2110 w2122 w2129 w2135 w2144 w2244 w2350 w2401 w2411]
          tunnel: [w1557 w1578 w1603 w1624 w1653 w1704 w1726 w1751 w1758 w1788 w1795 w1801 w1820 w1939 w1963 w1970 w1987 w2005 w2012 w2033 w2047 w2060 w2072 w2079 w2089 w2097 w2103 w2109 w2121 w2128 w2134 w2151 w2198 w2339 w2392 w2416] -> w1546
          tunnel: [w1555 w1576 w1602 w1647 w1651 w1706 w1719 w1733 w1769 w1786 w1793 w1804 w1872 w1947 w1967 w1979 w1994 w2001 w2014 w2035 w2046 w2068 w2078 w2087 w2093 w2102 w2108 w2118 w2125 w2132 w2137 w2159 w2256 w2361 w2400 w2432] -> w1545
          tunnel: w1544 -> [w1555 w1576 w1602 w1647 w1652 w1706 w1718 w1742 w1770 w1786 w1793 w1805 w1873 w1947 w1967 w1982 w1997 w2001 w2016 w2035 w2046 w2068 w2078 w2087 w2093 w2102 w2108 w2118 w2125 w2132 w2138 w2159 w2256 w2361 w2400 w2432]
          tunnel: w1543 -> [w1556 w1577 w1601 w1646 w1662 w1708 w1725 w1750 w1763 w1785 w1797 w1806 w1857 w1938 w1960 w1978 w1993 w2004 w2011 w2032 w2041 w2062 w2077 w2086 w2092 w2100 w2106 w2117 w2124 w2131 w2136 w2191 w2286 w2389 w2399 w2431]
          tunnel: [w1556 w1577 w1601 w1646 w1656 w1707 w1725 w1750 w1762 w1783 w1792 w1806 w1857 w1936 w1961 w1977 w1992 w2002 w2011 w2034 w2039 w2059 w2077 w2086 w2092 w2100 w2106 w2117 w2124 w2131 w2136 w2191 w2286 w2389 w2399 w2431] -> w1542
          tunnel: w1541 -> [_ w1572 _ _ w1649 _ w1717 w1744 w1756 _ _ w1812 w1877 w1942 w1968 _ _ w2008 _ _ _ w2067 w2071 w2085 w2094 _ _ w2115 _ _ _ _ w2226 _ w2390 w2406]
          frame "TimeOut", Default {
            n743 = property on="Action" class="Str"("Value"="TimeOut" ("Action")) -> ()  [unwired: 2 in, 2 out]
          }
          frame "Wait" {
            n744 = flat-sequence {
              tunnel: [w1590] -> w1573
              tunnel: w1572 -> [w1590]
              tunnel: [w1589] -> w1570
              frame #0 {
                n745 = Tick Count (ms)() -> (millisecond timer value=w1589:u32)
              }
            }
            n746 = Unbundle By Name(w1573) -> ("Numeric 1"=w1564:dbl)
            n747 = property on="SS:PeriodicTime" class="DigNum (strict)"() -> ("Value"=w1566:dbl[unit])  [unwired: 2 in, 2 out]
            n748 = Multiply(x=w1564, y=1000.0) -> (x*y=w1568:dbl)
            n749 = node(w1564) -> (w1565:dbl[unit])
            n750 = property on="SS_StepsLeft" class="DigNum (strict)"() -> ("Value"=w1563:dbl)  [unwired: 2 in, 2 out]
            n751 = Round Toward -Infinity(1:w1564) -> (0:w1567:dbl)
            n752 = Subtract(x=w1566, y=w1565) -> (x-y=w1560:dbl[unit])
            n753 = Decrement(x=w1563) -> (x-1=w1562:dbl)
            n754 = Multiply(x=w1562, y=w1566) -> (x*y=w1561:dbl[unit])
            n755 = Add(x=w1561, y=w1560) -> (x+y=w1559:dbl[unit])
            n756 = for {
              N: w1567 -> [_]
              tunnel: 1000.0 ("y") -> [w1591]
              tunnel: [w1599] -> w1571
              tunnel: w1559 -> [w1596]
              i -> [w1594]
              stop <- w1599 stop-if-true
              n757 = Increment(x=w1594) -> (x+1=w1592:i32)
              n758 = Multiply(x=w1591, y=w1592) -> (x*y=w1593:dbl)
              n759 = node(w1593) -> (w1595:dbl[unit])
              n760 = property on="Stop Button" class="Bool (strict)"() -> ("Value"=w1599:bool)  [unwired: 2 in, 2 out]
              n761 = Wait (ms)(milliseconds to wait=w1591) -> (millisecond timer value=w1597:u32)
              n762 = Subtract(x=w1596, y=w1595) -> (x-y=w1598:dbl[unit])
              n763 = flat-sequence {
                tunnel: w1598 -> [w1600]
                tunnel: w1597 -> [_]
                frame #0 {
                  n764 = property on="SS_TimePrediction" class="DigNum (strict)"("Value"=w1600) -> ()  [unwired: 2 in, 2 out]
                }
              }
            }
            n765 = property on="Action" class="Str"("Value"="Wait" ("Action")) -> ()  [unwired: 2 in, 2 out]
            n766 = case shown="False" w1571 {
              tunnel: w1570 -> [w1585 _]
              tunnel: w1568 -> [w1580 _]
              frame False {
                n767 = flat-sequence {
                  tunnel: [w1588] -> w1586
                  frame #0 {
                    n768 = Tick Count (ms)() -> (millisecond timer value=w1588:u32)
                  }
                }
                n769 = Subtract(x=w1586, y=w1585) -> (x-y=w1584:u32)
                n770 = To Double Precision Float(number=w1584) -> (double precision float=w1581:dbl)
                n771 = Subtract(x=w1580, y=w1581) -> (x-y=w1582:dbl)
                n772 = Greater Than 0?(x=w1582) -> (x > 0?=w1583:bool)
                n773 = case shown="True" w1583 {
                  tunnel: w1582 -> [_ w1587]
                  frame False {
                  }
                  frame True {
                    n774 = Wait (ms)(milliseconds to wait=w1587) -> ()  [unwired: 1 out]
                  }
                }
              }
              frame True {
                # "If Aborted, do nothing"
              }
            }
          }
          frame "Close_Program" {
            w1621 = T11 {"QueueAction"=enum."TimeOut", "Numeric 1"=0.0, "Numeric 2"=0.0, "Boolean 1"=FALSE, "Boolean 2"=FALSE, "Spin Program"=[], "Spin Prg v07"=[], "Time Stamp"=timestamp(0 s since 1904-01-01), "TabControl"=enum."Measure"}  # Device Queue
            n775 = Bundle By Name(cluster=w1621, "QueueAction"=DeviceQueue_Action."Spectrometer_Close") -> (w1616:T11)
            n776 = Bundle By Name(cluster=w1616, "QueueAction"=DeviceQueue_Action."Laser_Close") -> (w1614:T11)
            n777 = Bundle By Name(cluster=w1614, "QueueAction"=DeviceQueue_Action."Arduino_Close") -> (w1608:T11)
            n778 = Enqueue Element(queue=w1620, element=w1616, error in (no error)=w1604) -> (queue out=w1618:refnum<queue>, error out=w1613:errorcluster)  [unwired: 1 in, 1 out]
            n779 = Bundle By Name(cluster=w1608, "QueueAction"=DeviceQueue_Action."Close_Program") -> (w1606:T11)
            n780 = Enqueue Element(queue=w1618, element=w1614, error in (no error)=w1613) -> (queue out=w1612:refnum<queue>, error out=w1611:errorcluster)  [unwired: 1 in, 1 out]
            n781 = Enqueue Element(queue=w1612, element=w1608, error in (no error)=w1611) -> (queue out=w1610:refnum<queue>, error out=w1609:errorcluster)  [unwired: 1 in, 1 out]
            n782 = Enqueue Element(queue=w1610, element=w1606, error in (no error)=w1609) -> (queue out=w1605:refnum<queue>, error out=w1603:errorcluster)  [unwired: 1 in, 1 out]
            n783 = First Call?() -> (First Call?: T/F=w1623:bool)
            n784 = Not(x=w1623) -> (.not. x?=w1622:bool)
          }
          frame "Abort" {
            w1645 = T11 {"QueueAction"=enum."TimeOut", "Numeric 1"=0.0, "Numeric 2"=0.0, "Boolean 1"=FALSE, "Boolean 2"=FALSE, "Spin Program"=[], "Spin Prg v07"=[], "Time Stamp"=timestamp(0 s since 1904-01-01), "TabControl"=enum."Measure"}  # Device Queue
            n785 = Flush Queue(queue=w1643, error in (no error)=w1642) -> (queue out=w1641:refnum<queue>, error out=w1640:errorcluster)  [unwired: 1 out]
            n786 = Bundle By Name(cluster=w1645, "QueueAction"=DeviceQueue_Action."Spectrometer_StopMeasurement") -> (w1637:T11)
            n787 = Bundle By Name(cluster=w1637, "QueueAction"=DeviceQueue_Action."Arduino_StopSpin") -> (w1633:T11)
            n788 = Enqueue Element(queue=w1641, element=w1637, error in (no error)=w1640) -> (queue out=w1639:refnum<queue>, error out=w1638:errorcluster)  [unwired: 1 in, 1 out]
            n789 = Bundle By Name(cluster=w1633, "QueueAction"=DeviceQueue_Action."Measure_Stop") -> (w1628:T11)
            n790 = Enqueue Element(queue=w1639, element=w1633, error in (no error)=w1638) -> (queue out=w1635:refnum<queue>, error out=w1634:errorcluster)  [unwired: 1 in, 1 out]
            n791 = Bundle By Name(cluster=w1628, "QueueAction"=DeviceQueue_Action."Spectrometer_SetTriggerMode", "Numeric 1"=0.0) -> (w1625:T11)
            n792 = Enqueue Element(queue=w1635, element=w1628, error in (no error)=w1634) -> (queue out=w1631:refnum<queue>, error out=w1629:errorcluster)  [unwired: 1 in, 1 out]
            n793 = Enqueue Element(queue=w1631, element=w1625, error in (no error)=w1629) -> (queue out=w1630:refnum<queue>, error out=w1624:errorcluster)  [unwired: 1 in, 1 out]
          }
          frame "Spectrometer_Init" {
            n794 = call-dynamic "Init.vi"("error in (no error)"=w1665, "Variant"=0, "Avantes in"=refnum<class "Avantes.lvclass"> refnum ("Avantes.lvclass")) -> ("error out"=w1664:errorcluster, "Avantes out"=w1663:refnum<class "Avantes.lvclass">)  [unwired: 7 in]
            n795 = call-dynamic "IsInit.vi"("error in (no error)"=w1664, "Avantes in"=w1663) -> ("error out"=w1660:errorcluster, "Is Init?"=w1659:bool, "Avantes out"=w1661:refnum<class "Avantes.lvclass">)  [unwired: 7 in]
            n796 = Unbundle By Name(w1649) -> ("TabControl"=w1648:T10)
            n797 = property on="Spectromter" class="Bool (strict)"("Value"=w1659) -> ()  [unwired: 2 in, 2 out]
            n798 = property on="Init_Spectrometer" class="Bool (strict)"("Value"=w1659) -> ()  [unwired: 2 in, 2 out]
            n799 = call-dynamic "Set_ExposurePerFrame.vi"("error in (no error)"=w1660, "Exposure per Frame"=1, "Avantes in"=w1661) -> ("error out"=w1655:errorcluster, "Avantes out"=w1658:refnum<class "Avantes.lvclass">)  [unwired: 7 in]
            n800 = case shown="True" w1659 {
              tunnel: w1658 -> [_ w1688]
              tunnel: w1655 -> [w1671 w1686]
              tunnel: [refnum<class "Abstract_CCD.lvclass"> refnum ("Abstract_CCD.lvclass") w1687] -> w1657
              tunnel: w1654 -> [w1669 w1698]
              tunnel: [w1671 w1691] -> w1653
              tunnel: w1652 -> [w1670 w1683]
              tunnel: [w1670 w1681] -> w1651
              tunnel: [w1669 w1679] -> w1650
              tunnel: w1649 -> [_ w1676]
              tunnel: w1648 -> [_ w1675]
              frame False {
              }
              frame True {
                w1689 = T8 {"QueueAction"=enum."TimeOut", "Data"=[], "Data_Raw"=[], "Data_Dark"=[], "Data_Ref"=[], "Device Information"=[], "Numeric Control"=0.0, "Boolean"=FALSE, "Wavelength"=[], "Time"=[], "Time Stamp"=timestamp(0 s since 1904-01-01), "Numeric Control 2"=0.0, "TabControl"=enum."Measure", "Numeric Control 3"=0.0}  # DataQueue
                n801 = case shown="\"Spectral Stability\"" w1675 {
                  tunnel: [w1700 w1702] -> w1674
                  tunnel: [w1699 w1701] -> w1673
                  frame "Measure", Default {
                    n802 = property on="Measure_IntegrationTime" class="DigNum (strict)"() -> ("Value"=w1700:dbl[unit])  [unwired: 2 in, 2 out]
                    n803 = property on="Measure_FramesSpectrometer" class="DigNum (strict)"() -> ("Value"=w1699:dbl)  [unwired: 2 in, 2 out]
                  }
                  frame "Spectral Stability" {
                    n804 = property on="SpectralStability_FramesSpectrometer" class="DigNum (strict)"() -> ("Value"=w1701:dbl)  [unwired: 2 in, 2 out]
                    n805 = property on="SpectralStability_IntegrationTime" class="DigNum (strict)"() -> ("Value"=w1702:dbl[unit])  [unwired: 2 in, 2 out]
                  }
                }
                n806 = call-dynamic "Get_WavelengthAxis.vi"("error in (no error)"=w1686, "Avantes in"=w1688) -> ("error out"=w1685:errorcluster, "lambda"=w1680:dbl[unit][], "Avantes out"=w1687:refnum<class "Avantes.lvclass">)  [unwired: 7 in]
                n807 = Unbundle(w1685) -> ("status"=w1684:bool)  [unwired: 2 out]
                n808 = property on="Error_Spectromter" class="Bool (strict)"("Value"=w1684) -> ()  [unwired: 2 in, 2 out]
                n809 = property on="Calculate Frames_Normal" class="Bool (strict)"() -> ("Value"=w1677:bool)  [unwired: 2 in, 2 out]
                n810 = Bundle By Name(cluster=w1689, "QueueAction"=DataQueue_Action."Set_Wavelength", "Wavelength"=w1680) -> (w1690:T8)
                n811 = node(w1674) -> (w1696:dbl)
                n812 = Bundle By Name(cluster=w1676, "QueueAction"=DeviceQueue_Action."Spectrometer_SetIntegrationTime", "Numeric 1"=w1696, "Boolean 1"=w1677) -> (w1694:T11)
                n813 = Enqueue Element(queue=w1683, element=w1690) -> (queue out=w1681:refnum<queue>)  [unwired: 2 in, 2 out]
                n814 = Bundle By Name(cluster=w1694, "QueueAction"=DeviceQueue_Action."Spectrometer_SetFrames", "Numeric 1"=w1673) -> (w1693:T11)
                n815 = Enqueue Element(queue=w1698, element=w1694, error in (no error)=w1686) -> (queue out=w1695:refnum<queue>, error out=w1692:errorcluster)  [unwired: 1 in, 1 out]
                n816 = Enqueue Element(queue=w1695, element=w1693, error in (no error)=w1692) -> (queue out=w1679:refnum<queue>, error out=w1691:errorcluster)  [unwired: 1 in, 1 out]
              }
            }
            n817 = Bundle By Name(cluster=w1662, "Abstract_CCD.lvclass"=w1657) -> (w1656:T6)
          }
          frame "Spectrometer_Close" {
            n818 = property on="Spectromter" class="Bool (strict)"("Value"=FALSE ("Spectromter")) -> ()  [unwired: 2 in, 2 out]
            n819 = Unbundle By Name(w1708) -> ("Abstract_CCD.lvclass"=w1711:refnum<class "Abstract_CCD.lvclass">)
            n820 = flat-sequence {
              tunnel: [refnum<class "Abstract_CCD.lvclass"> refnum ("Abstract_CCD.lvclass")] -> w1705
              tunnel: w1704 -> [_]
              frame #0 {
              }
            }
            n821 = call-dynamic "Close.vi"("error in (no error)"=w1710, "Abstract_CCD in"=w1711) -> ("error out"=w1704:errorcluster)  [unwired: 8 in, 1 out]
            n822 = Bundle By Name(cluster=w1708, "Abstract_CCD.lvclass"=w1705) -> (w1707:T6)
          }
          frame "Spectrometer_Measure" {
            w1730 = T8 {"QueueAction"=enum."TimeOut", "Data"=[], "Data_Raw"=[], "Data_Dark"=[], "Data_Ref"=[], "Device Information"=[], "Numeric Control"=0.0, "Boolean"=FALSE, "Wavelength"=[], "Time"=[], "Time Stamp"=timestamp(0 s since 1904-01-01), "Numeric Control 2"=0.0, "TabControl"=enum."Measure", "Numeric Control 3"=0.0}  # DataQueue
            n823 = Unbundle By Name(w1725) -> ("Abstract_CCD.lvclass"=w1729:refnum<class "Abstract_CCD.lvclass">)
            n824 = Unbundle By Name(w1717) -> ("Time Stamp"=w1714:timestamp, "TabControl"=w1715:T10)
            n825 = Get Date/Time In Seconds() -> (seconds since 1Jan1904=w1713:timestamp)
            n826 = Subtract(x=w1713, y=w1714) -> (x-y=w1716:dbl)
            n827 = call-dynamic "Measure.vi"("error in (no error)"=w1727, "Abstract_CCD in"=w1729) -> ("error out"=w1726:errorcluster, "Data Raw"=w1722:T14, "Data"=w1723:T14, "Darkspec"=w1721:T14, "Time"=w1720:dbl[])  [unwired: 3 in, 2 out]
            n828 = Bundle By Name(cluster=w1730, "QueueAction"=DataQueue_Action."Spectrometer_Measure", "Data"=w1723, "Data_Raw"=w1722, "Data_Dark"=w1721, "Time"=w1720, "Time Stamp"=w1714, "Numeric Control 2"=w1716, "TabControl"=w1715) -> (w1731:T8)
            n829 = Enqueue Element(queue=w1718, element=w1731) -> (queue out=w1719:refnum<queue>)  [unwired: 2 in, 2 out]
          }
          frame "Spectrometer_MeasureAdvanced" {
            w1741 = T8 {"QueueAction"=enum."TimeOut", "Data"=[], "Data_Raw"=[], "Data_Dark"=[], "Data_Ref"=[], "Device Information"=[], "Numeric Control"=0.0, "Boolean"=FALSE, "Wavelength"=[], "Time"=[], "Time Stamp"=timestamp(0 s since 1904-01-01), "Numeric Control 2"=0.0, "TabControl"=enum."Measure", "Numeric Control 3"=0.0}  # DataQueue
            w1755 = T8 {"QueueAction"=enum."TimeOut", "Data"=[], "Data_Raw"=[], "Data_Dark"=[], "Data_Ref"=[], "Device Information"=[], "Numeric Control"=0.0, "Boolean"=FALSE, "Wavelength"=[], "Time"=[], "Time Stamp"=timestamp(0 s since 1904-01-01), "Numeric Control 2"=0.0, "TabControl"=enum."Measure", "Numeric Control 3"=0.0}  # DataQueue
            n830 = Unbundle By Name(w1750) -> ("Abstract_CCD.lvclass"=w1754:refnum<class "Abstract_CCD.lvclass">)
            n831 = Unbundle By Name(w1744) -> ("Time Stamp"=w1743:timestamp)
            n832 = call-dynamic "Measure.vi"("error in (no error)"=w1752, "Abstract_CCD in"=w1754) -> ("error out"=w1751:errorcluster, "Data Raw"=w1747:T14, "Data"=w1748:T14, "Darkspec"=w1746:T14, "Time"=w1745:dbl[])  [unwired: 3 in, 2 out]
            n833 = Bundle By Name(cluster=w1741, "QueueAction"=DataQueue_Action."Measure_SpectrumAdvanced") -> (w1739:T8)
            n834 = Bundle By Name(cluster=w1755, "QueueAction"=DataQueue_Action."Spectrometer_Measure", "Data"=w1748, "Data_Raw"=w1747, "Data_Dark"=w1746, "Time"=w1745, "Time Stamp"=w1743) -> (w1736:T8)
            n835 = Enqueue Element(queue=w1742, element=w1739) -> (queue out=w1738:refnum<queue>)  [unwired: 2 in, 2 out]
            n836 = Enqueue Element(queue=w1738, element=w1736) -> (queue out=w1737:refnum<queue>)  [unwired: 2 in, 2 out]
            n837 = Bundle By Name(cluster=w1736, "QueueAction"=DataQueue_Action."Stop_Measurement") -> (w1734:T8)
            n838 = property on="Action" class="Str"("Value"="Measure Spectra A" ("Action")) -> ()  [unwired: 2 in, 2 out]
            n839 = Enqueue Element(queue=w1737, element=w1734) -> (queue out=w1733:refnum<queue>)  [unwired: 2 in, 2 out]
          }
          frame "Spectrometer_Preview" {
            w1771 = T8 {"QueueAction"=enum."TimeOut", "Data"=[], "Data_Raw"=[], "Data_Dark"=[], "Data_Ref"=[], "Device Information"=[], "Numeric Control"=0.0, "Boolean"=FALSE, "Wavelength"=[], "Time"=[], "Time Stamp"=timestamp(0 s since 1904-01-01), "Numeric Control 2"=0.0, "TabControl"=enum."Measure", "Numeric Control 3"=0.0}  # DataQueue
            n840 = Unbundle By Name(w1763) -> ("Abstract_CCD.lvclass"=w1761:refnum<class "Abstract_CCD.lvclass">)
            n841 = Unbundle By Name(w1756) -> ("TabControl"=w1757:T10)
            n842 = call-dynamic "Measure.vi"("error in (no error)"=w1760, "Abstract_CCD in"=w1761) -> ("error out"=w1758:errorcluster, "Data Raw"=w1768:T14, "Abstract_CCD out"=w1759:refnum<class "Abstract_CCD.lvclass">)  [unwired: 3 in, 4 out]
            n843 = case shown="\"Measure\"" w1757 {
              tunnel: [FALSE ("Value") w1775 w1776] -> w1766
              tunnel: w1758 -> [_ w1774 _]
              frame Default {
              }
              frame "Measure" {
                n844 = property on="Measure_Preview" class="Bool (strict)"(error in=w1774) -> ("Value"=w1775:bool)  [unwired: 1 in, 2 out]
              }
              frame "Spectral Stability" {
                n845 = property on="SpectralStability_Preview" class="Bool (strict)"() -> ("Value"=w1776:bool)  [unwired: 2 in, 2 out]
              }
            }
            n846 = case shown="True" w1766 {
              tunnel: [w1777 w1780] -> w1765
              tunnel: w1764 -> [w1777 w1779]
              tunnel: w1756 -> [_ w1778]
              frame False {
              }
              frame True {
                n847 = Bundle By Name(cluster=w1778, "QueueAction"=DeviceQueue_Action."Spectrometer_Preview") -> (w1781:T11)
                n848 = Enqueue Element(queue=w1779, element=w1781) -> (queue out=w1780:refnum<queue>)  [unwired: 2 in, 2 out]
              }
            }
            n849 = Bundle By Name(cluster=w1771, "Data_Raw"=w1768, "QueueAction"=DataQueue_Action."Spectrometer_Preview", "TabControl"=w1757) -> (w1772:T8)
            n850 = Enqueue Element(queue=w1770, element=w1772) -> (queue out=w1769:refnum<queue>)  [unwired: 2 in, 2 out]
            n851 = Bundle By Name(cluster=w1763, "Abstract_CCD.lvclass"=w1759) -> (w1762:T6)
          }
          frame "Spectrometer_StartMeasurement" {
            n852 = Unbundle By Name(w1785) -> ("Abstract_CCD.lvclass"=w1789:refnum<class "Abstract_CCD.lvclass">)
            n853 = call-dynamic "StartMeasure.vi"("error in (no error)"=w1790, "Frames"=-1, "Abstract_CCD in"=w1789) -> ("error out"=w1788:errorcluster, "Abstract_CCD out"=w1784:refnum<class "Abstract_CCD.lvclass">)  [unwired: 7 in]
            n854 = Bundle By Name(cluster=w1785, "Abstract_CCD.lvclass"=w1784) -> (w1783:T6)
          }
          frame "Spectrometer_StopMeasurement" {
            n855 = Unbundle By Name(w1797) -> ("Abstract_CCD.lvclass"=w1799:refnum<class "Abstract_CCD.lvclass">)
            n856 = call-dynamic "StopMeasurement.vi"("error in (no error)"=w1798, "Abstract_CCD in"=w1799) -> ("error out"=w1795:errorcluster, "Abstract_CCD out"=w1796:refnum<class "Abstract_CCD.lvclass">)  [unwired: 8 in]
            n857 = Bundle By Name(cluster=w1797, "Abstract_CCD.lvclass"=w1796) -> (w1792:T6)
          }
          frame "Spectrometer_GetData" {
            w1809 = T8 {"QueueAction"=enum."TimeOut", "Data"=[], "Data_Raw"=[], "Data_Dark"=[], "Data_Ref"=[], "Device Information"=[], "Numeric Control"=0.0, "Boolean"=FALSE, "Wavelength"=[], "Time"=[], "Time Stamp"=timestamp(0 s since 1904-01-01), "Numeric Control 2"=0.0, "TabControl"=enum."Measure", "Numeric Control 3"=0.0}  # DataQueue
            n858 = Unbundle By Name(w1806) -> ("Abstract_CCD.lvclass"=w1811:refnum<class "Abstract_CCD.lvclass">)
            n859 = Unbundle By Name(w1812) -> ("Numeric 1"=w1803:dbl)
            n860 = call-dynamic "Measure_GetData.vi"("error in (no error)"=w1810, "SpectraCount"=w1803, "Abstract_CCD in"=w1811) -> ("error out"=w1801:errorcluster, "Data_Raw"=w1800:T14, "Time"=w1802:dbl[])  [unwired: 5 in, 1 out]
            n861 = Bundle By Name(cluster=w1809, "QueueAction"=DataQueue_Action."Spectrometer_Measure", "Data_Raw"=w1800, "Time"=w1802) -> (w1808:T8)
            n862 = Enqueue Element(queue=w1805, element=w1808) -> (queue out=w1804:refnum<queue>)  [unwired: 2 in, 2 out]
          }
          frame "Spectrometer_GetData_Short" {
            w1860 = 0 ("index (page)")
            w1855 = nan
            w1876 = T8 {"QueueAction"=enum."TimeOut", "Data"=[], "Data_Raw"=[], "Data_Dark"=[], "Data_Ref"=[], "Device Information"=[], "Numeric Control"=0.0, "Boolean"=FALSE, "Wavelength"=[], "Time"=[], "Time Stamp"=timestamp(0 s since 1904-01-01), "Numeric Control 2"=0.0, "TabControl"=enum."Measure", "Numeric Control 3"=0.0}  # DataQueue
            # "Frames"
            # "Start Time + Offset"
            n863 = Unbundle By Name(w1857) -> ("Abstract_CCD.lvclass"=w1865:refnum<class "Abstract_CCD.lvclass">)
            n864 = local read "Seconds to Spin_Short"() -> (w1840:dbl[unit])
            n865 = Unbundle By Name(w1877) -> ("Numeric 2"=w1831:dbl)
            n866 = call <vilib>:"High Resolution Relative Seconds.vi"() -> ("relative seconds"=w1871:dbl)
            n867 = node("Time Detect") -> (w1870:dbl)
            n868 = To Long Integer(number=w1831) -> (32bit integer=w1826:i32)
            n869 = node(w1840) -> (w1869:dbl)
            n870 = call-dynamic "Measure_GetData_SpectraOutput.vi"("error in (no error)"=w1866, "Abstract_CCD in"=w1865) -> ("error out"=w1868:errorcluster, "Spectra"=w1861:dbl[], "Abstract_CCD out"=w1867:refnum<class "Abstract_CCD.lvclass">, "Time"=w1852:dbl)  [unwired: 6 in]
            n871 = Compound Arithmetic op=ADD(w1871, w1869, w1870) -> (w1858:dbl)
            n872 = Initialize Array(w1855, w1826) -> (w1854:dbl[])
            n873 = Array Size(array=w1861) -> (size(s)=w1864:i32)
            n874 = Initialize Array(w1855, w1826, 1 ("index"), w1864) -> (w1862:dbl[][][])
            n875 = Replace Array Subset(array=w1854, new element=w1852, index=0) -> (w1851:dbl[])
            n876 = Replace Array Subset(array=w1862, new element=w1861, index (dim 0)=w1860, index (dim 1)=w1860) -> (w1859:dbl[][][])  [unwired: 1 in]
            n877 = while {
              shift-right: [w1931] -> w1836
              shift-left: w1868 -> [w1932]
              shift-right: [w1928] -> w1837
              shift-left: w1859 -> [w1930]
              tunnel: w1858 -> [w1927]
              shift-right: [w1924] -> w1838
              shift-left: w1851 -> [w1926]
              tunnel: [w1921] -> w1839
              tunnel: [w1919] -> w1834
              shift-right: [w1918] -> w1835
              shift-left: w1867 -> [w1933]
              i -> [w1920]
              stop <- w1922 stop-if-true
              # "Wait for correct Time"
              n878 = call <vilib>:"High Resolution Relative Seconds.vi"() -> ("relative seconds"=w1923:dbl)
              n879 = call-dynamic "Measure_GetData_SpectraOutput.vi"("error in (no error)"=w1932, "Abstract_CCD in"=w1933) -> ("error out"=w1931:errorcluster, "Spectra"=w1921:dbl[], "Abstract_CCD out"=w1918:refnum<class "Abstract_CCD.lvclass">, "Time"=w1925:dbl)  [unwired: 6 in]
              n880 = Greater?(x=w1923, y=w1927) -> (0:w1922:bool)
              n881 = Increment(x=w1920) -> (x+1=w1919:i32)
              n882 = Replace Array Subset(array=w1926, new element=w1925, index=w1919) -> (w1924:dbl[])
              n883 = Replace Array Subset(array=w1930, new element=w1921, index (dim 0)=w1919, index (dim 1)=0 ("disabled index (row)")) -> (w1928:dbl[][][])  [unwired: 1 in]
            }
            n884 = local read "WL-Det\nPos"() -> (w1833:i32)
            n885 = Increment(x=w1834) -> (x+1=w1819:i32)
            n886 = Index Array(array=w1839, index=w1833) -> (element=w1832:dbl)
            n887 = while {
              shift-right: [w1911] -> w1828
              shift-left: w1838 -> [w1913]
              shift-right: [w1909] -> w1829
              shift-left: w1837 -> [w1910]
              shift-right: [w1901] -> w1818
              shift-left: w1836 -> [w1917]
              tunnel: w1819 -> [w1915]
              tunnel: w1833 -> [w1903]
              tunnel: w1826 -> [w1900]
              tunnel: [w1895] -> w1824
              tunnel: [w1894] -> w1815
              shift-right: [w1896] -> w1827
              shift-left: w1835 -> [w1916]
              i -> [w1914]
              stop <- w1897 stop-if-true
              # "Wait for threshold"
              n888 = call-dynamic "Measure_GetData_SpectraOutput.vi"("error in (no error)"=w1917, "Abstract_CCD in"=w1916) -> ("error out"=w1901:errorcluster, "Spectra"=w1904:dbl[], "Abstract_CCD out"=w1896:refnum<class "Abstract_CCD.lvclass">, "Time"=w1912:dbl)  [unwired: 6 in]
              n889 = Add(x=w1915, y=w1914) -> (x+y=w1895:i32)
              n890 = Index Array(array=w1904, index=w1903) -> (element=w1905:dbl)
              n891 = Replace Array Subset(array=w1913, new element=w1912, index=w1895) -> (w1911:dbl[])
              n892 = Replace Array Subset(array=w1910, new element=w1904, index (dim 0)=w1895, index (dim 1)=0 ("disabled index (row)")) -> (w1909:dbl[][][])  [unwired: 1 in]
              n893 = Divide(x=w1905, y="Reference\nValue") -> (x/y=w1906:dbl)
              n894 = Less?(x=w1906, y="Threshold") -> (x < y?=w1899:bool)
              n895 = Equal?(x=w1900, y=w1895) -> (x = y?=w1898:bool)
              n896 = call <vilib>:"High Resolution Relative Seconds.vi"() -> ("relative seconds"=w1894:dbl)
              n897 = Or(x=w1898, y=w1899) -> (x .or. y?=w1897:bool)
            }
            n898 = local write "Reference\nValue"(w1832) -> ()
            n899 = Unbundle By Name(w1857) -> ("SpinCoater.lvclass"=w1830:refnum<class "SpinCoater.lvclass">)
            n900 = Subtract(x=w1826, y=w1824) -> (x-y=w1825:i32)
            n901 = Increment(x=w1824) -> (x+1=w1822:i32)
            n902 = call-dynamic "Stop_Short.vi"("error in (no error)"=w1818, "SpinCoater in"=w1830) -> ("error out"=w1817:errorcluster)  [unwired: 8 in, 1 out]
            n903 = for {
              N: w1825 -> [_]
              shift-right: [w1889] -> w1823
              shift-left: w1828 -> [w1888]
              shift-right: [w1885] -> w1821
              shift-left: w1829 -> [w1886]
              tunnel: w1822 -> [w1891]
              shift-right: [w1881] -> w1820
              shift-left: w1818 -> [w1893]
              shift-right: [w1880] -> _
              shift-left: w1827 -> [w1892]
              i -> [w1890]
              n904 = call-dynamic "Measure_GetData_SpectraOutput.vi"("error in (no error)"=w1893, "Abstract_CCD in"=w1892) -> ("error out"=w1881:errorcluster, "Spectra"=w1882:dbl[], "Abstract_CCD out"=w1880:refnum<class "Abstract_CCD.lvclass">, "Time"=w1887:dbl)  [unwired: 6 in]
              n905 = Add(x=w1890, y=w1891) -> (x+y=w1884:i32)
              n906 = Replace Array Subset(array=w1888, new element=w1887, index=w1884) -> (w1889:dbl[])
              n907 = Replace Array Subset(array=w1886, new element=w1882, index (dim 0)=w1884, index (dim 1)=0 ("disabled index (row)")) -> (w1885:dbl[][][])  [unwired: 1 in]
            }
            n908 = flat-sequence {
              tunnel: w1817 -> [_]
              tunnel: [w1879] -> w1816
              frame #0 {
                n909 = call <vilib>:"High Resolution Relative Seconds.vi"() -> ("relative seconds"=w1879:dbl)
              }
            }
            n910 = Subtract(x=w1815, y=w1816) -> (x-y=→"x-y":dbl)
            n911 = Array Size(array=w1821) -> (size(s)=w1849:i32[])
            n912 = Index Array(array=w1849, index #1=0 ("index"), index #2=1 ("index"), index #3=2 ("index")) -> (element #1=w1846:i32, element #2=w1847:i32, element #3=w1848:i32)
            n913 = Bundle By Name(cluster=T15 {"Image"=[], "Frame Size"={"F"=0, "Y"=0, "X"=0}} ("Cluster"), "Image"=w1821, "Frame Size.F"=w1846, "Frame Size.Y"=w1847, "Frame Size.X"=w1848) -> (w1842:T15)
            n914 = Build Array(w1842) -> (w1841:T14)
            n915 = Bundle By Name(cluster=w1876, "QueueAction"=DataQueue_Action."Spectrometer_Measure", "Data_Raw"=w1841, "Time"=w1823) -> (w1875:T8)
            n916 = Enqueue Element(queue=w1873, element=w1875) -> (queue out=w1872:refnum<queue>)  [unwired: 2 in, 2 out]
          }
          frame "Spectrometer_SetIntegrationTime" {
            n917 = Unbundle By Name(w1942) -> ("Numeric 1"=w1944:dbl)
            n918 = Unbundle By Name(w1938) -> ("Abstract_CCD.lvclass"=w1946:refnum<class "Abstract_CCD.lvclass">)
            n919 = Unbundle By Name(w1942) -> ("TabControl"=w1934:T10, "Boolean 1"=w1941:bool)
            n920 = node(w1944) -> (w1943:dbl[unit])
            n921 = call-dynamic "Set_ExposureTime.vi"("error in (no error)"=w1945, "Exposure Time"=w1943, "Abstract_CCD in"=w1946) -> ("error out"=w1949:errorcluster, "Abstract_CCD out"=w1948:refnum<class "Abstract_CCD.lvclass">)  [unwired: 7 in]
            n922 = call-dynamic "Get_FrameRate.vi"("error in (no error)"=w1949, "Abstract_CCD in"=w1948) -> ("error out"=w1939:errorcluster, "Frame Rate"=w1940:dbl[unit], "Abstract_CCD out"=w1937:refnum<class "Abstract_CCD.lvclass">)  [unwired: 7 in]
            n923 = Bundle By Name(cluster=w1938, "Abstract_CCD.lvclass"=w1937) -> (w1936:T6)
            n924 = case shown="\"Measure\"" w1934 {
              tunnel: w1941 -> [_ _ w1952]
              tunnel: w1940 -> [_ w1950 w1951]
              frame Default {
              }
              frame "Spectral Stability" {
                "SpectralStability_FrameRate" <- w1950
              }
              frame "Measure" {
                n925 = case shown="True" w1952 {
                  tunnel: w1951 -> [_ w1956]
                  frame False {
                  }
                  frame True {
                    n926 = property on="Program Spin Coater" class="Arr (strict)"() -> ("Value"=w1953:T2)  [unwired: 2 in, 2 out]
                    n927 = property on="Seconds to Spin_Normal" class="DigNum (strict)"() -> ("Value"=w1958:dbl[unit])  [unwired: 2 in, 2 out]
                    n928 = property on="Seconds after Spin" class="DigNum (strict)"() -> ("Value"=w1957:dbl[unit])  [unwired: 2 in, 2 out]
                    n929 = call "CalculateFrames_v03.vi"("Program Spin Coater"=w1953, "Seconds End"=w1957, "Seconds Start"=w1958, "Frame Rate"=w1956) -> ("Time"=w1955:dbl, "Frames"=w1954:i32)  [unwired: 6 in]
                    n930 = property on="Frames" class="DigNum (strict)"("Value"=w1954) -> ()  [unwired: 2 in, 2 out]
                    n931 = property on="Overall Time" class="DigNum (strict)"("Value"=w1955) -> ()  [unwired: 2 in, 2 out]
                  }
                }
                "Measure_FrameRate" <- w1951
              }
            }
          }
          frame "Spectrometer_SetFrames" {
            n932 = Unbundle By Name(w1960) -> ("Abstract_CCD.lvclass"=w1965:refnum<class "Abstract_CCD.lvclass">)
            n933 = Unbundle By Name(w1968) -> ("Numeric 1"=w1962:dbl)
            n934 = call-dynamic "Set_Frames.vi"("error in (no error)"=w1964, "Frames"=w1962, "Abstract_CCD in"=w1965) -> ("error out"=w1963:errorcluster, "Abstract_CCD out"=w1959:refnum<class "Abstract_CCD.lvclass">)  [unwired: 7 in]
            n935 = Bundle By Name(cluster=w1960, "Abstract_CCD.lvclass"=w1959) -> (w1961:T6)
          }
          frame "Spectrometer_SetDarkspec" {
            w1983 = T8 {"QueueAction"=enum."TimeOut", "Data"=[], "Data_Raw"=[], "Data_Dark"=[], "Data_Ref"=[], "Device Information"=[], "Numeric Control"=0.0, "Boolean"=FALSE, "Wavelength"=[], "Time"=[], "Time Stamp"=timestamp(0 s since 1904-01-01), "Numeric Control 2"=0.0, "TabControl"=enum."Measure", "Numeric Control 3"=0.0}  # DataQueue
            n936 = Unbundle By Name(w1978) -> ("Abstract_CCD.lvclass"=w1976:refnum<class "Abstract_CCD.lvclass">)
            n937 = call-dynamic "Measure.vi"("error in (no error)"=w1975, "Abstract_CCD in"=w1976) -> ("error out"=w1973:errorcluster, "Data Raw"=w1980:T14, "Abstract_CCD out"=w1974:refnum<class "Abstract_CCD.lvclass">)  [unwired: 3 in, 4 out]
            n938 = Bundle By Name(cluster=w1983, "QueueAction"=DataQueue_Action."Set_Dark", "Data_Dark"=w1980) -> (w1984:T8)
            n939 = Enqueue Element(queue=w1982, element=w1984) -> (queue out=w1979:refnum<queue>)  [unwired: 2 in, 2 out]
            n940 = Bundle By Name(cluster=w1978, "Abstract_CCD.lvclass"=w1974) -> (w1977:T6)
            n941 = property on="Measure:\nRecord_Darkspec" class="Bool (strict)"(error in=w1973, "Value"=FALSE ("Record_Darkspec")) -> (error out=w1971:errorcluster)  [unwired: 1 in, 1 out]
            n942 = property on="SpectralStability:\nRecord_Darkspec" class="Bool (strict)"(error in=w1971, "Value"=FALSE ("SpectralStability:\nRecord_Darkspec")) -> (error out=w1970:errorcluster)  [unwired: 1 in, 1 out]
          }
          frame "Spectrometer_SetReference" {
            w1998 = T8 {"QueueAction"=enum."TimeOut", "Data"=[], "Data_Raw"=[], "Data_Dark"=[], "Data_Ref"=[], "Device Information"=[], "Numeric Control"=0.0, "Boolean"=FALSE, "Wavelength"=[], "Time"=[], "Time Stamp"=timestamp(0 s since 1904-01-01), "Numeric Control 2"=0.0, "TabControl"=enum."Measure", "Numeric Control 3"=0.0}  # DataQueue
            n943 = Unbundle By Name(w1993) -> ("Abstract_CCD.lvclass"=w1990:refnum<class "Abstract_CCD.lvclass">)
            n944 = call-dynamic "Measure.vi"("error in (no error)"=w1991, "Abstract_CCD in"=w1990) -> ("error out"=w1988:errorcluster, "Data Raw"=w1995:T14, "Abstract_CCD out"=w1989:refnum<class "Abstract_CCD.lvclass">)  [unwired: 3 in, 4 out]
            n945 = Bundle By Name(cluster=w1998, "QueueAction"=DataQueue_Action."Set_Ref", "Data_Ref"=w1995) -> (w1999:T8)
            n946 = Enqueue Element(queue=w1997, element=w1999) -> (queue out=w1994:refnum<queue>)  [unwired: 2 in, 2 out]
            n947 = Bundle By Name(cluster=w1993, "Abstract_CCD.lvclass"=w1989) -> (w1992:T6)
            n948 = property on="Record RefSpec" class="Bool (strict)"(error in=w1988, "Value"=FALSE ("Record RefSpec")) -> (error out=w1987:errorcluster)  [unwired: 1 in, 1 out]
          }
          frame "Spectrometer_SetTriggerMode" {
            n949 = Unbundle By Name(w2004) -> ("Abstract_CCD.lvclass"=w2009:refnum<class "Abstract_CCD.lvclass">)
            n950 = Unbundle By Name(w2008) -> ("Numeric 1"=w2006:dbl)
            n951 = call-dynamic "Set_TriggerMode.vi"("error in (no error)"=w2007, "Trigger Mode"=w2006, "Abstract_CCD in"=w2009) -> ("error out"=w2005:errorcluster, "Abstract_CCD out"=w2003:refnum<class "Abstract_CCD.lvclass">)  [unwired: 7 in]
            n952 = Bundle By Name(cluster=w2004, "Abstract_CCD.lvclass"=w2003) -> (w2002:T6)
          }
          frame "Spectrometer_DeviceInformation" {
            w2017 = T8 {"QueueAction"=enum."TimeOut", "Data"=[], "Data_Raw"=[], "Data_Dark"=[], "Data_Ref"=[], "Device Information"=[], "Numeric Control"=0.0, "Boolean"=FALSE, "Wavelength"=[], "Time"=[], "Time Stamp"=timestamp(0 s since 1904-01-01), "Numeric Control 2"=0.0, "TabControl"=enum."Measure", "Numeric Control 3"=0.0}  # DataQueue
            n953 = Unbundle By Name(w2011) -> ("Abstract_CCD.lvclass"=w2019:refnum<class "Abstract_CCD.lvclass">)
            n954 = call-dynamic "Get_DeviceInformation.vi"("error in (no error)"=w2018, "Abstract_CCD in"=w2019) -> ("error out"=w2013:errorcluster, "Array"=w2020:string[])  [unwired: 7 in, 1 out]
            n955 = Bundle By Name(cluster=w2017, "QueueAction"=DataQueue_Action."Transfer_Settings", "Device Information"=w2020) -> (w2015:T8)
            n956 = Enqueue Element(queue=w2016, element=w2015, error in (no error)=w2013) -> (queue out=w2014:refnum<queue>, error out=w2012:errorcluster)  [unwired: 1 in, 1 out]
          }
          frame "Arduino_Init" {
            n957 = Unbundle By Name(w2032) -> ("SpinCoater.lvclass"=w2031:refnum<class "SpinCoater.lvclass">)
            n958 = call-dynamic "Init.vi"("error in (no error)"=w2030, "Variant"="Port Arduino", "SpinCoater in"=w2031) -> ("error out"=w2027:errorcluster, "SpinCoater out"=w2028:refnum<class "SpinCoater.lvclass">)  [unwired: 7 in]
            n959 = call-dynamic "IsInit.vi"("error in (no error)"=w2027, "SpinCoater in"=w2028) -> ("error out"=w2024:errorcluster, "Init"=w2025:bool, "SpinCoater out"=w2026:refnum<class "SpinCoater.lvclass">)  [unwired: 7 in]
            n960 = property on="Arduino" class="Bool (strict)"("Value"=w2025) -> ()  [unwired: 2 in, 2 out]
            n961 = case shown="False" w2025 {
              tunnel: [w2036 w2038] -> w2033
              tunnel: w2024 -> [w2036 w2038]
              frame False {
              }
              frame True {
                n962 = property on="Program Spin Coater" class="Arr (strict)"() -> ("Value"=w2037:T2)  [unwired: 2 in, 2 out]
                n963 = property on="Program Spin Coater" class="Arr (strict)"("Val(Sgnl)"=w2037) -> ()  [unwired: 2 in, 2 out]
              }
            }
            n964 = Bundle By Name(cluster=w2032, "SpinCoater.lvclass"=w2026) -> (w2034:T6)
          }
          frame "Arduino_Close" {
            n965 = Unbundle By Name(w2041) -> ("SpinCoater.lvclass"=w2049:refnum<class "SpinCoater.lvclass">)
            n966 = property on="Arduino" class="Bool (strict)"() -> (error out=w2043:errorcluster, "Value"=w2042:bool)  [unwired: 2 in, 1 out]
            n967 = property on="Arduino" class="Bool (strict)"(error in=w2043, "Value"=FALSE ("Arduino")) -> ()  [unwired: 1 in, 2 out]
            n968 = case shown="False" w2042 {
              tunnel: w2049 -> [w2050 w2055]
              tunnel: w2048 -> [w2051 w2054]
              tunnel: [w2051 w2053] -> w2047
              tunnel: [w2050 w2052] -> w2040
              frame False {
              }
              frame True {
                n969 = call-dynamic "Close.vi"("error in (no error)"=w2054, "SpinCoater in"=w2055) -> ("error out"=w2053:errorcluster, "SpinCoater out"=w2052:refnum<class "SpinCoater.lvclass">)  [unwired: 8 in]
              }
            }
            n970 = Bundle By Name(cluster=w2041, "SpinCoater.lvclass"=w2040) -> (w2039:T6)
          }
          frame "Arduino_LoadProgram" {
            n971 = Unbundle By Name(w2067) -> ("Spin Prg v07"=w2058:T2, "Numeric 1"=w2066:dbl, "Numeric 2"=w2057:dbl)
            n972 = Unbundle By Name(w2062) -> ("SpinCoater.lvclass"=w2065:refnum<class "SpinCoater.lvclass">)
            n973 = node(w2066) -> (w2064:dbl[unit])
            n974 = node(w2057) -> (w2056:dbl[unit])
            n975 = call-dynamic "Program_Load_v03.vi"("Time Spin"=w2056, "error in (no error)"=w2063, "Time Start"=w2064, "Program Spin Coater"=w2058, "SpinCoater in"=w2065) -> ("error out"=w2060:errorcluster, "SpinCoater out"=w2061:refnum<class "SpinCoater.lvclass">)  [unwired: 5 in]
            n976 = Bundle By Name(cluster=w2062, "SpinCoater.lvclass"=w2061) -> (w2059:T6)
          }
          frame "Arduino_StartProgram" {
            n977 = Unbundle By Name(w2077) -> ("SpinCoater.lvclass"=w2074:refnum<class "SpinCoater.lvclass">)
            n978 = Unbundle By Name(w2071) -> ("Numeric 1"=w2070:dbl)
            n979 = call-dynamic "Program_Run.vi"("error in (no error)"=w2073, "Numeric"=w2070, "SpinCoater in"=w2074) -> ("error out"=w2072:errorcluster)  [unwired: 7 in, 1 out]
            n980 = property on="Action" class="Str"("Value"="Measuring" ("Action")) -> ()  [unwired: 2 in, 2 out]
          }
          frame "Arduino_SetSpeed" {
            n981 = Unbundle By Name(w2086) -> ("SpinCoater.lvclass"=w2082:refnum<class "SpinCoater.lvclass">)
            n982 = Unbundle By Name(w2085) -> ("Numeric 1"=w2084:dbl)
            n983 = To Unsigned Long Integer(number=w2084) -> (unsigned 32bit integer=w2080:u32)
            n984 = call-dynamic "Debug_SetSpeed.vi"("error in (no error)"=w2081, "Speed"=w2080, "SpinCoater in"=w2082) -> ("error out"=w2079:errorcluster)  [unwired: 7 in, 1 out]
          }
          frame "Arduino_SetMillis" {
            n985 = Unbundle By Name(w2092) -> ("SpinCoater.lvclass"=w2091:refnum<class "SpinCoater.lvclass">)
            n986 = Unbundle By Name(w2094) -> ("Numeric 1"=w2096:dbl)
            n987 = To Unsigned Long Integer(number=w2096) -> (unsigned 32bit integer=w2088:u32)
            n988 = call-dynamic "Debug_SetMillis.vi"("error in (no error)"=w2090, "Milliseconds"=w2088, "SpinCoater in"=w2091) -> ("error out"=w2089:errorcluster)  [unwired: 7 in, 1 out]
          }
          frame "Arduino_StopSpin" {
            n989 = Unbundle By Name(w2100) -> ("SpinCoater.lvclass"=w2099:refnum<class "SpinCoater.lvclass">)
            n990 = call-dynamic "Stop_Spin.vi"("error in (no error)"=w2098, "SpinCoater in"=w2099) -> ("error out"=w2097:errorcluster)  [unwired: 8 in, 1 out]
          }
          frame "Arduino_ShortStop" {
            n991 = Unbundle By Name(w2106) -> ("SpinCoater.lvclass"=w2105:refnum<class "SpinCoater.lvclass">)
            n992 = call-dynamic "Stop_Short.vi"("error in (no error)"=w2104, "SpinCoater in"=w2105) -> ("error out"=w2103:errorcluster)  [unwired: 8 in, 1 out]
          }
          frame "Arduino_Shutter_SetPosition" {
            n993 = Unbundle By Name(w2115) -> ("Numeric 1"=w2114:dbl)
            n994 = Unbundle By Name(w2117) -> ("SpinCoater.lvclass"=w2116:refnum<class "SpinCoater.lvclass">)
            n995 = Number To Decimal String(number=w2114) -> (decimal integer string=w2113:string)  [unwired: 1 in]
            n996 = Concatenate Strings("!shu_M" ("string"), w2113) -> (w2111:string)
            n997 = call-dynamic "Send_String.vi"("error in (no error)"=w2110, "String"=w2111, "SpinCoater in"=w2116) -> ("error out"=w2109:errorcluster)  [unwired: 6 in, 2 out]
          }
          frame "Arduino_Shutter_Close" {
            n998 = Unbundle By Name(w2124) -> ("SpinCoater.lvclass"=w2123:refnum<class "SpinCoater.lvclass">)
            n999 = call-dynamic "Send_String.vi"("error in (no error)"=w2122, "String"="!shuOFF" ("string"), "SpinCoater in"=w2123) -> ("error out"=w2121:errorcluster)  [unwired: 6 in, 2 out]
          }
          frame "Arduino_Shutter_Open" {
            n1000 = Unbundle By Name(w2131) -> ("SpinCoater.lvclass"=w2130:refnum<class "SpinCoater.lvclass">)
            n1001 = call-dynamic "Send_String.vi"("error in (no error)"=w2129, "String"="!shuON" ("string"), "SpinCoater in"=w2130) -> ("error out"=w2128:errorcluster)  [unwired: 6 in, 2 out]
          }
          frame "Measure_Stop" {
            w2140 = T8 {"QueueAction"=enum."TimeOut", "Data"=[], "Data_Raw"=[], "Data_Dark"=[], "Data_Ref"=[], "Device Information"=[], "Numeric Control"=0.0, "Boolean"=FALSE, "Wavelength"=[], "Time"=[], "Time Stamp"=timestamp(0 s since 1904-01-01), "Numeric Control 2"=0.0, "TabControl"=enum."Measure", "Numeric Control 3"=0.0}  # DataQueue
            n1002 = Bundle By Name(cluster=w2140, "QueueAction"=DataQueue_Action."Stop_Measurement") -> (w2141:T8)
            n1003 = Enqueue Element(queue=w2138, element=w2141, error in (no error)=w2135) -> (queue out=w2137:refnum<queue>, error out=w2134:errorcluster)  [unwired: 1 in, 1 out]
          }
          frame "Measure_InSitu" {
            w2182 = T11 {"QueueAction"=enum."TimeOut", "Numeric 1"=0.0, "Numeric 2"=0.0, "Boolean 1"=FALSE, "Boolean 2"=FALSE, "Spin Program"=[], "Spin Prg v07"=[], "Time Stamp"=timestamp(0 s since 1904-01-01), "TabControl"=enum."Measure"}  # Device Queue
            w2189 = T11 {"QueueAction"=enum."TimeOut", "Numeric 1"=0.0, "Numeric 2"=0.0, "Boolean 1"=FALSE, "Boolean 2"=FALSE, "Spin Program"=[], "Spin Prg v07"=[], "Time Stamp"=timestamp(0 s since 1904-01-01), "TabControl"=enum."Measure"}  # Device Queue
            n1004 = Bundle By Name(cluster=w2189, "QueueAction"=DeviceQueue_Action."Spectrometer_SetTriggerMode", "Numeric 1"=1.0) -> (w2187:T11)
            n1005 = Bundle By Name(cluster=w2182, "QueueAction"=DeviceQueue_Action."Spectrometer_DeviceInformation") -> (w2179:T11)
            n1006 = Bundle By Name(cluster=w2179, "QueueAction"=DeviceQueue_Action."Spectrometer_StartMeasurement") -> (w2175:T11)
            n1007 = Enqueue Element(queue=w2188, element=w2187, error in (no error)=w2144) -> (queue out=w2184:refnum<queue>, error out=w2185:errorcluster)  [unwired: 1 in, 1 out]
            n1008 = property on="Frames" class="DigNum (strict)"() -> ("Value"=w2145:i32)  [unwired: 2 in, 2 out]
            n1009 = Bundle By Name(cluster=w2175, "QueueAction"=DeviceQueue_Action."Arduino_StartProgram") -> (w2170:T11)
            n1010 = Enqueue Element(queue=w2184, element=w2179, error in (no error)=w2185) -> (queue out=w2181:refnum<queue>, error out=w2180:errorcluster)  [unwired: 1 in, 1 out]
            n1011 = Bundle By Name(cluster=w2170, "QueueAction"=DeviceQueue_Action."Spectrometer_GetData", "Numeric 1"="Dividider Get Spectra") -> (w2165:T11)
            n1012 = Divide(x=w2145, y="Dividider Get Spectra") -> (x/y=w2177:dbl)
            n1013 = Round Toward +Infinity(x=w2177) -> (ceil(x): smallest int >= x=w2176:dbl)
            n1014 = Enqueue Element(queue=w2181, element=w2175, error in (no error)=w2180) -> (queue out=w2174:refnum<queue>, error out=w2173:errorcluster)  [unwired: 1 in, 1 out]
            n1015 = Enqueue Element(queue=w2174, element=w2170, error in (no error)=w2173) -> (queue out=w2171:refnum<queue>, error out=w2168:errorcluster)  [unwired: 1 in, 1 out]
            n1016 = for {
              N: w2176 -> [_]
              shift-right: [w2192] -> w2167
              shift-left: w2171 -> [w2196]
              tunnel: w2165 -> [w2193]
              shift-right: [w2194] -> w2166
              shift-left: w2168 -> [w2195]
              n1017 = Enqueue Element(queue=w2196, element=w2193, error in (no error)=w2195) -> (queue out=w2192:refnum<queue>, error out=w2194:errorcluster)  [unwired: 1 in, 1 out]
            }
            n1018 = Bundle By Name(cluster=w2165, "QueueAction"=DeviceQueue_Action."Spectrometer_StopMeasurement") -> (w2161:T11)
            n1019 = property on="Measure_FramesSpectrometer" class="DigNum (strict)"() -> ("Value"=w2147:dbl)  [unwired: 2 in, 2 out]
            n1020 = Bundle By Name(cluster=w2161, "QueueAction"=DeviceQueue_Action."Measure_Stop") -> (w2154:T11)
            n1021 = Enqueue Element(queue=w2167, element=w2161, error in (no error)=w2166) -> (queue out=w2162:refnum<queue>, error out=w2163:errorcluster)  [unwired: 1 in, 1 out]
            n1022 = Bundle By Name(cluster=w2154, "QueueAction"=DeviceQueue_Action."Spectrometer_SetTriggerMode", "Numeric 1"=0.0) -> (w2149:T11)
            n1023 = Enqueue Element(queue=w2162, element=w2154, error in (no error)=w2163) -> (queue out=w2157:refnum<queue>, error out=w2158:errorcluster)  [unwired: 1 in, 1 out]
            n1024 = Bundle By Name(cluster=w2149, "QueueAction"=DeviceQueue_Action."Spectrometer_SetFrames", "Numeric 1"=w2147) -> (w2146:T11)
            n1025 = Enqueue Element(queue=w2157, element=w2149, error in (no error)=w2158) -> (queue out=w2156:refnum<queue>, error out=w2155:errorcluster)  [unwired: 1 in, 1 out]
            n1026 = Enqueue Element(queue=w2156, element=w2146, error in (no error)=w2155) -> (queue out=w2150:refnum<queue>, error out=w2151:errorcluster)  [unwired: 1 in, 1 out]
          }
          frame "Measure_InSituAdvanced" {
            w2284 = T11 {"QueueAction"=enum."TimeOut", "Numeric 1"=0.0, "Numeric 2"=0.0, "Boolean 1"=FALSE, "Boolean 2"=FALSE, "Spin Program"=[], "Spin Prg v07"=[], "Time Stamp"=timestamp(0 s since 1904-01-01), "TabControl"=enum."Measure"}  # Device Queue
            n1027 = property on="Dividider Get Spectra" class="DigNum (strict)"() -> ("Value"=w2243:u32)  [unwired: 2 in, 2 out]
            n1028 = Bundle By Name(cluster=w2284, "QueueAction"=DeviceQueue_Action."Spectrometer_SetTriggerMode", "Numeric 1"=1.0) -> (w2239:T11)
            n1029 = Bundle By Name(cluster=w2239, "QueueAction"=DeviceQueue_Action."Spectrometer_DeviceInformation") -> (w2276:T11)
            n1030 = Bundle By Name(cluster=w2276, "QueueAction"=DeviceQueue_Action."Spectrometer_StartMeasurement") -> (w2272:T11)
            n1031 = Enqueue Element(queue=w2283, element=w2239, error in (no error)=w2244) -> (queue out=w2280:refnum<queue>, error out=w2281:errorcluster)  [unwired: 1 in, 1 out]
            n1032 = Bundle By Name(cluster=w2272, "QueueAction"=DeviceQueue_Action."Arduino_StartProgram", "Numeric 1"=1.0) -> (w2267:T11)
            n1033 = property on="Frames" class="DigNum (strict)"() -> ("Value"=w2245:i32)  [unwired: 2 in, 2 out]
            n1034 = Unbundle By Name(w2226) -> ("Time Stamp"=w2225:timestamp)
            n1035 = Enqueue Element(queue=w2280, element=w2276, error in (no error)=w2281) -> (queue out=w2278:refnum<queue>, error out=w2277:errorcluster)  [unwired: 1 in, 1 out]
            n1036 = Divide(x=w2245, y=w2243) -> (x/y=w2274:dbl)
            n1037 = Bundle By Name(cluster=w2267, "QueueAction"=DeviceQueue_Action."Spectrometer_GetData", "Numeric 1"=w2243) -> (w2262:T11)
            n1038 = Round Toward +Infinity(x=w2274) -> (ceil(x): smallest int >= x=w2273:dbl)
            n1039 = Enqueue Element(queue=w2278, element=w2272, error in (no error)=w2277) -> (queue out=w2271:refnum<queue>, error out=w2270:errorcluster)  [unwired: 1 in, 1 out]
            n1040 = Enqueue Element(queue=w2271, element=w2267, error in (no error)=w2270) -> (queue out=w2268:refnum<queue>, error out=w2265:errorcluster)  [unwired: 1 in, 1 out]
            n1041 = Bundle By Name(cluster=w2262, "QueueAction"=DeviceQueue_Action."Spectrometer_StopMeasurement") -> (w2258:T11)
            n1042 = for {
              N: w2273 -> [_]
              shift-right: [w2334] -> w2264
              shift-left: w2268 -> [w2338]
              tunnel: w2262 -> [w2335]
              shift-right: [w2336] -> w2263
              shift-left: w2265 -> [w2337]
              n1043 = Enqueue Element(queue=w2338, element=w2335, error in (no error)=w2337) -> (queue out=w2334:refnum<queue>, error out=w2336:errorcluster)  [unwired: 1 in, 1 out]
            }
            n1044 = property on="Measure_FramesSpectrometer" class="DigNum (strict)"() -> ("Value"=w2246:dbl)  [unwired: 2 in, 2 out]
            n1045 = property on="periodic time" class="DigNum (strict)"() -> ("Value"=w2238:dbl[unit])  [unwired: 2 in, 2 out]
            n1046 = Bundle By Name(cluster=w2258, "QueueAction"=DeviceQueue_Action."Measure_Stop") -> (w2251:T11)
            n1047 = property on="Duration after" class="DigNum (strict)"() -> ("Value"=w2237:dbl[unit])  [unwired: 2 in, 2 out]
            n1048 = node(w2238) -> (w2208:dbl)
            n1049 = property on="periodic time" class="DigNum (strict)"() -> ("Value"=w2236:dbl[unit])  [unwired: 2 in, 2 out]
            n1050 = Bundle By Name(cluster=w2251, "QueueAction"=DeviceQueue_Action."Spectrometer_SetTriggerMode", "Numeric 1"=0.0) -> (w2248:T11)
            n1051 = Enqueue Element(queue=w2264, element=w2258, error in (no error)=w2263) -> (queue out=w2259:refnum<queue>, error out=w2260:errorcluster)  [unwired: 1 in, 1 out]
            n1052 = node(w2237) -> (w2231:dbl)
            n1053 = Bundle By Name(cluster=w2248, "QueueAction"=DeviceQueue_Action."Spectrometer_SetFrames", "Numeric 1"=w2246) -> (w2228:T11)
            n1054 = Enqueue Element(queue=w2259, element=w2251, error in (no error)=w2260) -> (queue out=w2254:refnum<queue>, error out=w2255:errorcluster)  [unwired: 1 in, 1 out]
            n1055 = node(w2236) -> (w2230:dbl)
            n1056 = Bundle By Name(cluster=w2228, "QueueAction"=DeviceQueue_Action."Wait", "Numeric 1"=w2208) -> (w2210:T11)
            n1057 = Enqueue Element(queue=w2254, element=w2248, error in (no error)=w2255) -> (queue out=w2253:refnum<queue>, error out=w2252:errorcluster)  [unwired: 1 in, 1 out]
            n1058 = Not Equal To 0?(x=w2230) -> (x != 0?=w2234:bool)
            n1059 = Not Equal To 0?(x=w2231) -> (x != 0?=w2235:bool)
            n1060 = Divide(x=w2231, y=w2230) -> (x/y=w2232:dbl)
            n1061 = Bundle By Name(cluster=w2210, "QueueAction"=DeviceQueue_Action."Spectrometer_MeasureAdvanced", "Time Stamp"=w2225) -> (w2209:T11)
            n1062 = And(x=w2235, y=w2234) -> (x .and. y?=w2233:bool)
            n1063 = Round Toward +Infinity(x=w2232) -> (ceil(x): smallest int >= x=w2229:dbl)
            n1064 = Enqueue Element(queue=w2253, element=w2228, error in (no error)=w2252) -> (queue out=w2242:refnum<queue>, error out=w2241:errorcluster)  [unwired: 1 in, 1 out]
            n1065 = Bundle By Name(cluster=w2209, "QueueAction"=DeviceQueue_Action."Arduino_SetSpeed", "Numeric 1"=1500.0) -> (w2220:T11)
            n1066 = Bundle By Name(cluster=w2220, "Numeric 1"=0.0) -> (w2212:T11)
            n1067 = property on="Measure_FrameRate" class="DigNum (strict)"() -> ("Value"=w2217:dbl[unit])  [unwired: 2 in, 2 out]
            n1068 = property on="Measure_FramesSpectrometer" class="DigNum (strict)"() -> ("Value"=w2216:dbl)  [unwired: 2 in, 2 out]
            n1069 = Divide(x=w2216, y=w2217) -> (x/y=w2218:dbl[unit])
            n1070 = Bundle By Name(cluster=w2210, "Numeric 1"=1.0) -> (w2213:T11)
            n1071 = node(w2218) -> (w2207:dbl)
            n1072 = Subtract(x=w2208, y=w2207) -> (x-y=w2206:dbl)
            n1073 = Bundle By Name(cluster=w2210, "Numeric 1"=w2206) -> (w2205:T11)
            n1074 = Round Toward +Infinity(x=w2207) -> (ceil(x): smallest int >= x=w2219:dbl)
            n1075 = Add(x=w2219, y=2.0) -> (x+y=w2214:dbl)
            n1076 = Bundle By Name(cluster=w2213, "Numeric 1"=w2214) -> (w2202:T11)
            n1077 = case shown="True" w2233 {
              tunnel: w2242 -> [w2288 w2290]
              tunnel: w2241 -> [w2287 w2293]
              tunnel: w2229 -> [_ w2306]
              tunnel: w2209 -> [_ w2305]
              tunnel: w2205 -> [_ w2301]
              tunnel: w2220 -> [_ w2300]
              tunnel: w2213 -> [_ w2299]
              tunnel: w2209 -> [_ w2298]
              tunnel: w2202 -> [_ w2297]
              tunnel: w2212 -> [_ w2296]
              tunnel: [w2287 w2295] -> w2204
              tunnel: [w2288 w2294] -> w2203
              tunnel: w2210 -> [_ w2289]
              frame False {
              }
              frame True {
                n1078 = Enqueue Element(queue=w2290, element=w2289, error in (no error)=w2293) -> (queue out=w2291:refnum<queue>, error out=w2292:errorcluster)  [unwired: 1 in, 1 out]
                n1079 = for {
                  N: w2306 -> [_]
                  shift-right: [w2327] -> w2303
                  shift-left: w2291 -> [w2333]
                  shift-right: [w2326] -> w2302
                  shift-left: w2292 -> [w2332]
                  tunnel: w2305 -> [w2331]
                  tunnel: w2301 -> [w2328]
                  n1080 = Enqueue Element(queue=w2333, element=w2331, error in (no error)=w2332) -> (queue out=w2329:refnum<queue>, error out=w2330:errorcluster)  [unwired: 1 in, 1 out]
                  n1081 = Enqueue Element(queue=w2329, element=w2328, error in (no error)=w2330) -> (queue out=w2327:refnum<queue>, error out=w2326:errorcluster)  [unwired: 1 in, 1 out]
                }
                n1082 = case shown="True" "Spin at end" {
                  tunnel: w2303 -> [w2308 w2325]
                  tunnel: w2302 -> [w2307 w2324]
                  tunnel: w2300 -> [_ w2319]
                  tunnel: w2299 -> [_ w2318]
                  tunnel: w2298 -> [_ w2317]
                  tunnel: w2297 -> [_ w2312]
                  tunnel: w2296 -> [_ w2311]
                  tunnel: [w2307 w2310] -> w2295
                  tunnel: [w2308 w2309] -> w2294
                  frame False {
                  }
                  frame True {
                    n1083 = Enqueue Element(queue=w2325, element=w2319, error in (no error)=w2324) -> (queue out=w2323:refnum<queue>, error out=w2322:errorcluster)  [unwired: 1 in, 1 out]
                    n1084 = Enqueue Element(queue=w2323, element=w2318, error in (no error)=w2322) -> (queue out=w2321:refnum<queue>, error out=w2320:errorcluster)  [unwired: 1 in, 1 out]
                    n1085 = Enqueue Element(queue=w2321, element=w2317, error in (no error)=w2320) -> (queue out=w2316:refnum<queue>, error out=w2315:errorcluster)  [unwired: 1 in, 1 out]
                    n1086 = Enqueue Element(queue=w2316, element=w2312, error in (no error)=w2315) -> (queue out=w2313:refnum<queue>, error out=w2314:errorcluster)  [unwired: 1 in, 1 out]
                    n1087 = Enqueue Element(queue=w2313, element=w2311, error in (no error)=w2314) -> (queue out=w2309:refnum<queue>, error out=w2310:errorcluster)  [unwired: 1 in, 1 out]
                  }
                }
              }
            }
            n1088 = Bundle By Name(cluster=w2202, "QueueAction"=DeviceQueue_Action."Arduino_Shutter_Close") -> (w2201:T11)
            n1089 = Enqueue Element(queue=w2203, element=w2201, error in (no error)=w2204) -> (queue out=w2199:refnum<queue>, error out=w2198:errorcluster)  [unwired: 1 in, 1 out]
            "Nr After Spin" <- u16 0 ("Nr After Spin")
          }
          frame "Measure_InSituAdvanced_Short" {
            w2387 = T11 {"QueueAction"=enum."TimeOut", "Numeric 1"=0.0, "Numeric 2"=0.0, "Boolean 1"=FALSE, "Boolean 2"=FALSE, "Spin Program"=[], "Spin Prg v07"=[], "Time Stamp"=timestamp(0 s since 1904-01-01), "TabControl"=enum."Measure"}  # Device Queue
            n1090 = property on="Nr After Spin" class="DigNum (strict)"("Value"=u16 0 ("Nr After Spin")) -> ()  [unwired: 2 in, 2 out]
            n1091 = Bundle By Name(cluster=w2387, "QueueAction"=DeviceQueue_Action."Spectrometer_SetTriggerMode", "Numeric 1"=1.0) -> (w2349:T11)
            n1092 = Bundle By Name(cluster=w2349, "QueueAction"=DeviceQueue_Action."Spectrometer_DeviceInformation") -> (w2379:T11)
            n1093 = property on="Frames" class="DigNum (strict)"() -> ("Value"=w2340:i32)  [unwired: 2 in, 2 out]
            n1094 = Bundle By Name(cluster=w2379, "QueueAction"=DeviceQueue_Action."Spectrometer_StartMeasurement") -> (w2377:T11)
            n1095 = Enqueue Element(queue=w2386, element=w2349, error in (no error)=w2350) -> (queue out=w2383:refnum<queue>, error out=w2384:errorcluster)  [unwired: 1 in, 1 out]
            n1096 = Bundle By Name(cluster=w2377, "QueueAction"=DeviceQueue_Action."Arduino_StartProgram", "Numeric 1"=2.0) -> (w2372:T11)
            n1097 = Enqueue Element(queue=w2383, element=w2379, error in (no error)=w2384) -> (queue out=w2381:refnum<queue>, error out=w2380:errorcluster)  [unwired: 1 in, 1 out]
            n1098 = Bundle By Name(cluster=w2372, "QueueAction"=DeviceQueue_Action."Spectrometer_GetData_Short", "Numeric 2"=w2340) -> (w2367:T11)
            n1099 = Enqueue Element(queue=w2381, element=w2377, error in (no error)=w2380) -> (queue out=w2376:refnum<queue>, error out=w2375:errorcluster)  [unwired: 1 in, 1 out]
            n1100 = Enqueue Element(queue=w2376, element=w2372, error in (no error)=w2375) -> (queue out=w2373:refnum<queue>, error out=w2370:errorcluster)  [unwired: 1 in, 1 out]
            n1101 = Bundle By Name(cluster=w2367, "QueueAction"=DeviceQueue_Action."Spectrometer_StopMeasurement") -> (w2363:T11)
            n1102 = property on="Measure_FramesSpectrometer" class="DigNum (strict)"() -> ("Value"=w2351:dbl)  [unwired: 2 in, 2 out]
            n1103 = Enqueue Element(queue=w2373, element=w2367, error in (no error)=w2370) -> (queue out=w2369:refnum<queue>, error out=w2368:errorcluster)  [unwired: 1 in, 1 out]
            n1104 = Bundle By Name(cluster=w2363, "QueueAction"=DeviceQueue_Action."Measure_Stop") -> (w2356:T11)
            n1105 = Bundle By Name(cluster=w2356, "QueueAction"=DeviceQueue_Action."Spectrometer_SetTriggerMode", "Numeric 1"=0.0) -> (w2353:T11)
            n1106 = Enqueue Element(queue=w2369, element=w2363, error in (no error)=w2368) -> (queue out=w2364:refnum<queue>, error out=w2365:errorcluster)  [unwired: 1 in, 1 out]
            n1107 = Bundle By Name(cluster=w2353, "QueueAction"=DeviceQueue_Action."Spectrometer_SetFrames", "Numeric 1"=w2351) -> (w2345:T11)
            n1108 = Enqueue Element(queue=w2364, element=w2356, error in (no error)=w2365) -> (queue out=w2359:refnum<queue>, error out=w2360:errorcluster)  [unwired: 1 in, 1 out]
            n1109 = Enqueue Element(queue=w2359, element=w2353, error in (no error)=w2360) -> (queue out=w2358:refnum<queue>, error out=w2357:errorcluster)  [unwired: 1 in, 1 out]
            n1110 = Enqueue Element(queue=w2358, element=w2345, error in (no error)=w2357) -> (queue out=w2344:refnum<queue>, error out=w2343:errorcluster)  [unwired: 1 in, 1 out]
            n1111 = Bundle By Name(cluster=w2345, "QueueAction"=DeviceQueue_Action."Arduino_Shutter_Close") -> (w2348:T11)
            n1112 = Enqueue Element(queue=w2344, element=w2348, error in (no error)=w2343) -> (queue out=w2346:refnum<queue>, error out=w2339:errorcluster)  [unwired: 1 in, 1 out]
          }
          frame "Measure_Spectrum" {
            n1113 = Unbundle By Name(w2390) -> ("Time Stamp"=w2391:timestamp)
            n1114 = Bundle By Name(cluster=w2390, "QueueAction"=DeviceQueue_Action."Spectrometer_Measure", "Time Stamp"=w2391) -> (w2396:T11)
            n1115 = Bundle By Name(cluster=w2396, "QueueAction"=DeviceQueue_Action."Measure_Stop") -> (w2394:T11)
            n1116 = Enqueue Element(queue=w2402, element=w2396, error in (no error)=w2401) -> (queue out=w2397:refnum<queue>, error out=w2398:errorcluster)  [unwired: 1 in, 1 out]
            n1117 = Enqueue Element(queue=w2397, element=w2394, error in (no error)=w2398) -> (queue out=w2393:refnum<queue>, error out=w2392:errorcluster)  [unwired: 1 in, 1 out]
          }
          frame "Measure_SpectralStability" {
            n1118 = Bundle By Name(cluster=w2406, "QueueAction"=DeviceQueue_Action."Spectrometer_DeviceInformation") -> (w2409:T11)
            n1119 = property on="SpectralStability_\nFrameRate" class="DigNum (strict)"() -> ("Value"=w2429:dbl[unit])  [unwired: 2 in, 2 out]
            n1120 = property on="SpectralStability_\nFramesSpectrometer" class="DigNum (strict)"() -> ("Value"=w2430:dbl)  [unwired: 2 in, 2 out]
            n1121 = Bundle By Name(cluster=w2409, "QueueAction"=DeviceQueue_Action."Spectrometer_Measure") -> (w2408:T11)
            n1122 = Enqueue Element(queue=w2412, element=w2409, error in (no error)=w2411) -> (queue out=w2414:refnum<queue>, error out=w2413:errorcluster)  [unwired: 1 in, 1 out]
            n1123 = Divide(x=w2430, y=w2429) -> (x/y=w2424:dbl[unit])
            n1124 = Unbundle By Name(w2406) -> ("Numeric 1"=w2405:dbl)
            n1125 = Subtract(x="SpectralStability_\nPeriodicTime", y=w2424) -> (x-y=w2423:dbl[unit])
            n1126 = Enqueue Element(queue=w2414, element=w2408, error in (no error)=w2413) -> (queue out=w2428:refnum<queue>, error out=w2427:errorcluster)  [unwired: 1 in, 1 out]
            n1127 = node(w2423) -> (w2422:dbl)
            n1128 = Decrement(x=w2405) -> (x-1=w2404:dbl)
            n1129 = Bundle By Name(cluster=w2408, "QueueAction"=DeviceQueue_Action."Wait", "Numeric 1"=w2422) -> (w2418:T11)
            n1130 = for {
              N: w2404 -> [_]
              shift-right: [w2434] -> w2421
              shift-left: w2428 -> [w2440]
              shift-right: [w2433] -> w2420
              shift-left: w2427 -> [w2439]
              tunnel: w2418 -> [w2436]
              tunnel: w2408 -> [w2435]
              n1131 = Enqueue Element(queue=w2440, element=w2436, error in (no error)=w2439) -> (queue out=w2438:refnum<queue>, error out=w2437:errorcluster)  [unwired: 1 in, 1 out]
              n1132 = Enqueue Element(queue=w2438, element=w2435, error in (no error)=w2437) -> (queue out=w2434:refnum<queue>, error out=w2433:errorcluster)  [unwired: 1 in, 1 out]
            }
            n1133 = Bundle By Name(cluster=w2418, "QueueAction"=DeviceQueue_Action."Measure_Stop") -> (w2417:T11)
            n1134 = Enqueue Element(queue=w2421, element=w2417, error in (no error)=w2420) -> (queue out=w2415:refnum<queue>, error out=w2416:errorcluster)  [unwired: 1 in, 1 out]
          }
        }
      }
      frame Error {
        w2445 = T19 4 items=["no dialog", "OK message", "continue or stop message", "OK message + warnings", "continue/stop + warnings"] ("type of dialog (OK msg:1)")
        n1135 = call <vilib>:"General Error Handler.vi"("type of dialog (OK msg:1)"=w2445, "error in (no error)"=w2446) -> ("error out"=w2444:errorcluster)  [unwired: 9 in, 4 out]
        n1136 = call <vilib>:"Clear Errors.vi"("error in (no error)"=w2444) -> ("error out"=w2443:errorcluster)  [unwired: 5 in, 1 out]
      }
    }
  }
  n1137 = disable-structure shown="Disabled" {
    frame Disabled {
      w2449 = T11 {"QueueAction"=enum."TimeOut", "Numeric 1"=0.0, "Numeric 2"=0.0, "Boolean 1"=FALSE, "Boolean 2"=FALSE, "Spin Program"=[], "Spin Prg v07"=[], "Time Stamp"=timestamp(0 s since 1904-01-01), "TabControl"=enum."Measure"}  # Device Queue
      n1138 = Bundle By Name(cluster=w2449, "QueueAction"=DeviceQueue_Action."Arduino_SetSpeed") -> (w2450:T11)  [unwired: 1 in]
      n1139 = Enqueue Element(element=w2450) -> ()  [unwired: 3 in, 3 out]
    }
    frame Enabled {
    }
  }
  n1140 = Release Queue(queue=w9) -> ()  [unwired: 2 in, 3 out]
  n1141 = Release Queue(queue=w10) -> ()  [unwired: 2 in, 3 out]
